vi "blackfly camera capture v2.1 - laser pointer.vi"() -> ()   [LabVIEW 2020]
uses:
  <vilib>/userDefined/High Color/IMAQdx.ctl
  <vilib>/vision/driver/IMAQdx.llb/IMAQdx Acquisition Mode.ctl
  <vilib>/vision/driver/IMAQdx.llb/IMAQdx Buffer Number Mode.ctl
  <vilib>/DAQmx/write.llb/DAQmx Write (Analog Wfm 1Chan NSamp).vi
  <vilib>/DAQmx/read.llb/DAQmx Read (Analog DBL 1Chan 1Samp).vi
  <extravilib>/ChannelInstances/Stream-a[.](u8)/Read With Abort.vi
  <extravilib>/ChannelInstances/Stream-a[.](u8)/Write With Abort.vi
  <extravilib>/ChannelInstances/Stream-a[.](u8)/EndpointRead.vi
  <extravilib>/ChannelInstances/Stream-a[.](u8)/Endpoint.vi
  <vilib>/DAQmx/create/channels.llb/DAQmx Create Channel (AO-Voltage-Basic).vi
  <vilib>/DAQmx/configure/timing.llb/DAQmx Timing (Sample Clock).vi
  <vilib>/DAQmx/create/channels.llb/DAQmx Create Channel (AI-Voltage-Basic).vi
  <vilib>/DAQmx/miscellaneous.llb/DAQmx Fill In Error Info.vi
  <extravilib>/ChannelInstances/Stream-a[.](u8)/Instantiate.vi
  <extravilib>/ChannelInstances/Stream-a[.](u8)/)Channel.vi
  <resource>/ChannelSupport/_ChannelSupport/WaitIfNeeded.vi
  <vilib>/vision/driver/NI_Vision_Acquisition_Software.lvlib
  <resource>/objmgr/imaqdx.rc
  <vilib>/Analysis/NI_AALPro.lvlib
  <vilib>/Analysis/NI_AALBase.lvlib
  <instrlib>/Tektronix AFG 1000 Series/Tektronix AFG 1000 Series.lvlib
  <extravilib>/ChannelInstances/Stream-a[.](u8).lvlib
  <resource>/objmgr/daqmx.rc
  <vilib>/measure/NI_MABase.lvlib
  Lab View projects/Tektronix DC Power Supply Interface/Tektronix PWS4XXX Series/Tektronix PWS4XXX Series.lvlib
panel:
  in  "prog 2 v arr":dbl[](array[numeric])=[0.0, 1.2, 1.4, 1.6, 1.6, 1.4, 1.2]
  in  "v time p2":dbl=20.0
  out "prog 2 step":dbl
  in  "Program 2":bool
  in  "move on click":bool
  in  "de-init time":dbl=10.0
  in  "v time":dbl=40.0
  in  "init time":dbl=10.0
  out "prog1 step":dbl
  in  "Program 1":bool
  in  "AOBD MIN":dbl=2.4
  in  "AOBD MAX":dbl=4.0
  out "Global Rectangle":i32[](array[numeric])
  out "Image":T1(plugin-control)
  in  "AOBD GO":bool
  in  "AOBD W":dbl=0.001 min=0.0 max=3.0 step=0.1
  in  "AOBD Y":dbl=3.2
  in  "AOBD X":dbl=3.2
  in  "Partial P. Ref.":string(combo)="70 nm Au"
  out "All data log refnum":refnum<file>
  out "laer volts refnum":refnum<file>
  out "Laser mW renum":refnum<file>
  in  "V limit":dbl=3.0
  in  "Laser On/Off":bool
  in  "Current (A)":dbl
  in  "Laser Volts (V)":dbl=0.3 min=0.0 max=5.0 step=0.1
  out "nm/pixel\n(binned)":dbl
  in  "nm/pixel\n(native)":dbl=67.5
  in  "2x binning":bool=TRUE
  out "offsety":dbl
  out "offsetx":dbl
  in  "Camera pixels":string(combo)="256"
  in  "Ratio Buffer Size":i32=20
  in  "Dynamic Range":dbl=0.03 step=0.01
  in  "Ratiometric?":bool
  in  "Tab Control - Record Save":enum32{"Page 1", "Page 2"}(tab)
  out "red":bool
  out "yellow":bool
  in  "Experiment Name":string="test code"
  in  "Experiment Notes":string="8ul NaH2PO4\n8ul sample\n75nm Au Partial Reflector"
  in  "SAVE RAW IMAGE":bool
  in  "RECORD / STOP VIDEO":bool
  in  "Copy Notes To Log":bool
  in  "FOV (um)":dbl
  out "second":i32
  out "minute":i32
  out "recorded fps":dbl
  out "Y":dbl
  out "X":dbl
  in  "Base Path":path=path "C:/Users/Matt/Desktop/ISCAT EXPERIMENTS"
  out "Date":string
  out "Record Step":u8
  out "record start time":dbl format="%_19f"
  in  "Save Raw Binary":bool=TRUE
  in  "Save Feed Binary":bool
  in  "Clear Log":bool
  in  "Save Experiment Log":bool
  out "Experiment Log":string
  out "Camera Status":string
  in  "Refresh":bool
  out "copy buffer":bool
  out "noise":dbl format="%0.7f"
  in  "get noise":bool
  in  "Paste Buffer":bool
  in  "Copy Buffer":bool
  out "XY Graph 2":cluster{dbl[], "element":u8[]}(graph)
  in  "V":dbl(slide) scale=-1.5..1.5
  in  "signal type":T2(ring)
  in  "Laser Zoom Level":T3(radio)=enum."Radio Selection 3"
  in  "Record\nVoltage?":bool=TRUE
  out "EPD Voltage":dbl format="%0.2f"
  out "Waveform Graph":waveform(dbl)(graph)
  in  "Amplitude (V)":dbl=1.0
  in  "Frequency (hz)":dbl=0.1
  in  "Offset (V)":dbl
  in  "phase (°)":dbl
  in  "EPD Voltage set":dbl=1.2 step=0.1
  in  "AC":bool
  in  "EPD-DC Power":bool
  out "Main Intensity":dbl[][](graph)
  in  "Camera Zoom Level - DEPRECATED":T4(radio)
  in  "conc.":string
  in  "set sample name":bool
  in  "pH":string="7"
  in  "Size":string="50"
  in  "Material":string(combo)="PS"
  in  "Coverslip":string(combo)="ITO dc 70-100 ohm - no bb"
  in  "Laser Current":dbl=500.0
  in  "Laser Power":dbl=5.0
  out "Laser Temp":u8(slide) scale=20.0..50.0
  out "PSU Temp":u8(slide) scale=20.0..50.0
  out "Laser PSUType":u16(ring)=3 items=["FPU", "MPC6000", "MPC3000", "SMD12"]
  out "Laser COM Port":refnum<visa-resource-name>="COM6"
  in  "Set Laser Power":bool
  in  "Set Power (mW)":dbl=150.0
  in  "Green Laser":bool
  in  "stop":bool
  out "Histogram Graph 2":T5(graph)
  in  "Extras":T6(tab)
  out "live print map":dbl[][](graph)
  out "resampled image":u8[][](graph)
  out "aobd y":dbl
  out "aobd x":dbl
  out "volts on?":bool
  out "applied volts":dbl
  in  "reset print image button":bool
  in  "print image button":bool
  out "timer value":dbl
  out "initialized array":dbl[][](array[numeric])
  out "x":i32
  out "y":i32
  out "pixel value":dbl
  in  "exposure time":dbl(slide)=1000.0 scale=0.0..10000.0
  in  "aobd max":dbl=4.2
  in  "aobd min":dbl=2.2
  in  "set volts":dbl=1.0
  in  "output resolution":dbl=4.0
  in  "load image button":bool
  out "Raw binfile refnum":refnum<file>
  out "Text File refnum":refnum<file>
  out "Feed binfile refnum":refnum<file>
  out "text file path":string
  out "feed file path":string
  out "raw file path":string
  out "image file path":string
  out "Laser Status Update Timer":u32
  out "fps 2":dbl(graph)
  out "raw feed":u8[][](graph)
  out "t1":dbl format="%_19f"
  out "t2":dbl format="%_19f"
  out "rt":dbl
  out "rt 2":dbl
  out "zoom array":i32[](array[numeric])
  out "FOV array":i32[](array[numeric])
  out "FunGen Amp Array":dbl[](array[numeric])
  out "EPD Voltage Log refnum":refnum<file>
  out "Voltage Log file Path":string
  in  "Tab Control 3":T7(tab)
  out "frame rate warning":bool
  in  "900 fps":bool
  in  "600 fps":bool
  in  "500 fps":bool
  in  "200 fps":bool
  out "Gain Warning":bool
  out "sync exp warning":bool
  in  "Exposure Time (us)":dbl(slide)=676.6766570605188 scale=4.4..10000.0
  in  "Frame Rate (hz)":dbl(slide) scale=0.0..1000.0
  in  "Gain (dB)":dbl(slide) scale=0.0..47.9
  out "frame rate":dbl
  out "exp time":dbl=1.0
  out "Gain (dB)":dbl
  out "sync exp":dbl
  out "Ratio Stack 1":dbl[][](array[numeric])
  out "Boolean":bool
  out "Ratio Stack 2":dbl[][](array[numeric])
  out "Boolean 2":bool
  out "max value":dbl
  out "min value":dbl
  out "Histogram Graph":T5(graph)
  out "loading ratiometric":dbl
  out "loading ratiometric stack":bool
  out "queue2 save":cluster{dbl[][]}[](array[cluster])
  out "# elements in queue":i32
  out "Numeric":i32
  out "# elements in queue 2":i32
  out "size(s)":i32
  out "queue1 save":cluster{dbl[][]}[](array[cluster])
  in  "get camera info":bool
  out "AcquisitionMode":dbl
  out "AcquisitionFrameRateEnable":dbl
  out "ExposureMode":dbl
  out "Line Selector":dbl
  out "Line Mode":dbl
  out "Line Inverter":dbl
  out "Gain Auto":dbl
  out "binning vertical":dbl
  out "binning horizontal":dbl
  out "height":dbl
  out "width":dbl
  in  "Auto Exposure":string(combo)
  in  "Auto Framerate":string(combo)
  in  "Auto Gain":string(combo)
  in  "Manual Framerate Enabled?":bool
  out "Buffer Number Out":u32
  out "bg array":dbl[][](array[numeric])
  in  "bg array sum":dbl[][](array[numeric])
  out "bg timer":u32
  out "n bg frames":i32
  out "bg countdown":dbl format="%#_2f"
  in  "acquire bg":bool
  in  "apply bg removal":bool
  out "acquiring bg":bool
  # "was 74"
  # "was 37"
  # "nm"
  # "send to NI voltage card"
  # "send to function generator"
  # "I should just remove this \"feature\""
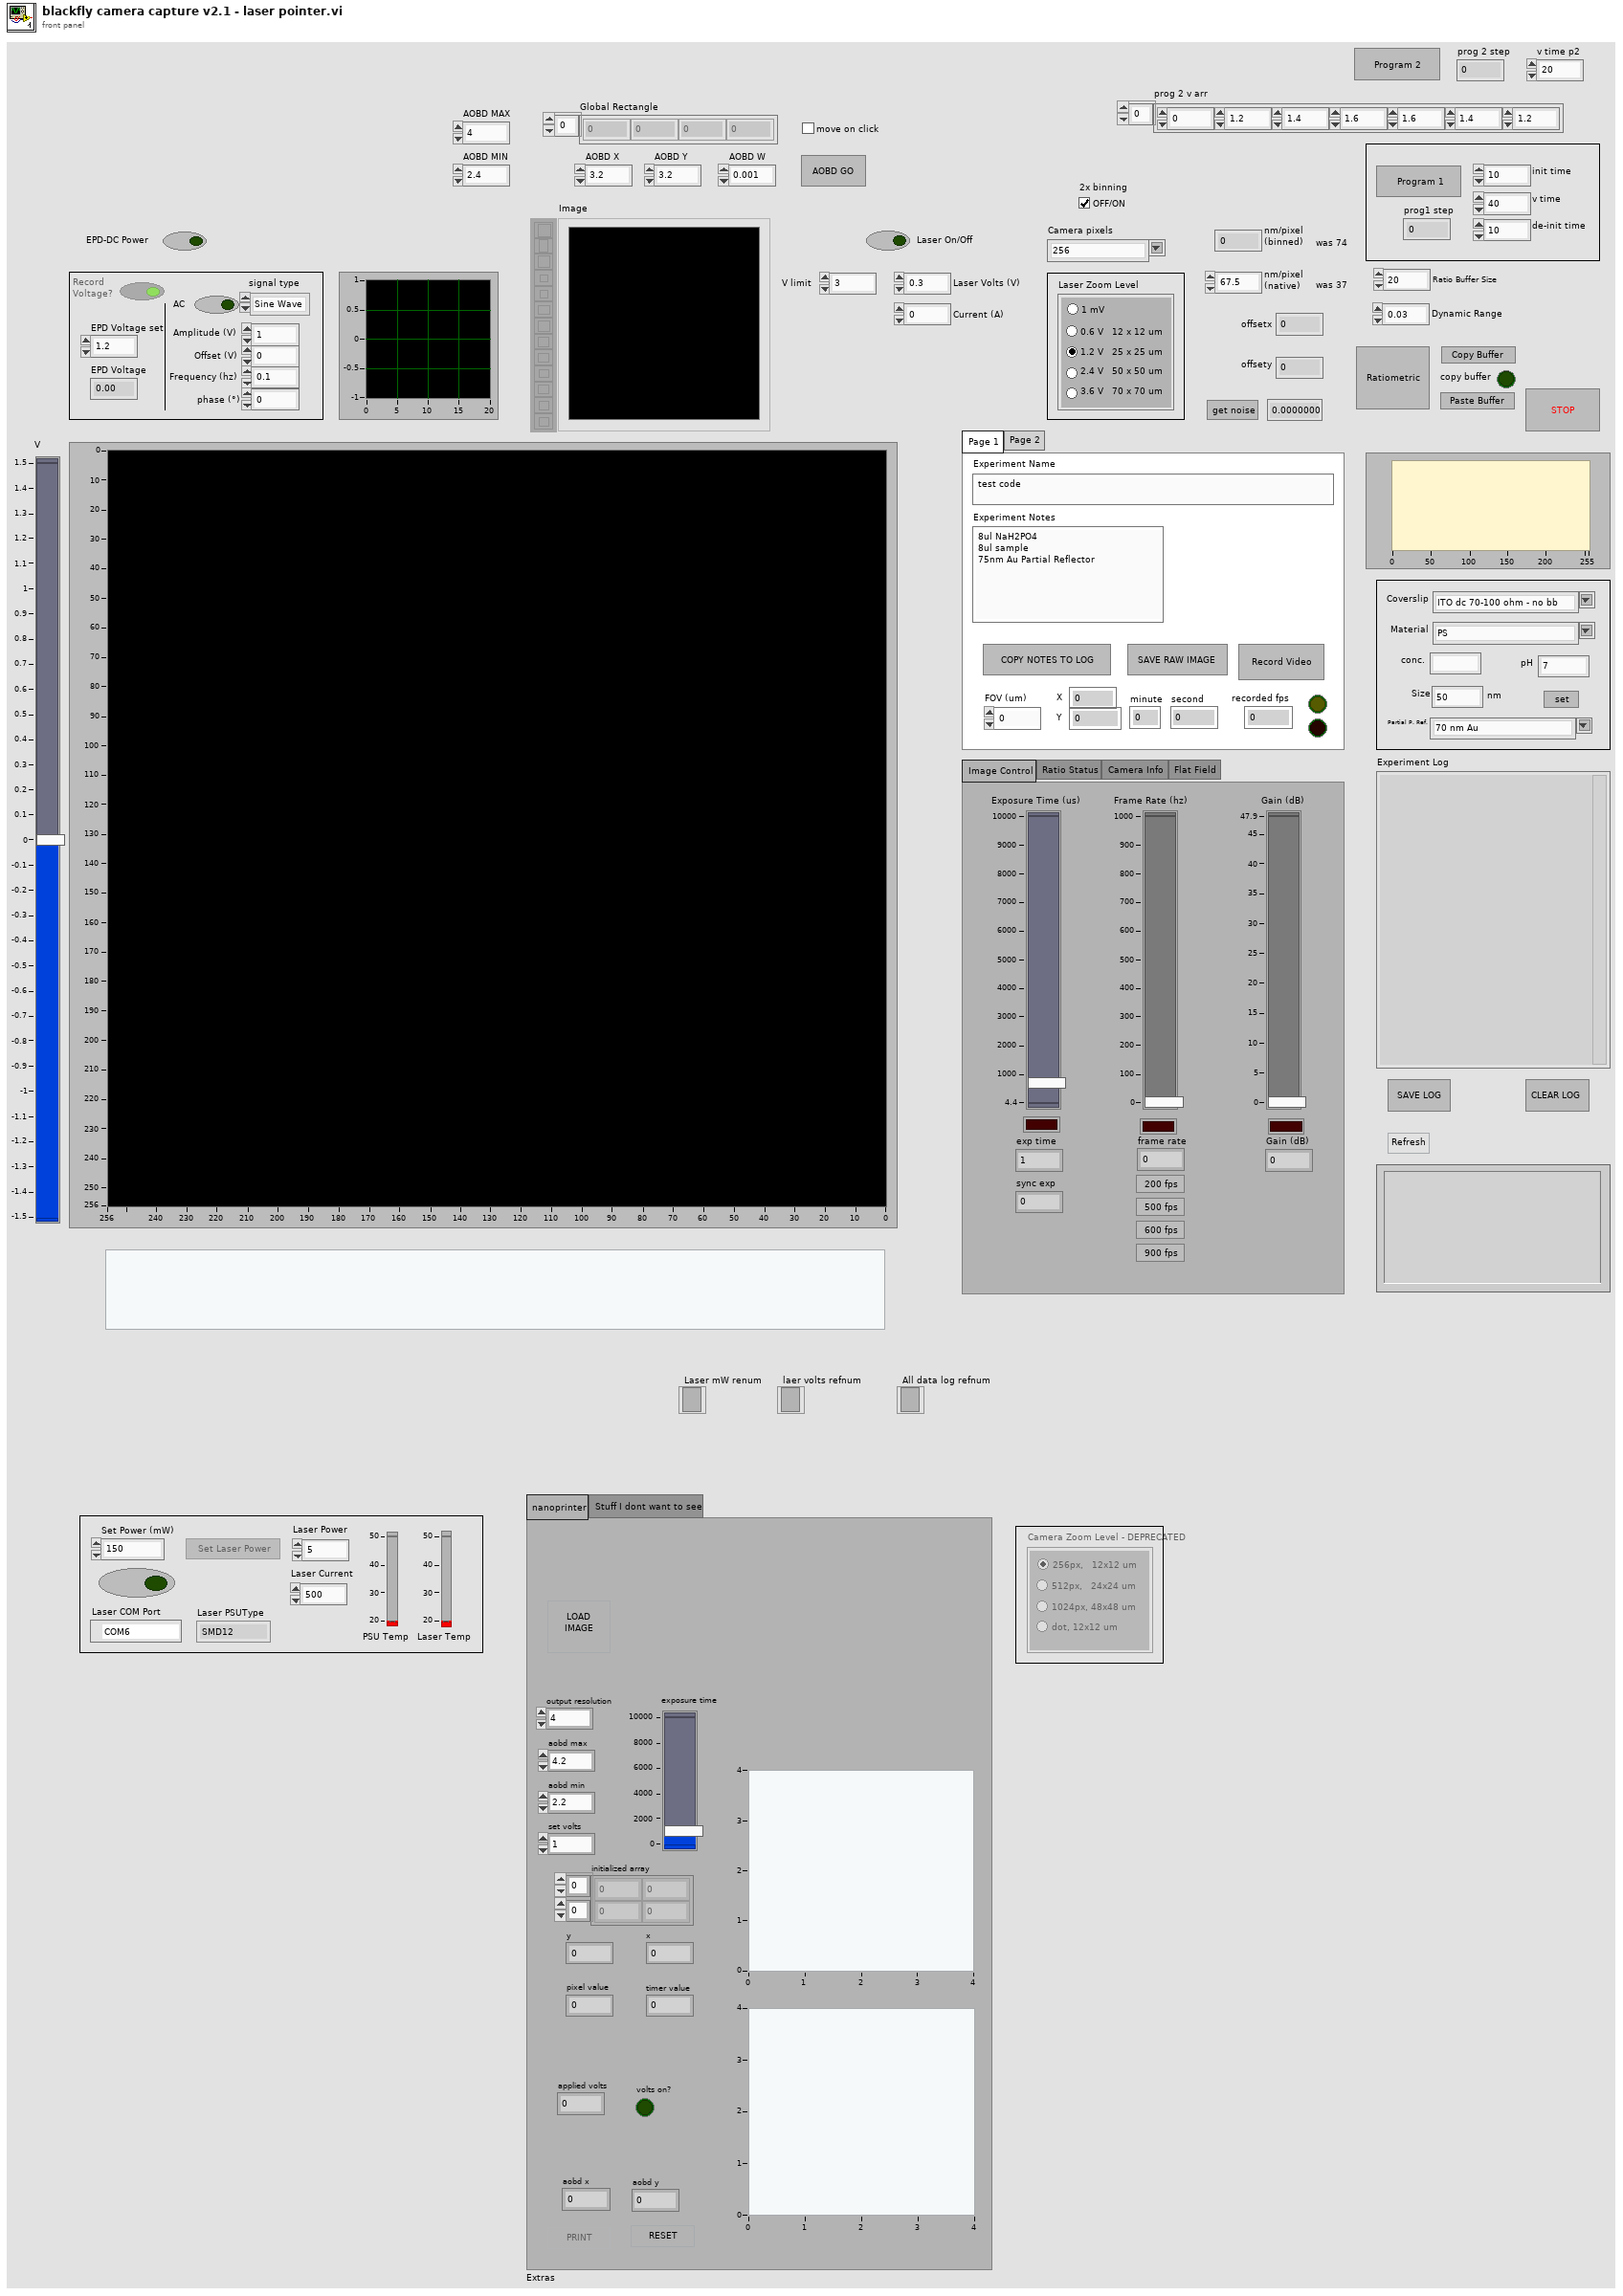
[diagram p1: front panel]
types:
  T1 = typedef "IMAQ Image.ctl" = refnum<image>
  T2 = enum16{"Sine Wave", "Triangle Wave", "Square Wave", "Sawtooth Wave"}
  T3 = enum32{"Radio Selection 1", "Radio Selection 2", "Radio Selection 3", "Radio Selection 4", "Radio Selection 5"}
  T4 = enum32{"256px,   12x12 um", "512px,   24x24 um", "1024px, 48x48 um", "dot, 12x12 um"}
  T5 = cluster{"X Values":dbl[], "Histogram: h(x)":i32[]}
  T6 = enum32{"nanoprinter", "Stuff I dont want to see"}
  T7 = enum32{"Image Control", "Ratio Status", "Camera Info", "Flat Field"}
  T8 = typedef "IMAQdx.ctl" = refnum<k21>
  T9 = enum8{"Enabled", "Disabled", "Disabled and Grayed Out"}
  T10 = typedef "NI_Vision_Acquisition_Software.lvlib/IMAQdx Acquisition Mode.ctl" = enum32{"One Shot", "Continuous"}
  T11 = typedef "NI_Vision_Acquisition_Software.lvlib/IMAQdx Buffer Number Mode.ctl" = enum32{"Next", "Last", "Buffer Number", "Every", "Last New"}
  T12 = cluster{string, "ValueDBL":dbl, string, "ValueDBL":dbl, string, "ValueDBL":dbl, string, "ValueDBL":dbl, "ValueDBL":dbl, "ValueDBL":dbl, "ValueDBL":dbl, "ValueDBL":dbl, "ValueDBL":dbl, "ValueDBL":dbl}
  T13 = cluster{"Global Rectangle":i32[], "Contours":cluster{"Contour Type":u32, "ROI Type":u32, "Points":i32[]}[]}
  T14 = typedef "Stream-a[.](u8).lvlib/)Channel.ctl" = refnum<queue>
  T15 = typedef "LVDateTimeRec.ctl" = cluster{"fractional second":dbl, "second":i32, "minute":i32, "hour":i32, "day of month":i32, "month":i32, "year":i32, "day of week":i32, "day of year":i32, "DST":i32}
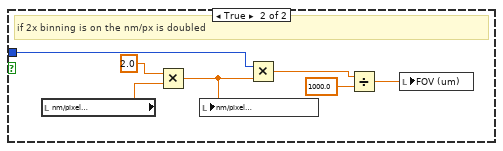
[diagram p2: hidden frame]
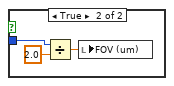
[diagram p3: hidden frame]
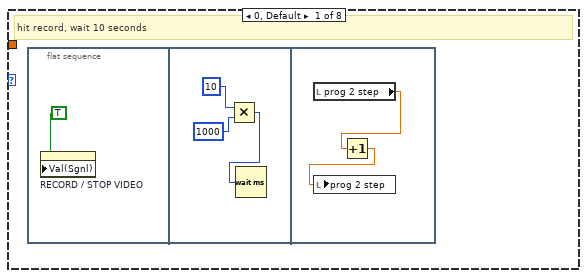
[diagram p11: hidden frame]
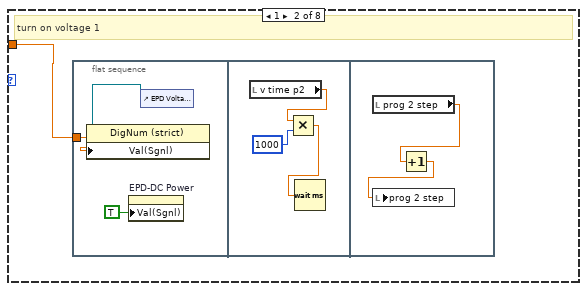
[diagram p12: hidden frame]
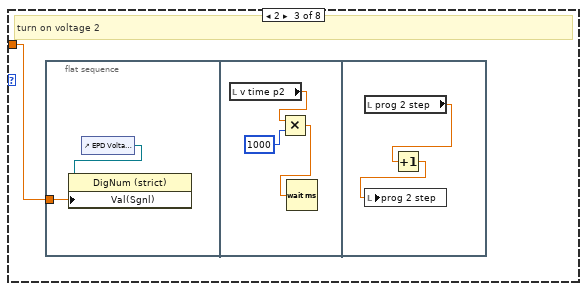
[diagram p13: hidden frame]
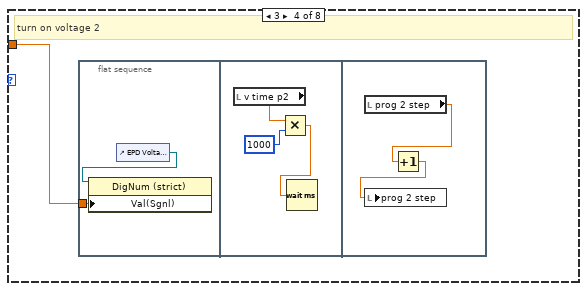
[diagram p14: hidden frame]
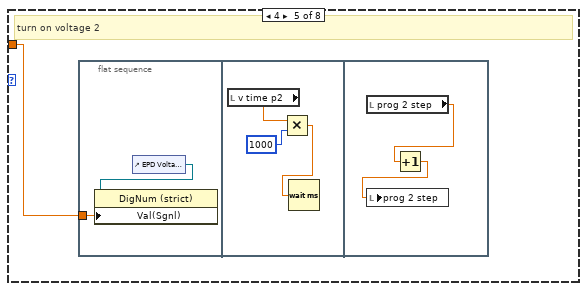
[diagram p15: hidden frame]
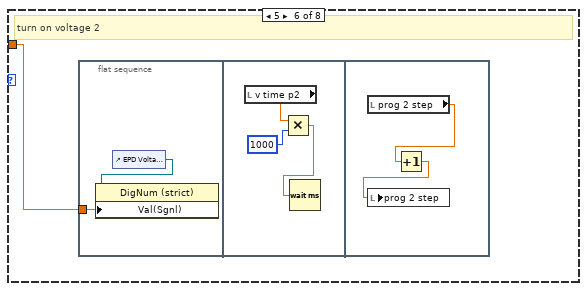
[diagram p16: hidden frame]
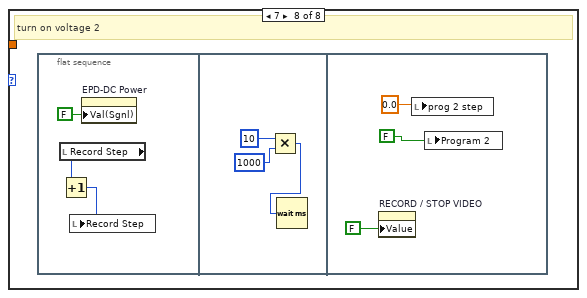
[diagram p17: hidden frame]
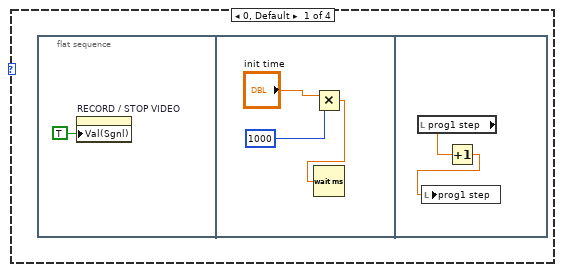
[diagram p19: hidden frame]
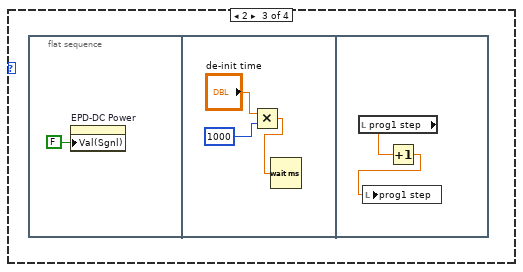
[diagram p20: hidden frame]
diagram:
  n1 = flat-sequence {
    tunnel: [w63] -> w38
    tunnel: [w53] -> w24
    tunnel: [w52] -> w23
    tunnel: [w47] -> w20
    tunnel: [w42] -> w14
    tunnel: [w40] -> w6
    tunnel: [w39] -> w3
    tunnel: w38 -> [w272]
    tunnel: [w275] -> w37
    tunnel: [w272] -> w35
    tunnel: [w273] -> w34
    tunnel: [w259] -> w30
    tunnel: [w258] -> w29
    tunnel: w24 -> [w164]
    tunnel: w23 -> [w163]
    tunnel: [w229] -> w22
    tunnel: w20 -> [w229]
    tunnel: [w197] -> w19
    tunnel: [w196] -> w17
    tunnel: [w195] -> w16
    tunnel: w14 -> [w194]
    tunnel: [w193] -> w13
    tunnel: [w187] -> w11
    tunnel: [w186] -> w10
    tunnel: w6 -> [w72]
    tunnel: [w72] -> w5
    tunnel: w3 -> [w71]
    tunnel: [w71] -> w2
    tunnel: w37 -> [w404]
    tunnel: [w400] -> w36
    tunnel: w35 -> [w400]
    tunnel: w34 -> [w405]
    tunnel: [w403] -> w33
    tunnel: [w402] -> w32
    tunnel: [w406] -> w31
    tunnel: w30 -> [w398]
    tunnel: w29 -> [w397]
    tunnel: [w396] -> w28
    tunnel: [w395] -> w27
    tunnel: [w394] -> w26
    tunnel: [w393] -> w25
    tunnel: w22 -> [w380]
    tunnel: [w399] -> w21
    tunnel: w19 -> [w391]
    tunnel: [w390] -> w18
    tunnel: w17 -> [w389]
    tunnel: w16 -> [w388]
    tunnel: [w387] -> w15
    tunnel: w13 -> [w386]
    tunnel: [w385] -> w12
    tunnel: w11 -> [w384]
    tunnel: w10 -> [w383]
    tunnel: [w382] -> w9
    tunnel: [w381] -> w8
    tunnel: [w379] -> w7
    tunnel: w5 -> [w377]
    tunnel: [w377] -> w4
    tunnel: w2 -> [w376]
    tunnel: [w375] -> w1
    tunnel: w36 -> [w2026]
    tunnel: w33 -> [w2034]
    tunnel: w32 -> [w2027]
    tunnel: w31 -> [w2016]
    tunnel: w28 -> [w2023]
    tunnel: w27 -> [w2022]
    tunnel: w26 -> [w2019]
    tunnel: w25 -> [w2018]
    tunnel: w21 -> [w2015]
    tunnel: w18 -> [w2013]
    tunnel: w15 -> [w2003]
    tunnel: w12 -> [w2002]
    tunnel: w9 -> [w2000]
    tunnel: w8 -> [w1999]
    tunnel: w7 -> [w1991]
    tunnel: w4 -> [w1990]
    tunnel: w1 -> [w1989]
    frame #0 {
      # "Lasertack Laser Controls\n\nTektronix PWS4721 Programmable\nDC Power Supply 0-72V, 1.2A"
      # "FUNCTION GENERATOR FOR ITO EXPERIMENTS"
      # "Function Generator Controls"
      # "BINARY VIDEO SAVING"
      # "Reset Default Controls Upon Start-Up"
      # "Video Feed Circular Buffer Initialization"
      # "MAIN CONTROLS"
      # "Camera Feed Controls"
      # "Initialization 1"
      n2 = control-ref of="This VI"() -> (w58:refnum<vi>)
      n3 = Multiply(x="Ratio Buffer Size", y=2) -> (x*y=w61:i32)
      n4 = Add(x=w61, y=10.0) -> (x+y=w64:dbl)
      n5 = invoke class="VI" method="Default Vals.Reinit All"(reference=w58) -> ()  [unwired: 2 in, 3 out]
      n6 = call <instrlib>:"Initialize.vi"("Reset (True)"=FALSE, "VISA resource name"=refnum<visa-resource-name> "USB0::0x0699::0x0353::2002170::INSTR") -> ("error out"=w42:errorcluster, "VISA resource name out"=w47:refnum<visa-resource-name>)  [unwired: 8 in]
      n7 = for {
        N: w64 -> [_]
        tunnel: [w66] -> w63 mode=indexing
        tunnel: [w65] -> w57
        i -> [w70]
        # "Allocate Buffer Memory"
        n8 = Format Into String(format string="Buffer ID %d", w70) -> (resulting string=w68:string)  [unwired: 2 in, 1 out]
        n9 = call "IMAQ Create"("Border Size"=0, "Image Name"=w68) -> ("New Image"=w66:T1, "error out"=w65:errorcluster)  [unwired: 3 in]
      }
      n10 = call <instrlib>:"Initialize.vi"("VISA resource name"=refnum<visa-resource-name> "USB0::0x0699::0x0394::C010244::INSTR") -> ("error out"=w39:errorcluster, "VISA resource name out"=w40:refnum<visa-resource-name>)  [unwired: 9 in]
      n11 = property on="Main Intensity" class="IntGraph (strict)"("ZScale.Maximum"=255.0 ("Z Scale.Range:Maximum"), "ZScale.Minimum"=0.0 ("Z Scale.Range:Minimum")) -> ()  [unwired: 2 in, 2 out]
      n12 = property on="Main Intensity" class="IntGraph (strict)"("XScale.Minimum"=0.0 ("Z Scale.Range:Maximum"), "YScale.Minimum"=0.0 ("Z Scale.Range:Minimum"), "XScale.Maximum"=512.0 ("Y Scale.Range:Minimum"), "YScale.Maximum"=512.0 ("Y Scale.Range:Minimum")) -> ()  [unwired: 2 in, 2 out]
      n13 = call <vilib>:"IMAQdx Open Camera.vi"("error in"=w57, "Session In"=T8 "blackfly") -> ("error out"=w53:errorcluster, "Session Out"=w52:T8)  [unwired: 8 in]
      "rt" <- 0.0 ("rt")
      "rt 2" <- 0.0 ("rt")
    }
    frame #1 {
      w83 = "\t"
      w81 = "\r\n"
      w80 = 2.0 ("ValueDBL")
      w126 = u32 256 ("Height")
      w127 = u32 256 ("Width")
      w213 = 10123 items=["Finite Samples"=10178, "Continuous Samples"=10123, "Hardware Timed Single Point"=12522] ("sample mode")
      w216 = 10123 items=["Finite Samples"=10178, "Continuous Samples"=10123, "Hardware Timed Single Point"=12522] ("sample mode")
      # "READ VOLTAGE CHANNEL"
      # "ANALOG VOLTAGE OUTPUT CHANNEL"
      # "Initialization 2"
      n14 = local read "Camera Zoom Level - DEPRECATED"() -> (w228:T4)
      n15 = property class="IMAQdx"(reference=w163, error in=w164, "OffsetX"=u32 0, "OffsetY"=u32 0) -> (reference out=w147:T8, error out=w146:errorcluster)
      n16 = disable-structure shown="Disabled" {
        frame Disabled {
          w294 = u16 3 items=["FPU", "MPC6000", "MPC3000", "SMD12"] ("PSUType")
          n17 = Tick Count (ms)() -> (millisecond timer value=→"Laser Status Update Timer":u32)
          "Laser COM Port" <- refnum<visa-resource-name> "COM6" ("LQComm Resource In")
          "Laser PSUType" <- w294
        }
        frame Enabled {
        }
      }
      n18 = disable-structure shown="Disabled" {
        disable-tunnel: _ -> [w343 _]
        disable-tunnel: [w342 _] -> _
        frame Disabled {
          n19 = property class="IMAQdx"(reference=w343, "ActiveAttribute"="CameraAttributes::ImageFormatControl::VideoMode", "ValueDBL"=2.0) -> (reference out=w342:T8)  [unwired: 1 in, 1 out]
        }
        frame Enabled {
        }
      }
      n20 = local read "FOV array"() -> (w239:i32[])
      n21 = local read "Laser Zoom Level"() -> (w143:T3)
      n22 = local read "2x binning"() -> (w79:bool)
      n23 = Build Array(0.75 ("dimension size"), 1.5 ("dimension size"), 3.0 ("dimension size"), 0.001 ("element")) -> (→"FunGen Amp Array":dbl[])
      n24 = Index Array(array=w239, index=w228) -> (element=w78:i32)
      n25 = Build Array(256 ("dimension size"), 512 ("dimension size"), 1024 ("dimension size"), 256 ("element")) -> (→"zoom array":i32[])
      n26 = Build Array(9 ("dimension size"), 18 ("dimension size"), 36 ("dimension size"), 9 ("element")) -> (→"FOV array":i32[])
      n27 = call-poly <vilib>:"DAQmx Create Virtual Channel.vi"("maximum value"=10.0, "minimum value"=-10.0, "physical channels"=tag "Dev1/ao0", "name to assign"="Channel 1 V_out") -> ("task out"=w215:refnum<k21>, "error out"=w190:errorcluster)  [unwired: 10 in]
      n28 = case shown="False" w79 {
        tunnel: w78 -> [w289 w290]
        frame False {
          n29 = local write "FOV (um)"(w289) -> ()
        }
        frame True {
          n30 = Divide(x=w290, y=2.0) -> (x/y=w291:dbl)
          n31 = local write "FOV (um)"(w291) -> ()
        }
      }
      n32 = local read "zoom array"() -> (w238:i32[])
      n33 = flat-sequence "Recall Function Generator Settings" {
        tunnel: [w351] -> w180
        tunnel: w229 -> [w350]
        tunnel: [u32 200 ("milliseconds to wait")] -> w178
        tunnel: w143 -> [w349]
        tunnel: [w348] -> w176
        tunnel: w194 -> [w347]
        tunnel: w180 -> [w355]
        tunnel: [w355] -> w179
        tunnel: w178 -> [w353]
        tunnel: [w353] -> w177
        tunnel: w176 -> [w354]
        tunnel: [w354] -> w175
        tunnel: [w360] -> w185
        tunnel: w179 -> [w359]
        tunnel: w177 -> [w358]
        tunnel: [w358] -> w183
        tunnel: w175 -> [w357]
        tunnel: [w356] -> w182
        tunnel: w185 -> [w365]
        tunnel: [w365] -> w184
        tunnel: w183 -> [w363]
        tunnel: w182 -> [w364]
        tunnel: [w364] -> w181
        tunnel: w184 -> [w368]
        tunnel: w181 -> [w367]
        tunnel: [w366] -> w193
        frame #0 {
          w352 = u16 0 items=["Recall", "Save"] ("Operation (0: Recall)")
          n34 = call <instrlib>:"Recall Save Instrument Settings.vi"("error in (no error)"=w347, "Setup Memory Location (0)"=w349, "Operation (0: Recall)"=w352, "VISA resource name"=w350) -> ("error out"=w348:errorcluster, "VISA resource name out"=w351:refnum<visa-resource-name>)  [unwired: 6 in]
        }
        frame #1 {
          n35 = Wait (ms)(milliseconds to wait=w353) -> ()  [unwired: 1 out]
        }
        frame #2 {
          w361 = u16 1 items=["Channel 1"=1, "Channel2"=2] ("Channel (1: Channel 1)")
          n36 = call <instrlib>:"Enable Output.vi"("Enable Output (T: Enable)"=TRUE, "error in (no error)"=w357, "Channel (1: Channel 1)"=w361, "VISA resource name"=w359) -> ("error out"=w356:errorcluster, "VISA resource name out"=w360:refnum<visa-resource-name>)  [unwired: 6 in]
        }
        frame #3 {
          n37 = Wait (ms)(milliseconds to wait=w363) -> ()  [unwired: 1 out]
        }
        frame #4 {
          w369 = u16 2 items=["Channel 1"=1, "Channel2"=2] ("Channel (1: Channel 1)")
          n38 = call <instrlib>:"Enable Output.vi"("Enable Output (T: Enable)"=TRUE, "error in (no error)"=w367, "Channel (1: Channel 1)"=w369, "VISA resource name"=w368) -> ("error out"=w366:errorcluster)  [unwired: 6 in, 1 out]
        }
      }
      n39 = call-poly <vilib>:"DAQmx Create Virtual Channel.vi"("physical channels"=tag "Dev1/_ao0_vs_aognd") -> ("task out"=w214:refnum<k21>, "error out"=w192:errorcluster)  [unwired: 13 in]
      n40 = Get Date/Time In Seconds() -> (seconds since 1Jan1904=w270:timestamp)
      n41 = property on="RECORD / STOP VIDEO" class="Bool (strict)"("BoolText.Text"="Record Video" ("Boolean Text.Text"), "BoolText.FontBold"=FALSE ("Boolean Text.Font:Bold")) -> ()  [unwired: 2 in, 2 out]
      n42 = Format Date/Time String(time format string (%c)="%Y-%m-%d-", seconds (now)=w270) -> (date/time string=→"Date":string)  [unwired: 1 in]
      n43 = Index Array(array=w238, index=w228) -> (element=w227:i32)
      n44 = call-poly <vilib>:"DAQmx Timing.vi"("task/channels in"=w214, "sample mode"=w213, "rate"=100000.0, "source"=tag "OnboardClock", "error in"=w192) -> ("task out"=w210:refnum<k21>, "error out"=w191:errorcluster)  [unwired: 9 in]
      n45 = Subtract(x=1224, y=w227) -> (x-y=w232:i32)
      n46 = Subtract(x=1024, y=w227) -> (x-y=w233:i32)
      n47 = call-poly <vilib>:"DAQmx Timing.vi"("task/channels in"=w215, "sample mode"=w216, "rate"=100000.0, "source"=tag "OnboardClock", "error in"=w190) -> ("task out"=w223:refnum<k21>, "error out"=w189:errorcluster)  [unwired: 9 in]
      n48 = Divide(x=w232, y=2) -> (x/y=w231:dbl)
      n49 = Divide(x=w233, y=2) -> (x/y=w230:dbl)
      n50 = disable-structure shown="Disabled" {
        disable-tunnel: w231 -> [w298 _]
        disable-tunnel: w230 -> [w297 _]
        disable-tunnel: w227 -> [w296 _]
        frame Disabled {
          n51 = property class="IMAQdx"("OffsetX"=u32 0, "OffsetY"=u32 0) -> (reference out=w299:T8)  [unwired: 2 in, 1 out]
          n52 = property class="IMAQdx"(reference=w299, "Width"=w296, "Height"=w296, "OffsetX"=w298, "OffsetY"=w297) -> ()  [unwired: 1 in, 2 out]
        }
        frame Enabled {
        }
      }
      n53 = property class="DAQmx Timing"(reference=w223) -> (reference out=w200:refnum<k21>, "SampClk.Rate"=w199:dbl)  [unwired: 1 in, 1 out]
      n54 = property class="IMAQdx"(reference=w147, error in=w146, "ActiveAttribute"="CameraAttributes::AcquisitionControl::AcquisitionFrameRateEnable", "ValueDBL"=1.0, "ActiveAttribute"="CameraAttributes::AcquisitionControl::AcquisitionFrameRate", "ValueDBL"=24.0, "ActiveAttribute"="CameraAttributes::AcquisitionControl::AcquisitionMode", "ValueDBL"=0.0, "ActiveAttribute"="CameraAttributes::ImageFormatControl::BinningHorizontal", "ValueDBL"=w80, "ActiveAttribute"="CameraAttributes::ImageFormatControl::BinningVertical", "ValueDBL"=w80, "ActiveAttribute"="CameraAttributes::AnalogControl::GainAuto", "ValueDBL"=0.0, "ActiveAttribute"="CameraAttributes::AnalogControl::Gain", "ValueDBL"=0.0, "ActiveAttribute"="CameraAttributes::AcquisitionControl::ExposureAuto", "ValueDBL"=0.0, "ActiveAttribute"="CameraAttributes::AcquisitionControl::ExposureTime", "ValueDBL"=1000.0) -> (reference out=w120:T8, error out=w119:errorcluster)
      n55 = property class="DAQmx Timing" props=["SampClk.Rate"](reference=w210) -> (reference out=w198:refnum<k21>)  [unwired: 1 in, 2 out]
      n56 = local read "Camera pixels"() -> (w74:string)
      n57 = local read "2x binning"() -> (w73:bool)
      n58 = property class="IMAQdx"(reference=w120, error in=w119, "ActiveAttribute"="CameraAttributes::DigitalIOControl::LineSelector", "ValueDBL"=2.0, "ActiveAttribute"="CameraAttributes::DigitalIOControl::LineMode", "ValueDBL"=1.0, "ActiveAttribute"="CameraAttributes::DigitalIOControl::LineInverter", "ValueDBL"=1.0) -> (reference out=w118:T8, error out=w117:errorcluster)
      n59 = Bundle By Name(cluster=cluster{"Fs":dbl, "#s":dbl} {"Fs"=1000.0, "#s"=1000.0} ("sampling info"), "#s"=1000000.0, "Fs"=w199) -> (w196:cluster{"Fs":dbl, "#s":dbl})
      n60 = Decimal String To Number(string=w74) -> (number=w75:i32)  [unwired: 2 in, 1 out]
      n61 = call "SUBVI_get_pixel_sensor_offset.vi"("vertical binning"=w80, "y dim"=w126, "horizontal binning"=w80, "x dim"=w127, "max height"=1100.0, "max width"=1600.0) -> ("y offset"=w76:dbl, "x offset"=w77:dbl)  [unwired: 4 in]
      n62 = case "Calculate FOV" shown="False" w73 {
        tunnel: w75 -> [w278 w282]
        frame False {
          # "If 2x binning is off then native nm/px = binned nm/px"
          n63 = local read "nm/pixel\n(native)"() -> (w277:dbl)
          n64 = local write "nm/pixel\n(binned)"(w277) -> ()
          n65 = Multiply(x=w278, y=w277) -> (x*y=w280:dbl)
          n66 = Divide(x=w280, y=1000.0) -> (x/y=w281:dbl)
          n67 = local write "FOV (um)"(w281) -> ()
        }
        frame True {
          # "if 2x binning is on the nm/px is doubled"
          n68 = local read "nm/pixel\n(native)"() -> (w286:dbl)
          n69 = Multiply(x=2.0 ("y"), y=w286) -> (x*y=w285:dbl)
          n70 = local write "nm/pixel\n(binned)"(w285) -> ()
          n71 = Multiply(x=w282, y=w285) -> (x*y=w287:dbl)
          n72 = Divide(x=w287, y=1000.0) -> (x/y=w288:dbl)
          n73 = local write "FOV (um)"(w288) -> ()
        }
      }
      n74 = property on="Main Intensity" class="IntGraph (strict)"("XScale.Minimum"=0.0 ("X Scale.Range:Minimum"), "YScale.Minimum"=0.0 ("Y Scale.Range:Minimum"), "XScale.Maximum"=w127, "YScale.Maximum"=w126) -> ()  [unwired: 2 in, 2 out]
      n75 = local write "Y"(w126) -> ()
      n76 = local write "X"(w127) -> ()
      n77 = property class="IMAQdx"(reference=w118, error in=w117, "Width"=w127, "Height"=w126, "OffsetX"=w77, "OffsetY"=w76) -> (reference out=w149:T8, error out=w148:errorcluster)
      n78 = call <vilib>:"Basic Function Generator.vi"("offset"=0.0, "sampling info"=w196, "signal type"=T2."Triangle Wave", "amplitude"=0.0, "frequency"=0.0) -> ("signal out"=w203:waveform(dbl))  [unwired: 4 in, 2 out]
      n79 = disable-structure shown="Disabled" {
        frame Disabled {
          n80 = local read "Laser COM Port"() -> (w372:refnum<visa-resource-name>)
          n81 = local read "Laser PSUType"() -> (w371:u16)
          n82 = call "TurnOFF.vi"("PSUType"=w371, "LQCommResourceIn"=w372) -> ()  [unwired: 1 in, 3 out]
        }
        frame Enabled {
        }
      }
      n83 = local read "Ratio Buffer Size"() -> (w262:i32)
      n84 = property on="print image button" class="Bool (strict)"("DisabledEnum"=T9."Disabled and Grayed Out" ("Disabled")) -> ()  [unwired: 2 in, 2 out]
      n85 = call-poly <vilib>:"DAQmx Write.vi"("task/channels in"=w200, "data"=w203, "error in"=w189) -> ("task out"=w204:refnum<k21>, "error out"=w188:errorcluster)  [unwired: 10 in, 1 out]
      n86 = local write "offsetx"(w77) -> ()
      n87 = local write "offsety"(w76) -> ()
      n88 = call <vilib>:"DAQmx Start Task.vi"("task/channels in"=w198, "error in"=w191) -> ("task out"=w197:refnum<k21>, "error out"=w186:errorcluster)  [unwired: 12 in]
      n89 = call <vilib>:"IMAQdx Configure Ring Acquisition.vi"("Mode"=IMAQdx_Acquisition_Mode."Continuous", "error in"=w148, "Images"=w272, "Session In"=w149) -> ("error out"=w274:errorcluster, "Session Out"=w173:T8)  [unwired: 5 in, 1 out]
      n90 = disable-structure shown="Disabled" {
        disable-tunnel: [w304 _] -> _
        disable-tunnel: [w303 _] -> _
        disable-tunnel: w173 -> [w302 _]
        frame Disabled {
          # "GET CAMERA INFO AND UPDATE CAMERA STATUS INFO"
          n91 = property class="IMAQdx" props=["ActiveAttribute", "ValueDBL", "ActiveAttribute", "ValueDBL", "ActiveAttribute", "ValueDBL", "ActiveAttribute", "ValueBool", "ActiveAttribute", "ValueDBL", "ActiveAttribute", "ValueDBL", "ActiveAttribute", "ValueDBL", "ActiveAttribute", "ValueDBL", "ActiveAttribute", "ValueDBL", "ActiveAttribute", "ValueDBL", "ActiveAttribute", "ValueDBL", "ActiveAttribute", "ValueDBL", "ActiveAttribute", "ValueDBL", "ActiveAttribute", "ValueDBL", "ActiveAttribute", "ValueDBL"](reference=w302, "ActiveAttribute"="CameraAttributes::AcquisitionControl::ExposureAuto", "ActiveAttribute"="CameraAttributes::AcquisitionControl::ExposureTime", "ActiveAttribute"="CameraAttributes::AcquisitionControl::AcquisitionFrameRateAuto", "ActiveAttribute"="CameraAttributes::AcquisitionControl::AcquisitionFrameRateEnabled", "ActiveAttribute"="CameraAttributes::AcquisitionControl::AcquisitionFrameRate", "ActiveAttribute"="CameraAttributes::AnalogControl::GainAuto", "ActiveAttribute"="CameraAttributes::AnalogControl::Gain", "ActiveAttribute"="CameraAttributes::ImageFormatControl::VideoMode", "ActiveAttribute"="CameraAttributes::ImageFormatControl::Width", "ActiveAttribute"="CameraAttributes::ImageFormatControl::Height", "ActiveAttribute"="CameraAttributes::ImageFormatControl::OffsetX", "ActiveAttribute"="CameraAttributes::ImageFormatControl::OffsetY", "ActiveAttribute"="CameraAttributes::ImageFormatControl::BinningHorizontal", "ActiveAttribute"="CameraAttributes::ImageFormatControl::BinningVertical", "ActiveAttribute"="CameraAttributes::ImageFormatControl::PixelSize") -> ("ValueDBL"=w317:dbl, "ValueDBL"=w316:dbl, "ValueDBL"=w315:dbl, "ValueDBL"=w314:dbl, "ValueDBL"=w313:dbl, "ValueDBL"=w312:dbl, "ValueDBL"=w311:dbl, "ValueDBL"=w304:dbl, "ValueDBL"=w303:dbl, "ValueDBL"=w310:dbl, "ValueDBL"=w309:dbl, "ValueDBL"=w308:dbl, "ValueDBL"=w307:dbl, "ValueDBL"=w305:dbl)  [unwired: 1 in, 3 out]
          n92 = Number To Decimal String(number=w317, width (-)=i16 1) -> (decimal integer string=w325:string)
          n93 = Number To Decimal String(number=w315, width (-)=i16 1) -> (decimal integer string=w326:string)
          n94 = Number To Decimal String(number=w313, width (-)=i16 1) -> (decimal integer string=w327:string)
          n95 = Number To Decimal String(number=w311, width (-)=i16 1) -> (decimal integer string=w322:string)
          n96 = local write "Auto Framerate"(w326) -> ()
          n97 = local write "Auto Gain"(w327) -> ()
          n98 = local write "Auto Exposure"(w325) -> ()
          n99 = Bundle(w325, "ValueDBL"=w316, w326, "ValueDBL"=w314, w327, "ValueDBL"=w312, w322, "ValueDBL"=w304, "ValueDBL"=w303, "ValueDBL"=w310, "ValueDBL"=w309, "ValueDBL"=w308, "ValueDBL"=w307, "ValueDBL"=w305) -> (w323:T12)  [unwired: 1 in]
          n100 = local write "X"(w304) -> ()
          n101 = local write "Y"(w303) -> ()
          n102 = call "SUBVI_blackfly_format_info.vi"("Cluster"=w323) -> ("String"=w324:string)
          n103 = local write "Exposure Time (us)"(w316) -> ()
          n104 = local write "Frame Rate (hz)"(w314) -> ()
          n105 = local write "Gain (dB)"(w312) -> ()
          n106 = local write "Camera Status"(w324) -> ()
        }
        frame Enabled {
        }
      }
      n107 = property class="IMAQdx"(reference=w173, "ActiveAttribute"="CameraAttributes::AcquisitionControl::ExposureTime", "ActiveAttribute"="CameraAttributes::AcquisitionControl::AcquisitionFrameRate", "ActiveAttribute"="CameraAttributes::ImageFormatControl::Width", "ActiveAttribute"="CameraAttributes::ImageFormatControl::Height", "ActiveAttribute"="CameraAttributes::ImageFormatControl::OffsetX", "ActiveAttribute"="CameraAttributes::ImageFormatControl::OffsetY", "ActiveAttribute"="CameraAttributes::ImageFormatControl::BinningHorizontal", "ActiveAttribute"="CameraAttributes::ImageFormatControl::BinningVertical", "ActiveAttribute"="CameraAttributes::AnalogControl::GainAuto", "ActiveAttribute"="CameraAttributes::AnalogControl::Gain", "ActiveAttribute"="CameraAttributes::AcquisitionControl::AcquisitionMode", "ActiveAttribute"="CameraAttributes::AcquisitionControl::AcquisitionFrameRateEnable", "ActiveAttribute"="CameraAttributes::AcquisitionControl::ExposureMode", "ActiveAttribute"="CameraAttributes::DigitalIOControl::LineSelector", "ActiveAttribute"="CameraAttributes::DigitalIOControl::LineMode", "ActiveAttribute"="CameraAttributes::DigitalIOControl::LineInverter") -> ("ValueDBL"=w105:dbl, "ValueDBL"=w104:dbl, "ValueDBL"=w103:dbl, "ValueDBL"=w102:dbl, "ValueDBL"=w101:dbl, "ValueDBL"=w100:dbl, "ValueDBL"=w99:dbl, "ValueDBL"=w98:dbl, "ValueDBL"=→"Gain Auto":dbl, "ValueDBL"=→"Gain (dB)":dbl, "ValueDBL"=→"AcquisitionMode":dbl, "ValueDBL"=→"AcquisitionFrameRateEnable":dbl, "ValueDBL"=→"ExposureMode":dbl, "ValueDBL"=→"Line Selector":dbl, "ValueDBL"=→"Line Mode":dbl, "ValueDBL"=→"Line Inverter":dbl)  [unwired: 1 in, 2 out]
      "exp time" <- w105
      "frame rate" <- w104
      "width" <- w103
      "height" <- w102
      "offsetx" <- w101
      "offsety" <- w100
      "binning horizontal" <- w99
      "binning vertical" <- w98
      n108 = Number To Decimal String(number=w104) -> (decimal integer string=w95:string)  [unwired: 1 in]
      n109 = Number To Decimal String(number=w105) -> (decimal integer string=w97:string)  [unwired: 1 in]
      n110 = Number To Decimal String(number=w103) -> (decimal integer string=w93:string)  [unwired: 1 in]
      n111 = Number To Decimal String(number=w102) -> (decimal integer string=w88:string)  [unwired: 1 in]
      n112 = Number To Decimal String(number=w101) -> (decimal integer string=w87:string)  [unwired: 1 in]
      n113 = Number To Decimal String(number=w100) -> (decimal integer string=w86:string)  [unwired: 1 in]
      n114 = Number To Decimal String(number=w98) -> (decimal integer string=w82:string)  [unwired: 1 in]
      n115 = Number To Decimal String(number=w99) -> (decimal integer string=w85:string)  [unwired: 1 in]
      n116 = Divide(x=1000000.0, y=w104) -> (x/y=→"sync exp":dbl)
      n117 = Initialize Array(0.0 ("element"), w102, w103) -> (w266:dbl[][])
      n118 = Initialize Array(0.0 ("element"), w102, w103) -> (→"Ratio Stack 2":dbl[][])
      n119 = Initialize Array(0.0 ("element"), w102, w103) -> (w265:dbl[][])
      n120 = Initialize Array(0.0 ("element"), w102, w103) -> (→"Ratio Stack 1":dbl[][])
      n121 = call <vilib>:"DAQmx Start Task.vi"("task/channels in"=w204, "error in"=w188) -> ("task out"=w195:refnum<k21>, "error out"=w187:errorcluster)  [unwired: 12 in]
      n122 = Obtain Queue(max queue size (-1, unlimited)=w262, name (unnamed)="front", element data type=w266) -> (queue out=w259:refnum<queue>)  [unwired: 2 in, 2 out]
      n123 = Concatenate Strings("Exposure Time (us):" ("string"), w83, w97, w81, "Frame Rate (fps):" ("string"), w83, w95, w81, "Width (px):" ("string"), w83, w93, w81, "Height (px):" ("string"), w83, w88, w81, "Offset X (px):" ("string"), w83, w87, w81, "Offset Y (px):" ("string"), w83, w86, w81, "Binning-H:" ("string"), w83, w85, w81, "Binning-V:" ("string"), w83, w82, w81) -> (w107:string)
      n124 = Obtain Queue(max queue size (-1, unlimited)=w262, name (unnamed)="back", element data type=w265) -> (queue out=w258:refnum<queue>)  [unwired: 2 in, 2 out]
      n125 = disable-structure shown="Disabled" {
        frame Disabled {
          n126 = property class="IMAQdx" props=["ActiveAttribute", "ValueDBL", "ActiveAttribute", "ValueDBL", "ActiveAttribute", "ValueDBL", "ActiveAttribute", "ValueDBL"]() -> ()  [unwired: 10 in, 2 out]
        }
        frame Enabled {
        }
      }
      n127 = call <vilib>:"IMAQdx Start Acquisition.vi"("error in"=w274, "Session In"=w173) -> ("error out"=w273:errorcluster, "Session Out"=w275:T8)  [unwired: 8 in]
      n128 = local write "Camera Status"(w107) -> ()
    }
    frame #2 {
      # "Main Program"
      n129 = while {
        stop <- w408 stop-if-true
        # "up down voltage steps"
        n130 = case shown="True" "Program 2" {
          frame False {
          }
          frame True {
            n131 = local read "prog 2 step"() -> (w410:dbl)
            n132 = Index Array(array="prog 2 v arr", index=w410) -> (element=w409:dbl)
            n133 = case shown="6" w410 {
              tunnel: w409 -> [_ w418 w427 w435 w443 w451 w459 _]
              frame 0, Default {
                # "hit record, wait 10 seconds"
                n134 = flat-sequence {
                  frame #0 {
                    n135 = property on="RECORD / STOP VIDEO" class="Bool (strict)"("Val(Sgnl)"=TRUE ("Value (Signaling)")) -> ()  [unwired: 2 in, 2 out]
                  }
                  frame #1 {
                    n136 = Multiply(x=u32 10, y=u32 1000 ("milliseconds to wait")) -> (x*y=w415:u32)
                    n137 = Wait (ms)(milliseconds to wait=w415) -> ()  [unwired: 1 out]
                  }
                  frame #2 {
                    n138 = local read "prog 2 step"() -> (w417:dbl)
                    n139 = Increment(x=w417) -> (x+1=w416:dbl)
                    n140 = local write "prog 2 step"(w416) -> ()
                  }
                }
              }
              frame 1 {
                # "turn on voltage 1"
                n141 = flat-sequence {
                  tunnel: w418 -> [w419]
                  frame #0 {
                    n142 = property on="EPD-DC Power" class="Bool (strict)"("Val(Sgnl)"=TRUE ("Value (Signaling)")) -> ()  [unwired: 2 in, 2 out]
                    n143 = control-ref of="EPD Voltage set"() -> (w420:refnum<vi>)
                    n144 = property on="Property Node" class="DigNum (strict)"(reference=w420, "Val(Sgnl)"=w419) -> ()  [unwired: 1 in, 2 out]
                  }
                  frame #1 {
                    n145 = local read "v time p2"() -> (w422:dbl)
                    n146 = Multiply(x=w422, y=u32 1000 ("milliseconds to wait")) -> (x*y=w424:dbl)
                    n147 = Wait (ms)(milliseconds to wait=w424) -> ()  [unwired: 1 out]
                  }
                  frame #2 {
                    n148 = local read "prog 2 step"() -> (w426:dbl)
                    n149 = Increment(x=w426) -> (x+1=w425:dbl)
                    n150 = local write "prog 2 step"(w425) -> ()
                  }
                }
              }
              frame 2 {
                # "turn on voltage 2"
                n151 = flat-sequence {
                  tunnel: w427 -> [w428]
                  frame #0 {
                    n152 = control-ref of="EPD Voltage set"() -> (w429:refnum<vi>)
                    n153 = property on="Property Node" class="DigNum (strict)"(reference=w429, "Val(Sgnl)"=w428) -> ()  [unwired: 1 in, 2 out]
                  }
                  frame #1 {
                    n154 = local read "v time p2"() -> (w430:dbl)
                    n155 = Multiply(x=w430, y=u32 1000 ("milliseconds to wait")) -> (x*y=w432:dbl)
                    n156 = Wait (ms)(milliseconds to wait=w432) -> ()  [unwired: 1 out]
                  }
                  frame #2 {
                    n157 = local read "prog 2 step"() -> (w434:dbl)
                    n158 = Increment(x=w434) -> (x+1=w433:dbl)
                    n159 = local write "prog 2 step"(w433) -> ()
                  }
                }
              }
              frame 3 {
                # "turn on voltage 2"
                n160 = flat-sequence {
                  tunnel: w435 -> [w436]
                  frame #0 {
                    n161 = control-ref of="EPD Voltage set"() -> (w437:refnum<vi>)
                    n162 = property on="Property Node" class="DigNum (strict)"(reference=w437, "Val(Sgnl)"=w436) -> ()  [unwired: 1 in, 2 out]
                  }
                  frame #1 {
                    n163 = local read "v time p2"() -> (w438:dbl)
                    n164 = Multiply(x=w438, y=u32 1000 ("milliseconds to wait")) -> (x*y=w440:dbl)
                    n165 = Wait (ms)(milliseconds to wait=w440) -> ()  [unwired: 1 out]
                  }
                  frame #2 {
                    n166 = local read "prog 2 step"() -> (w442:dbl)
                    n167 = Increment(x=w442) -> (x+1=w441:dbl)
                    n168 = local write "prog 2 step"(w441) -> ()
                  }
                }
              }
              frame 4 {
                # "turn on voltage 2"
                n169 = flat-sequence {
                  tunnel: w443 -> [w444]
                  frame #0 {
                    n170 = control-ref of="EPD Voltage set"() -> (w445:refnum<vi>)
                    n171 = property on="Property Node" class="DigNum (strict)"(reference=w445, "Val(Sgnl)"=w444) -> ()  [unwired: 1 in, 2 out]
                  }
                  frame #1 {
                    n172 = local read "v time p2"() -> (w446:dbl)
                    n173 = Multiply(x=w446, y=u32 1000 ("milliseconds to wait")) -> (x*y=w448:dbl)
                    n174 = Wait (ms)(milliseconds to wait=w448) -> ()  [unwired: 1 out]
                  }
                  frame #2 {
                    n175 = local read "prog 2 step"() -> (w450:dbl)
                    n176 = Increment(x=w450) -> (x+1=w449:dbl)
                    n177 = local write "prog 2 step"(w449) -> ()
                  }
                }
              }
              frame 5 {
                # "turn on voltage 2"
                n178 = flat-sequence {
                  tunnel: w451 -> [w452]
                  frame #0 {
                    n179 = control-ref of="EPD Voltage set"() -> (w453:refnum<vi>)
                    n180 = property on="Property Node" class="DigNum (strict)"(reference=w453, "Val(Sgnl)"=w452) -> ()  [unwired: 1 in, 2 out]
                  }
                  frame #1 {
                    n181 = local read "v time p2"() -> (w454:dbl)
                    n182 = Multiply(x=w454, y=u32 1000 ("milliseconds to wait")) -> (x*y=w456:dbl)
                    n183 = Wait (ms)(milliseconds to wait=w456) -> ()  [unwired: 1 out]
                  }
                  frame #2 {
                    n184 = local read "prog 2 step"() -> (w458:dbl)
                    n185 = Increment(x=w458) -> (x+1=w457:dbl)
                    n186 = local write "prog 2 step"(w457) -> ()
                  }
                }
              }
              frame 6 {
                # "turn on voltage 2"
                n187 = flat-sequence {
                  tunnel: w459 -> [w460]
                  frame #0 {
                    n188 = control-ref of="EPD Voltage set"() -> (w461:refnum<vi>)
                    n189 = property on="Property Node" class="DigNum (strict)"(reference=w461, "Val(Sgnl)"=w460) -> ()  [unwired: 1 in, 2 out]
                  }
                  frame #1 {
                    n190 = local read "v time p2"() -> (w462:dbl)
                    n191 = Multiply(x=w462, y=u32 1000 ("milliseconds to wait")) -> (x*y=w464:dbl)
                    n192 = Wait (ms)(milliseconds to wait=w464) -> ()  [unwired: 1 out]
                  }
                  frame #2 {
                    n193 = local read "prog 2 step"() -> (w466:dbl)
                    n194 = Increment(x=w466) -> (x+1=w465:dbl)
                    n195 = local write "prog 2 step"(w465) -> ()
                  }
                }
              }
              frame 7 {
                # "turn on voltage 2"
                n196 = flat-sequence {
                  frame #0 {
                    n197 = local read "Record Step"() -> (w469:u8)
                    n198 = Increment(x=w469) -> (x+1=w468:u8)
                    n199 = local write "Record Step"(w468) -> ()
                    n200 = property on="EPD-DC Power" class="Bool (strict)"("Val(Sgnl)"=FALSE ("Value (Signaling)")) -> ()  [unwired: 2 in, 2 out]
                  }
                  frame #1 {
                    n201 = Multiply(x=u32 10, y=u32 1000 ("milliseconds to wait")) -> (x*y=w472:u32)
                    n202 = Wait (ms)(milliseconds to wait=w472) -> ()  [unwired: 1 out]
                  }
                  frame #2 {
                    n203 = property on="RECORD / STOP VIDEO" class="Bool (strict)"("Value"=FALSE ("Value (Signaling)")) -> ()  [unwired: 2 in, 2 out]
                    n204 = local write "prog 2 step"(0.0 ("prog1 step")) -> ()
                    n205 = local write "Program 2"(FALSE ("Program 1")) -> ()
                  }
                }
              }
            }
          }
        }
        n206 = local read "stop"() -> (w408:bool)
      }
      n207 = while {
        stop <- w477 stop-if-true
        # "Autorecord 1 minute deposition"
        n208 = case shown="True" "Program 1" {
          frame False {
          }
          frame True {
            n209 = local read "prog1 step"() -> (w478:dbl)
            n210 = case shown="1" w478 {
              frame 0, Default {
                n211 = flat-sequence {
                  frame #0 {
                    n212 = property on="RECORD / STOP VIDEO" class="Bool (strict)"("Val(Sgnl)"=TRUE ("Value (Signaling)")) -> ()  [unwired: 2 in, 2 out]
                  }
                  frame #1 {
                    n213 = Multiply(x="init time", y=u32 1000 ("milliseconds to wait")) -> (x*y=w480:dbl)
                    n214 = Wait (ms)(milliseconds to wait=w480) -> ()  [unwired: 1 out]
                  }
                  frame #2 {
                    n215 = local read "prog1 step"() -> (w484:dbl)
                    n216 = Increment(x=w484) -> (x+1=w483:dbl)
                    n217 = local write "prog1 step"(w483) -> ()
                  }
                }
              }
              frame 1 {
                n218 = flat-sequence {
                  frame #0 {
                    n219 = property on="EPD-DC Power" class="Bool (strict)"("Val(Sgnl)"=TRUE ("Value (Signaling)")) -> ()  [unwired: 2 in, 2 out]
                  }
                  frame #1 {
                    n220 = Multiply(x="v time", y=u32 1000 ("milliseconds to wait")) -> (x*y=w486:dbl)
                    n221 = Wait (ms)(milliseconds to wait=w486) -> ()  [unwired: 1 out]
                  }
                  frame #2 {
                    n222 = local read "prog1 step"() -> (w490:dbl)
                    n223 = Increment(x=w490) -> (x+1=w489:dbl)
                    n224 = local write "prog1 step"(w489) -> ()
                  }
                }
              }
              frame 2 {
                n225 = flat-sequence {
                  frame #0 {
                    n226 = property on="EPD-DC Power" class="Bool (strict)"("Val(Sgnl)"=FALSE ("Value (Signaling)")) -> ()  [unwired: 2 in, 2 out]
                  }
                  frame #1 {
                    n227 = Multiply(x="de-init time", y=u32 1000 ("milliseconds to wait")) -> (x*y=w492:dbl)
                    n228 = Wait (ms)(milliseconds to wait=w492) -> ()  [unwired: 1 out]
                  }
                  frame #2 {
                    n229 = local read "prog1 step"() -> (w496:dbl)
                    n230 = Increment(x=w496) -> (x+1=w495:dbl)
                    n231 = local write "prog1 step"(w495) -> ()
                  }
                }
              }
              frame 3 {
                n232 = flat-sequence {
                  frame #0 {
                    n233 = local read "Record Step"() -> (w498:u8)
                    n234 = Increment(x=w498) -> (x+1=w497:u8)
                    n235 = local write "Record Step"(w497) -> ()
                  }
                  frame #1 {
                    n236 = property on="RECORD / STOP VIDEO" class="Bool (strict)"("Value"=FALSE ("Value (Signaling)")) -> ()  [unwired: 2 in, 2 out]
                    n237 = local write "Program 1"(FALSE ("Program 1")) -> ()
                    n238 = local write "prog1 step"(0.0 ("prog1 step")) -> ()
                  }
                }
              }
            }
          }
        }
        n239 = local read "stop"() -> (w477:bool)
      }
      n240 = call "IMAQ Create"("Image Name"="display image") -> ("New Image"=w373:T1)  [unwired: 4 in, 1 out]
      n241 = while {
        tunnel: w380 -> [w627]
        tunnel: [w626] -> w379
        stop <- w628 stop-if-true
        # "print loop"
        n242 = local read "print image button"() -> (w629:bool)
        n243 = case shown="True" w629 {
          tunnel: w627 -> [_ w631]
          tunnel: [_ w630] -> w626
          frame False {
          }
          frame True {
            n244 = flat-sequence {
              tunnel: w631 -> [w633]
              tunnel: [w632] -> w630
              frame #0 {
                n245 = local read "resampled image"() -> (w634:u8[][])
                n246 = local read "output resolution"() -> (w637:dbl)
                n247 = Initialize Array(0.0 ("element"), w637, w637) -> (w636:dbl[][])
                n248 = local write "initialized array"(w636) -> ()
                n249 = local write "live print map"(w636) -> ()
                n250 = for {
                  tunnel: w634 -> [w640] mode=indexing
                  tunnel: w633 -> [w639]
                  tunnel: [w638] -> w632
                  i -> [w641]
                  n251 = for {
                    tunnel: w640 -> [w644] mode=indexing
                    tunnel: w639 -> [w643]
                    tunnel: [w642] -> w638 mode=indexing
                    i -> [w647]
                    n252 = Greater?(x=w644, y=u8 0) -> (0:w645:bool)
                    n253 = case shown="True" w645 {
                      tunnel: w644 -> [_ w652]
                      tunnel: w643 -> [_ w651]
                      tunnel: [_ w648] -> w642
                      frame False {
                      }
                      frame True {
                        n254 = flat-sequence {
                          tunnel: [w703] -> w653
                          tunnel: w652 -> [w703]
                          tunnel: w651 -> [w687]
                          tunnel: [w657] -> w650
                          tunnel: [w654] -> w649
                          tunnel: [w688] -> w648
                          tunnel: w653 -> [w766]
                          tunnel: w650 -> [w765]
                          tunnel: w649 -> [w764]
                          frame #0 {
                            w672 = u16 2 items=["Channel 1"=1, "Channel 2"=2] ("Channel (1 Channel 1)")
                            w673 = u16 1 items=["Channel 1"=1, "Channel 2"=2] ("Channel (1 Channel 1)")
                            w666 = u16 3 items=["Sine", "Square", "Pulse", "Ramp", "Noise"] ("Waveform Function (0: Sine)")
                            n255 = local read "set volts"() -> (w704:dbl)
                            n256 = local read "y"() -> (w654:i32)
                            n257 = local read "x"() -> (w657:i32)
                            n258 = local read "aobd max"() -> (w692:dbl)
                            n259 = local read "aobd min"() -> (w693:dbl)
                            n260 = local read "output resolution"() -> (w694:dbl)
                            n261 = local read "aobd max"() -> (w699:dbl)
                            n262 = local read "aobd min"() -> (w698:dbl)
                            n263 = local read "output resolution"() -> (w697:dbl)
                            n264 = local read "aobd min"() -> (w695:dbl)
                            n265 = local read "aobd min"() -> (w696:dbl)
                            n266 = local write "applied volts"(w704) -> ()
                            n267 = flat-sequence {
                              tunnel: w687 -> [w711]
                              tunnel: w687 -> [w710]
                              tunnel: [w710] -> w686
                              tunnel: [w709] -> w685
                              tunnel: w673 -> [w708]
                              tunnel: [w707] -> w670
                              tunnel: u32 200 ("milliseconds to wait") -> [w706]
                              tunnel: [w706] -> w664
                              tunnel: w686 -> [w719]
                              tunnel: w685 -> [w718]
                              tunnel: [w718] -> w684
                              tunnel: [w717] -> w683
                              tunnel: w672 -> [w716]
                              tunnel: w670 -> [w715]
                              tunnel: [w714] -> w669
                              tunnel: w664 -> [w713]
                              tunnel: [w713] -> w663
                              tunnel: w684 -> [w728]
                              tunnel: w683 -> [w727]
                              tunnel: [w727] -> w682
                              tunnel: [w726] -> w681
                              tunnel: w673 -> [w725]
                              tunnel: w669 -> [w724]
                              tunnel: [w723] -> w668
                              tunnel: w666 -> [w722]
                              tunnel: w663 -> [w721]
                              tunnel: [w721] -> w662
                              tunnel: w682 -> [w736]
                              tunnel: w681 -> [w735]
                              tunnel: [w735] -> w680
                              tunnel: [w734] -> w677
                              tunnel: w672 -> [w733]
                              tunnel: w668 -> [w732]
                              tunnel: [w731] -> w667
                              tunnel: w666 -> [w730]
                              tunnel: w662 -> [w729]
                              tunnel: [w729] -> w661
                              tunnel: w680 -> [w745]
                              tunnel: [w744] -> w679
                              tunnel: w677 -> [w743]
                              tunnel: [w743] -> w676
                              tunnel: w673 -> [w742]
                              tunnel: w656 -> [w741]
                              tunnel: [w739] -> w671
                              tunnel: w667 -> [w738]
                              tunnel: w661 -> [w737]
                              tunnel: [w737] -> w660
                              tunnel: w679 -> [w753]
                              tunnel: [w753] -> w678
                              tunnel: w676 -> [w752]
                              tunnel: [w751] -> w675
                              tunnel: w672 -> [w750]
                              tunnel: w655 -> [w749]
                              tunnel: w671 -> [w747]
                              tunnel: w660 -> [w746]
                              tunnel: [w746] -> w659
                              tunnel: w678 -> [w758]
                              tunnel: w675 -> [w757]
                              tunnel: [w757] -> w674
                              tunnel: w673 -> [w756]
                              tunnel: w659 -> [w754]
                              tunnel: [w754] -> w658
                              tunnel: [w763] -> w688
                              tunnel: w674 -> [w762]
                              tunnel: w672 -> [w761]
                              tunnel: w658 -> [w759]
                              frame #0 {
                                n268 = Wait (ms)(milliseconds to wait=w706) -> ()  [unwired: 1 out]
                                n269 = call <instrlib>:"Enable Output.vi"("Enable Output (T: Enable)"=FALSE, "Channel (1: Channel 1)"=w708, "VISA resource name"=w711) -> ("error out"=w707:errorcluster, "VISA resource name out"=w709:refnum<visa-resource-name>)  [unwired: 7 in]
                              }
                              frame #1 {
                                n270 = Wait (ms)(milliseconds to wait=w713) -> ()  [unwired: 1 out]
                                n271 = call <instrlib>:"Enable Output.vi"("Enable Output (T: Enable)"=FALSE, "error in (no error)"=w715, "Channel (1: Channel 1)"=w716, "VISA resource name"=w719) -> ("error out"=w714:errorcluster, "VISA resource name out"=w717:refnum<visa-resource-name>)  [unwired: 6 in]
                              }
                              frame #2 {
                                n272 = Wait (ms)(milliseconds to wait=w721) -> ()  [unwired: 1 out]
                                n273 = call <instrlib>:"Configure Standard Waveform.vi"("error in (no error)"=w724, "Waveform Function (0: Sine)"=w722, "Channel (1 Channel 1)"=w725, "VISA resource name"=w728) -> ("error out"=w723:errorcluster, "VISA resource name out"=w726:refnum<visa-resource-name>)  [unwired: 6 in]
                              }
                              frame #3 {
                                n274 = call <instrlib>:"Configure Standard Waveform.vi"("error in (no error)"=w732, "Waveform Function (0: Sine)"=w730, "Channel (1 Channel 1)"=w733, "VISA resource name"=w736) -> ("error out"=w731:errorcluster, "VISA resource name out"=w734:refnum<visa-resource-name>)  [unwired: 6 in]
                                n275 = Wait (ms)(milliseconds to wait=w729) -> ()  [unwired: 1 out]
                              }
                              frame #4 {
                                w739 = 0.1 ("Amplitude (1 Vpp)")
                                n276 = Wait (ms)(milliseconds to wait=w737) -> ()  [unwired: 1 out]
                                n277 = call <instrlib>:"Configure Waveform.vi"("Frequency (1000 Hz)"=79000.0, "DC Offset (0.00 V)"=w741, "error in (no error)"=w738, "Amplitude (1 Vpp)"=w739, "Channel (1 Channel 1)"=w742, "VISA resource name"=w745) -> ("VISA resource name out"=w744:refnum<visa-resource-name>)  [unwired: 4 in, 1 out]
                              }
                              frame #5 {
                                n278 = call <instrlib>:"Configure Waveform.vi"("Frequency (1000 Hz)"=83000.0, "DC Offset (0.00 V)"=w749, "Amplitude (1 Vpp)"=w747, "Channel (1 Channel 1)"=w750, "VISA resource name"=w752) -> ("VISA resource name out"=w751:refnum<visa-resource-name>)  [unwired: 5 in, 1 out]
                                n279 = Wait (ms)(milliseconds to wait=w746) -> ()  [unwired: 1 out]
                              }
                              frame #6 {
                                n280 = call <instrlib>:"Enable Output.vi"("Enable Output (T: Enable)"=TRUE, "Channel (1: Channel 1)"=w756, "VISA resource name"=w758) -> ()  [unwired: 7 in, 2 out]
                                n281 = Wait (ms)(milliseconds to wait=w754) -> ()  [unwired: 1 out]
                              }
                              frame #7 {
                                n282 = call <instrlib>:"Enable Output.vi"("Enable Output (T: Enable)"=TRUE, "Channel (1: Channel 1)"=w761, "VISA resource name"=w762) -> ("error out"=w763:errorcluster)  [unwired: 7 in, 1 out]
                                n283 = Wait (ms)(milliseconds to wait=w759) -> ()  [unwired: 1 out]
                              }
                            }
                            n284 = Subtract(x=w692, y=w693) -> (x-y=w691:dbl)
                            n285 = Subtract(x=w699, y=w698) -> (x-y=w700:dbl)
                            n286 = Multiply(x=w657, y=w691) -> (x*y=w690:dbl)
                            n287 = Multiply(x=w654, y=w700) -> (x*y=w701:dbl)
                            n288 = Divide(x=w690, y=w694) -> (x/y=w689:dbl)
                            n289 = Divide(x=w701, y=w697) -> (x/y=w702:dbl)
                            n290 = Add(x=w689, y=w695) -> (x+y=w656:dbl)
                            n291 = Add(x=w702, y=w696) -> (x+y=w655:dbl)
                            n292 = local write "aobd x"(w656) -> ()
                            n293 = local write "volts on?"(TRUE ("volts on?")) -> ()
                            n294 = local write "aobd y"(w655) -> ()
                          }
                          frame #1 {
                            n295 = while {
                              tunnel: w766 -> [w777]
                              tunnel: w765 -> [w768]
                              tunnel: w764 -> [w767]
                              i -> [w778]
                              stop <- w776 stop-if-true
                              n296 = local read "initialized array"() -> (w769:dbl[][])
                              n297 = local read "exposure time"() -> (w773:dbl)
                              n298 = Index Array(array=w769, index (row)=w768, index (col)=w767) -> (element=w772:dbl)
                              n299 = Increment(x=w772) -> (x+1=w771:dbl)
                              n300 = Greater?(x=w778, y=w777) -> (0:w776:bool)
                              n301 = Replace Array Subset(array=w769, new element=w771, index (row)=w768, index (col)=w767) -> (w770:dbl[][])
                              n302 = local write "initialized array"(w770) -> ()
                              n303 = local write "live print map"(w770) -> ()
                              n304 = Divide(x=w773, y=256) -> (x/y=w775:dbl)
                              n305 = Wait (ms)(milliseconds to wait=w775) -> ()  [unwired: 1 out]
                            }
                          }
                          frame #2 {
                            n306 = local write "applied volts"(0.0 ("applied volts")) -> ()
                            n307 = local write "volts on?"(TRUE ("volts on?")) -> ()
                          }
                        }
                      }
                    }
                    "y" <- w647
                    "pixel value" <- w644
                  }
                  "x" <- w641
                }
              }
              frame #1 {
                n308 = local write "print image button"(FALSE ("print image button")) -> ()
              }
            }
          }
        }
        n309 = local read "stop"() -> (w628:bool)
      }
      n310 = while {
        stop <- w506 stop-if-true
        # "AOBD LASER POINTER"
        n311 = event shown="[1] \"Image\": Mouse Down" {
          selector: _ -> [_ _]
          dyn-events: _ -> [_ _]
          timeout: 3 -> [_ _]
          event Timeout {
            n312 = event-data() -> ()  [unwired: 1 in, 3 out]
          }
          event "Image": Mouse Down {
            n313 = event-data() -> ()  [unwired: 1 in, 5 out]
            n314 = case shown="True" "move on click" {
              frame False {
              }
              frame True {
                n315 = property on="AOBD GO" class="Bool (strict)"("Val(Sgnl)"=TRUE ("Value (Signaling)")) -> ()  [unwired: 2 in, 2 out]
              }
            }
          }
        }
        n316 = property on="Image" class="ImageControl"() -> ("ROI"=w505:T13)  [unwired: 2 in, 2 out]
        n317 = local read "stop"() -> (w506:bool)
        n318 = Unbundle(w505) -> ("Global Rectangle"=w503:i32[])  [unwired: 1 out]
        "Global Rectangle" <- w503
        n319 = Empty Array?(array=w503) -> (empty?=w504:bool)
        n320 = case shown="False" w504 {
          tunnel: w503 -> [w545 _]
          frame False {
            w534 = 1000
            n321 = local read "2x binning"() -> (w511:bool)
            n322 = property on="Camera pixels" class="CmbBox"() -> ("Text.Text"=w512:string)  [unwired: 2 in, 2 out]
            n323 = Decimal String To Number(string=w512) -> (number=w514:i32)  [unwired: 2 in, 1 out]
            n324 = Select(t=2.0, s=w511, f=1.0) -> (s? t:f=w513:dbl)
            n325 = Multiply(x=w514, y=w513) -> (x*y=w515:dbl)
            n326 = case shown="1024" w515 {
              frame 0, Default {
                n327 = local write "AOBD MAX"(4.7 ("element")) -> ()
                n328 = local write "AOBD MIN"(1.6 ("element")) -> ()
              }
              frame 64 {
                n329 = local write "AOBD MAX"(3.3 ("element")) -> ()
                n330 = local write "AOBD MIN"(3.1 ("element")) -> ()
              }
              frame 128 {
                n331 = local write "AOBD MAX"(3.4 ("element")) -> ()
                n332 = local write "AOBD MIN"(3.0 ("element")) -> ()
              }
              frame 256 {
                n333 = local write "AOBD MAX"(3.6 ("element")) -> ()
                n334 = local write "AOBD MIN"(2.8 ("element")) -> ()
              }
              frame 512 {
                n335 = local write "AOBD MAX"(3.9 ("element")) -> ()
                n336 = local write "AOBD MIN"(2.4 ("element")) -> ()
              }
              frame 1024 {
                n337 = local write "AOBD MAX"(4.7 ("element")) -> ()
                n338 = local write "AOBD MIN"(1.6 ("element")) -> ()
              }
            }
            n339 = Index Array(array=w545, index=0) -> (element=w518:i32)
            n340 = Index Array(array=w545, index=1) -> (element=w519:i32)
            n341 = Index Array(array=w545, index=2) -> ()  [unwired: 1 out]
            n342 = Index Array(array=w545, index=3) -> ()  [unwired: 1 out]
            n343 = local read "Y"() -> (w520:dbl)
            n344 = local read "X"() -> (w521:dbl)
            n345 = Subtract(x=w521, y=w518) -> (x-y=w516:dbl)
            n346 = Subtract(x=w520, y=w519) -> (x-y=w517:dbl)
            n347 = local read "X"() -> (w539:dbl)
            n348 = local read "Y"() -> (w540:dbl)
            n349 = Divide(x=w516, y=w539) -> (x/y=w537:dbl)
            n350 = Divide(x=w517, y=w540) -> (x/y=w538:dbl)
            n351 = local read "AOBD MIN"() -> (w529:dbl)
            n352 = local read "AOBD MAX"() -> (w531:dbl)
            n353 = Subtract(x=w531, y=w529) -> (x-y=w530:dbl)
            n354 = local read "AOBD MIN"() -> (w524:dbl)
            n355 = Multiply(x=w538, y=w530) -> (x*y=w528:dbl)
            n356 = Multiply(x=w530, y=w537) -> (x*y=w527:dbl)
            n357 = Add(x=w527, y=w524) -> (x+y=w523:dbl)
            n358 = Add(x=w528, y=w524) -> (x+y=w522:dbl)
            n359 = Multiply(x=w523, y=w534) -> (x*y=w536:dbl)
            n360 = Multiply(x=w534, y=w522) -> (x*y=w533:dbl)
            n361 = Round To Nearest(number=w536) -> (nearest integer value=w535:dbl)
            n362 = Round To Nearest(number=w533) -> (nearest integer value=w532:dbl)
            n363 = Divide(x=w535, y=w534) -> (x/y=w526:dbl)
            n364 = Divide(x=w532, y=w534) -> (x/y=w525:dbl)
            n365 = local write "AOBD X"(w525) -> ()
            n366 = local write "AOBD Y"(w526) -> ()
          }
          frame True {
          }
        }
      }
      n367 = while {
        tunnel: [w1504] -> w406
        tunnel: w404 -> [w1503]
        stop <- w1505 stop-if-true
        # "Button Functions"
        n368 = event shown="[13] \"Save Experiment Log\": Value Change" {
          selector: _ -> [_ _ _ _ _ _ _ _ _ _ _ _ _ _ _ _ _]
          dyn-events: _ -> [_ _ _ _ _ _ _ _ _ _ _ _ _ _ _ _ _]
          timeout: 10 -> [_ _ _ _ _ _ _ _ _ _ _ _ _ _ _ _ _]
          tunnel: [_ w1508 w1564 w1573 w1577 w1582 w1592 w1604 w1615 w1626 w1637 w1640 w1647 w1660 _ _ _] -> w1504
          tunnel: w1503 -> [_ w1509 w1563 w1574 w1576 w1581 w1593 w1605 w1616 w1627 w1638 w1639 w1649 _ _ _ _]
          event Timeout {
            n369 = event-data() -> ()  [unwired: 1 in, 3 out]
          }
          event "Refresh": Value Change {
            w1559 = "\t"
            w1561 = "\r\n"
            n370 = event-data() -> ()  [unwired: 1 in, 6 out]
            n371 = local write "Refresh"(FALSE ("Refresh")) -> ()
            n372 = property class="IMAQdx"(reference=w1509, "ActiveAttribute"="CameraAttributes::AcquisitionControl::ExposureTime", "ActiveAttribute"="CameraAttributes::AcquisitionControl::AcquisitionFrameRate", "ActiveAttribute"="CameraAttributes::ImageFormatControl::Width", "ActiveAttribute"="CameraAttributes::ImageFormatControl::Height", "ActiveAttribute"="CameraAttributes::ImageFormatControl::OffsetX", "ActiveAttribute"="CameraAttributes::ImageFormatControl::OffsetY", "ActiveAttribute"="CameraAttributes::ImageFormatControl::BinningHorizontal", "ActiveAttribute"="CameraAttributes::ImageFormatControl::BinningVertical", "ActiveAttribute"="CameraAttributes::AnalogControl::GainAuto", "ActiveAttribute"="CameraAttributes::AnalogControl::Gain", "ActiveAttribute"="CameraAttributes::AcquisitionControl::AcquisitionMode", "ActiveAttribute"="CameraAttributes::AcquisitionControl::AcquisitionFrameRateEnable", "ActiveAttribute"="CameraAttributes::AcquisitionControl::ExposureMode", "ActiveAttribute"="CameraAttributes::DigitalIOControl::LineSelector", "ActiveAttribute"="CameraAttributes::DigitalIOControl::LineMode", "ActiveAttribute"="CameraAttributes::DigitalIOControl::LineInverter") -> (error out=w1508:errorcluster, "ValueDBL"=w1511:dbl, "ValueDBL"=w1507:dbl, "ValueDBL"=w1514:dbl, "ValueDBL"=w1513:dbl, "ValueDBL"=w1515:dbl, "ValueDBL"=w1516:dbl, "ValueDBL"=w1517:dbl, "ValueDBL"=w1518:dbl, "ValueDBL"=w1519:dbl, "ValueDBL"=w1520:dbl, "ValueDBL"=w1521:dbl, "ValueDBL"=w1510:dbl, "ValueDBL"=w1522:dbl, "ValueDBL"=w1523:dbl, "ValueDBL"=w1524:dbl, "ValueDBL"=w1525:dbl)  [unwired: 1 in, 1 out]
            n373 = local write "exp time"(w1511) -> ()
            n374 = local write "binning vertical"(w1518) -> ()
            n375 = local write "frame rate"(w1507) -> ()
            n376 = local write "binning horizontal"(w1517) -> ()
            n377 = local write "AcquisitionFrameRateEnable"(w1510) -> ()
            n378 = local write "ExposureMode"(w1522) -> ()
            n379 = local write "offsetx"(w1515) -> ()
            n380 = local write "Gain Auto"(w1519) -> ()
            n381 = local write "width"(w1514) -> ()
            n382 = local write "height"(w1513) -> ()
            n383 = local write "Line Selector"(w1523) -> ()
            n384 = local write "Line Inverter"(w1525) -> ()
            n385 = local write "AcquisitionMode"(w1521) -> ()
            n386 = local write "offsety"(w1516) -> ()
            n387 = local write "Gain (dB)"(w1520) -> ()
            n388 = local write "Line Mode"(w1524) -> ()
            n389 = Number To Decimal String(number=w1507) -> (decimal integer string=w1547:string)  [unwired: 1 in]
            n390 = Number To Decimal String(number=w1511) -> (decimal integer string=w1545:string)  [unwired: 1 in]
            n391 = Number To Decimal String(number=w1514) -> (decimal integer string=w1549:string)  [unwired: 1 in]
            n392 = Number To Decimal String(number=w1513) -> (decimal integer string=w1554:string)  [unwired: 1 in]
            n393 = Number To Decimal String(number=w1515) -> (decimal integer string=w1555:string)  [unwired: 1 in]
            n394 = Number To Decimal String(number=w1516) -> (decimal integer string=w1556:string)  [unwired: 1 in]
            n395 = Number To Decimal String(number=w1518) -> (decimal integer string=w1560:string)  [unwired: 1 in]
            n396 = Number To Decimal String(number=w1517) -> (decimal integer string=w1557:string)  [unwired: 1 in]
            n397 = Divide(x=1000000.0, y=w1507) -> (x/y=w1526:dbl)
            n398 = local write "sync exp"(w1526) -> ()
            n399 = Concatenate Strings("Exposure Time (us):" ("string"), w1559, w1545, w1561, "Frame Rate (fps):" ("string"), w1559, w1547, w1561, "Width (px):" ("string"), w1559, w1549, w1561, "Height (px):" ("string"), w1559, w1554, w1561, "Offset X (px):" ("string"), w1559, w1555, w1561, "Offset Y (px):" ("string"), w1559, w1556, w1561, "Binning-H:" ("string"), w1559, w1557, w1561, "Binning-V:" ("string"), w1559, w1560, w1561) -> (w1543:string)
            n400 = local write "Camera Status"(w1543) -> ()
          }
          event "Auto Exposure": Value Change {
            n401 = event-data() -> ()  [unwired: 1 in, 6 out]
            n402 = local read "Auto Exposure"() -> (w1565:string)
            n403 = Decimal String To Number(string=w1565) -> (number=w1567:i32)  [unwired: 2 in, 1 out]
            n404 = property class="IMAQdx"(reference=w1563, "ActiveAttribute"="CameraAttributes::AcquisitionControl::ExposureAuto", "ValueDBL"=w1567) -> (error out=w1564:errorcluster)  [unwired: 1 in, 1 out]
          }
          event "Exposure Time (us)": Value Change {
            w1571 = "CameraAttributes::AcquisitionControl::ExposureTime"
            n405 = event-data() -> ()  [unwired: 1 in, 6 out]
            n406 = local read "Exposure Time (us)"() -> (w1575:dbl)
            n407 = property class="IMAQdx"(reference=w1574, "ActiveAttribute"=w1571, "ValueDBL"=w1575) -> (reference out=w1570:T8, error out=w1569:errorcluster)  [unwired: 1 in]
            n408 = property class="IMAQdx"(reference=w1570, error in=w1569, "ActiveAttribute"=w1571) -> (error out=w1573:errorcluster, "ValueDBL"=w1572:dbl)  [unwired: 1 out]
            n409 = local write "exp time"(w1572) -> ()
            n410 = property on="Refresh" class="Bool (strict)"("Val(Sgnl)"=TRUE ("Value (Signaling)")) -> ()  [unwired: 2 in, 2 out]
          }
          event "Auto Framerate": Value Change {
            n411 = event-data() -> ()  [unwired: 1 in, 6 out]
            n412 = local read "Auto Framerate"() -> (w1578:string)
            n413 = Decimal String To Number(string=w1578) -> (number=w1579:i32)  [unwired: 2 in, 1 out]
            n414 = property class="IMAQdx"(reference=w1576, "ActiveAttribute"="CameraAttributes::AcquisitionControl::AcquisitionFrameRateAuto", "ValueDBL"=w1579) -> (error out=w1577:errorcluster)  [unwired: 1 in, 1 out]
          }
          event "Manual Framerate Enabled?": Value Change {
            n415 = event-data() -> ()  [unwired: 1 in, 6 out]
            n416 = local read "Manual Framerate Enabled?"() -> (w1583:bool)
            n417 = property class="IMAQdx"(reference=w1581, "ActiveAttribute"="CameraAttributes::AcquisitionControl::AcquisitionFrameRateEnabled", "ValueBool"=w1583) -> (error out=w1582:errorcluster)  [unwired: 1 in, 1 out]
          }
          event "Frame Rate (hz)": Value Change {
            w1591 = "CameraAttributes::AcquisitionControl::AcquisitionFrameRate"
            n418 = event-data() -> ()  [unwired: 1 in, 6 out]
            n419 = local read "Frame Rate (hz)"() -> (w1594:dbl)
            n420 = property class="IMAQdx"(reference=w1593, "ActiveAttribute"=w1591, "ValueDBL"=w1594) -> (reference out=w1590:T8, error out=w1586:errorcluster)  [unwired: 1 in]
            n421 = property class="IMAQdx"(reference=w1590, error in=w1586, "ActiveAttribute"=w1591) -> (error out=w1592:errorcluster, "ValueDBL"=w1587:dbl)  [unwired: 1 out]
            n422 = local write "frame rate"(w1587) -> ()
            n423 = Divide(x=1000000.0, y=w1587) -> (x/y=w1589:dbl)
            n424 = local write "sync exp"(w1589) -> ()
            n425 = property on="Refresh" class="Bool (strict)"("Val(Sgnl)"=TRUE ("Value (Signaling)")) -> ()  [unwired: 2 in, 2 out]
          }
          event "200 fps": Value Change {
            w1597 = 200.0 ("ValueDBL")
            w1603 = "CameraAttributes::AcquisitionControl::AcquisitionFrameRate"
            n426 = event-data() -> ()  [unwired: 1 in, 6 out]
            n427 = property class="IMAQdx"(reference=w1605, "ActiveAttribute"=w1603, "ValueDBL"=w1597) -> (reference out=w1602:T8, error out=w1598:errorcluster)  [unwired: 1 in]
            n428 = local write "Frame Rate (hz)"(w1597) -> ()
            n429 = local write "200 fps"(FALSE ("200 fps")) -> ()
            n430 = property class="IMAQdx"(reference=w1602, error in=w1598, "ActiveAttribute"=w1603) -> (error out=w1604:errorcluster, "ValueDBL"=w1599:dbl)  [unwired: 1 out]
            n431 = local write "frame rate"(w1599) -> ()
            n432 = Divide(x=1000000.0, y=w1599) -> (x/y=w1601:dbl)
            n433 = local write "sync exp"(w1601) -> ()
            n434 = property on="Refresh" class="Bool (strict)"("Val(Sgnl)"=TRUE ("Value (Signaling)")) -> ()  [unwired: 2 in, 2 out]
          }
          event "500 fps": Value Change {
            w1608 = 500.0 ("ValueDBL")
            w1614 = "CameraAttributes::AcquisitionControl::AcquisitionFrameRate"
            n435 = event-data() -> ()  [unwired: 1 in, 6 out]
            n436 = property class="IMAQdx"(reference=w1616, "ActiveAttribute"=w1614, "ValueDBL"=w1608) -> (reference out=w1613:T8, error out=w1609:errorcluster)  [unwired: 1 in]
            n437 = local write "Frame Rate (hz)"(w1608) -> ()
            n438 = local write "500 fps"(FALSE ("200 fps")) -> ()
            n439 = property class="IMAQdx"(reference=w1613, error in=w1609, "ActiveAttribute"=w1614) -> (error out=w1615:errorcluster, "ValueDBL"=w1610:dbl)  [unwired: 1 out]
            n440 = local write "frame rate"(w1610) -> ()
            n441 = Divide(x=1000000.0, y=w1610) -> (x/y=w1612:dbl)
            n442 = local write "sync exp"(w1612) -> ()
            n443 = property on="Refresh" class="Bool (strict)"("Val(Sgnl)"=TRUE ("Value (Signaling)")) -> ()  [unwired: 2 in, 2 out]
          }
          event "600 fps": Value Change {
            w1619 = 600.0 ("ValueDBL")
            w1625 = "CameraAttributes::AcquisitionControl::AcquisitionFrameRate"
            n444 = event-data() -> ()  [unwired: 1 in, 6 out]
            n445 = property class="IMAQdx"(reference=w1627, "ActiveAttribute"=w1625, "ValueDBL"=w1619) -> (reference out=w1624:T8, error out=w1620:errorcluster)  [unwired: 1 in]
            n446 = local write "Frame Rate (hz)"(w1619) -> ()
            n447 = local write "600 fps"(FALSE ("200 fps")) -> ()
            n448 = property class="IMAQdx"(reference=w1624, error in=w1620, "ActiveAttribute"=w1625) -> (error out=w1626:errorcluster, "ValueDBL"=w1621:dbl)  [unwired: 1 out]
            n449 = local write "frame rate"(w1621) -> ()
            n450 = Divide(x=1000000.0, y=w1621) -> (x/y=w1623:dbl)
            n451 = local write "sync exp"(w1623) -> ()
            n452 = property on="Refresh" class="Bool (strict)"("Val(Sgnl)"=TRUE ("Value (Signaling)")) -> ()  [unwired: 2 in, 2 out]
          }
          event "900 fps": Value Change {
            w1630 = 900.0 ("ValueDBL")
            w1636 = "CameraAttributes::AcquisitionControl::AcquisitionFrameRate"
            n453 = event-data() -> ()  [unwired: 1 in, 6 out]
            n454 = property class="IMAQdx"(reference=w1638, "ActiveAttribute"=w1636, "ValueDBL"=w1630) -> (reference out=w1635:T8, error out=w1631:errorcluster)  [unwired: 1 in]
            n455 = local write "Frame Rate (hz)"(w1630) -> ()
            n456 = local write "900 fps"(FALSE ("200 fps")) -> ()
            n457 = property class="IMAQdx"(reference=w1635, error in=w1631, "ActiveAttribute"=w1636) -> (error out=w1637:errorcluster, "ValueDBL"=w1632:dbl)  [unwired: 1 out]
            n458 = local write "frame rate"(w1632) -> ()
            n459 = Divide(x=1000000.0, y=w1632) -> (x/y=w1634:dbl)
            n460 = local write "sync exp"(w1634) -> ()
            n461 = property on="Refresh" class="Bool (strict)"("Val(Sgnl)"=TRUE ("Value (Signaling)")) -> ()  [unwired: 2 in, 2 out]
          }
          event "Auto Gain": Value Change {
            n462 = event-data() -> ()  [unwired: 1 in, 6 out]
            n463 = local read "Auto Gain"() -> (w1641:string)
            n464 = Decimal String To Number(string=w1641) -> (number=w1642:i32)  [unwired: 2 in, 1 out]
            n465 = property class="IMAQdx"(reference=w1639, "ActiveAttribute"="CameraAttributes::AnalogControl::GainAuto", "ValueDBL"=w1642) -> (error out=w1640:errorcluster)  [unwired: 1 in, 1 out]
          }
          event "Gain (dB)": Value Change {
            w1646 = "CameraAttributes::AnalogControl::Gain"
            n466 = event-data() -> ()  [unwired: 1 in, 6 out]
            n467 = local read "Gain (dB)"() -> (w1650:dbl)
            n468 = property class="IMAQdx"(reference=w1649, "ActiveAttribute"=w1646, "ValueDBL"=w1650) -> (reference out=w1648:T8, error out=w1644:errorcluster)  [unwired: 1 in]
            n469 = property class="IMAQdx"(reference=w1648, error in=w1644, "ActiveAttribute"=w1646) -> (error out=w1647:errorcluster, "ValueDBL"=w1645:dbl)  [unwired: 1 out]
            n470 = local write "Gain (dB)"(w1645) -> ()
          }
          event "Save Experiment Log": Value Change {
            (unwired) "\\VIDEOS\\"
            n471 = event-data() -> ()  [unwired: 1 in, 6 out]
            n472 = local read "Experiment Name"() -> (w1677:string)
            n473 = Get Date/Time In Seconds() -> (seconds since 1Jan1904=w1673:timestamp)
            n474 = local read "Date"() -> (w1676:string)
            n475 = local read "Experiment Log"() -> (w1657:string)
            n476 = Format Date/Time String(time format string (%c)="%Y-%m-%d", seconds (now)=w1673) -> (date/time string=w1672:string)  [unwired: 1 in]
            n477 = local read "Base Path"() -> (w1675:path)
            n478 = Format Date/Time String(time format string (%c)="%H-%M-%S", seconds (now)=w1673) -> (date/time string=w1674:string)  [unwired: 1 in]
            n479 = Concatenate Strings(w1676, w1677) -> (w1678:string)
            n480 = Get Date/Time String() -> (date string=w1656:string, time string=w1653:string)  [unwired: 3 in]
            n481 = Concatenate Strings(w1672, "_", w1674) -> (w1666:string)
            n482 = Build Path(base path=w1675, name or relative path=w1678) -> (appended path=w1668:path)
            n483 = call <vilib>:"Space Constant.vi"() -> ("String"=w1651:string)
            n484 = Concatenate Strings(w1657, "\r", w1656, w1651, w1653, w1651, "Savied Experiment Log") -> (w1654:string)
            n485 = Concatenate Strings(w1666, "Experiment Log.txt" ("string")) -> (w1665:string)
            n486 = local write "Experiment Log"(w1654) -> ()
            n487 = Build Path(base path=w1668, name or relative path=w1665) -> (appended path=w1664:path)
            n488 = call <vilib>:"Create File and Containing Folders.vi"("file path"=w1664) -> ("error out"=w1659:errorcluster, "refnum out"=w1663:refnum<file>)  [unwired: 9 in]
            n489 = Write to Text File(file (use dialog)=w1663, text=w1654, error in=w1659) -> (refnum out=w1662:refnum<file>, error out=w1661:errorcluster)  [unwired: 1 in, 1 out]
            n490 = Close File(refnum=w1662, error in=w1661) -> (error out=w1660:errorcluster)  [unwired: 1 out]
            n491 = local write "Save Experiment Log"(FALSE ("Save Experiment Log")) -> ()
          }
          event "Clear Log": Value Change {
            n492 = event-data() -> ()  [unwired: 1 in, 6 out]
            n493 = local write "Experiment Log"("" ("Experiment Log")) -> ()
            n494 = local write "Clear Log"(FALSE ("Clear ELog")) -> ()
          }
          event "Copy Notes To Log": Value Change {
            w1685 = "\r"
            n495 = event-data() -> ()  [unwired: 1 in, 6 out]
            n496 = local read "Experiment Notes"() -> (w1684:string)
            n497 = local read "Experiment Log"() -> (w1682:string)
            n498 = Concatenate Strings(w1682, w1685, "Experiment Notes:", w1685, w1684, w1685) -> (w1681:string)
            n499 = local write "Experiment Log"(w1681) -> ()
            n500 = local write "Copy Notes To Log"(FALSE ("Copy Notes To Log")) -> ()
          }
          event "set sample name": Value Change {
            n501 = event-data() -> ()  [unwired: 1 in, 6 out]
            n502 = local read "Set Power (mW)"() -> (w1704:dbl)
            n503 = local read "Coverslip"() -> (w1694:string)
            n504 = local read "Material"() -> (w1698:string)
            n505 = local read "conc."() -> (w1696:string)
            n506 = local read "Size"() -> (w1701:string)
            n507 = local read "pH"() -> (w1688:string)
            n508 = Number To Decimal String(number=w1704) -> (decimal integer string=w1690:string)  [unwired: 1 in]
            n509 = call <vilib>:"Space Constant.vi"() -> ("String"=w1699:string)
            n510 = call <vilib>:"Space Constant.vi"() -> ("String"=w1697:string)
            n511 = call <vilib>:"Space Constant.vi"() -> ("String"=w1695:string)
            n512 = call <vilib>:"Space Constant.vi"() -> ("String"=w1693:string)
            n513 = call <vilib>:"Space Constant.vi"() -> ("String"=w1687:string)
            n514 = local write "set sample name"(FALSE ("set sample name")) -> ()
            n515 = Concatenate Strings(w1701, "nm", w1699, w1698, w1697, w1696, w1695, w1694, w1693, "pH", w1688, w1687, "Laser", w1690, "mW") -> (w1703:string)
            n516 = local write "Experiment Name"(w1703) -> ()
          }
        }
        n517 = local read "stop"() -> (w1505:bool)
      }
      n518 = while {
        tunnel: w391 -> [w787]
        tunnel: [w786] -> w390
        tunnel: w383 -> [w785]
        tunnel: [w784] -> w382
        stop <- w788 stop-if-true
        # "READ VOLTAGE"
        n519 = Wait Until Next ms Multiple(millisecond multiple=u32 100) -> ()  [unwired: 1 out]
        n520 = call-poly <vilib>:"DAQmx Read.vi"("task/channels in"=w787, "error in"=w785) -> ("task out"=w786:refnum<k21>, "data"=w783:dbl, "error out"=w784:errorcluster)  [unwired: 11 in]
        "EPD Voltage" <- w783
        n521 = local read "stop"() -> (w788:bool)
        n522 = local write "V"(w783) -> ()
      }
      n523 = while {
        tunnel: w389 -> [w801]
        tunnel: w388 -> [w796]
        tunnel: [w795] -> w387
        tunnel: w384 -> [w791]
        tunnel: [w790] -> w381
        stop <- w802 stop-if-true
        n524 = local read "Frequency (hz)"() -> (w798:dbl)
        n525 = local read "phase (°)"() -> (w797:dbl)
        n526 = local read "Amplitude (V)"() -> (w799:dbl)
        n527 = local read "Offset (V)"() -> (w800:dbl)
        n528 = call <vilib>:"Basic Function Generator.vi"("offset"=w800, "reset signal"=TRUE, "sampling info"=w801, "signal type"="signal type", "phase"=w797, "amplitude"=w799, "frequency"=w798) -> ("signal out"=w793:waveform(dbl))  [unwired: 2 in, 2 out]
        "Waveform Graph" <- w793
        n529 = event shown="[1] \"EPD-DC Power\": Value Change" {
          selector: _ -> [_ _ _ _]
          dyn-events: _ -> [_ _ _ _]
          timeout: 10 -> [_ _ _ _]
          tunnel: w796 -> [w804 w808 w838 w862]
          tunnel: [w804 w807 w839 w861] -> w795
          tunnel: w793 -> [_ _ _ w860]
          tunnel: w791 -> [w803 w806 w841 w859]
          tunnel: [w803 w805 w840 w858] -> w790
          event Timeout {
            n530 = event-data() -> ()  [unwired: 1 in, 3 out]
          }
          event "EPD-DC Power": Value Change {
            n531 = event-data() -> ("NewVal"=w809:bool)  [unwired: 1 in, 5 out]
            n532 = case shown="True" w809 {
              tunnel: w808 -> [w815 w831]
              tunnel: [w814 w830] -> w807
              tunnel: w806 -> [w813 w827]
              tunnel: [w810 w824] -> w805
              frame False {
                n533 = call <vilib>:"DAQmx Stop Task.vi"("task/channels in"=w815, "error in"=w813) -> ("task out"=w822:refnum<k21>, "error out"=w812:errorcluster)  [unwired: 12 in]
                n534 = property on="AC" class="Bool (strict)"("DisabledEnum"=T9."Enabled" ("Disabled")) -> ()  [unwired: 2 in, 2 out]
                n535 = call <vilib>:"Basic Function Generator.vi"("offset"=0.0, "signal type"=T2."Triangle Wave", "amplitude"=0.0, "frequency"=0.0) -> ("signal out"=w816:waveform(dbl))  [unwired: 5 in, 2 out]
                n536 = call-poly <vilib>:"DAQmx Write.vi"("task/channels in"=w822, "data"=w816, "error in"=w812) -> ("task out"=w821:refnum<k21>, "error out"=w811:errorcluster)  [unwired: 10 in, 1 out]
                n537 = call <vilib>:"DAQmx Start Task.vi"("task/channels in"=w821, "error in"=w811) -> ("task out"=w814:refnum<k21>, "error out"=w810:errorcluster)  [unwired: 12 in]
              }
              frame True {
                n538 = local read "EPD Voltage set"() -> (w829:dbl)
                n539 = call <vilib>:"DAQmx Stop Task.vi"("task/channels in"=w831) -> ("task out"=w836:refnum<k21>)  [unwired: 13 in, 1 out]
                n540 = call <vilib>:"Basic Function Generator.vi"("offset"=w829, "signal type"=T2."Triangle Wave", "error in (no error)"=w827, "amplitude"=0.0, "frequency"=0.0) -> ("error out"=w826:errorcluster, "signal out"=w837:waveform(dbl))  [unwired: 4 in, 1 out]
                n541 = call-poly <vilib>:"DAQmx Write.vi"("task/channels in"=w836, "data"=w837, "error in"=w826) -> ("task out"=w835:refnum<k21>, "error out"=w825:errorcluster)  [unwired: 10 in, 1 out]
                n542 = call <vilib>:"DAQmx Start Task.vi"("task/channels in"=w835, "error in"=w825) -> ("task out"=w830:refnum<k21>, "error out"=w824:errorcluster)  [unwired: 12 in]
                n543 = property on="AC" class="Bool (strict)"("DisabledEnum"=T9."Disabled and Grayed Out" ("Disabled")) -> ()  [unwired: 2 in, 2 out]
              }
            }
          }
          event "EPD Voltage set": Value Change {
            n544 = event-data() -> ()  [unwired: 1 in, 6 out]
            n545 = local read "EPD-DC Power"() -> (w842:bool)
            n546 = case shown="True" w842 {
              tunnel: w841 -> [w843 w849]
              tunnel: [w843 w848] -> w840
              tunnel: [w844 w847] -> w839
              tunnel: w838 -> [w844 w846]
              frame False {
              }
              frame True {
                n547 = local read "EPD Voltage set"() -> (w845:dbl)
                n548 = call <vilib>:"DAQmx Stop Task.vi"("task/channels in"=w846) -> ("task out"=w854:refnum<k21>)  [unwired: 13 in, 1 out]
                n549 = call <vilib>:"Basic Function Generator.vi"("offset"=w845, "signal type"=T2."Triangle Wave", "error in (no error)"=w849, "amplitude"=0.0, "frequency"=0.0) -> ("error out"=w856:errorcluster, "signal out"=w853:waveform(dbl))  [unwired: 4 in, 1 out]
                n550 = call-poly <vilib>:"DAQmx Write.vi"("task/channels in"=w854, "data"=w853, "error in"=w856) -> ("task out"=w855:refnum<k21>, "error out"=w857:errorcluster)  [unwired: 10 in, 1 out]
                n551 = call <vilib>:"DAQmx Start Task.vi"("task/channels in"=w855, "error in"=w857) -> ("task out"=w847:refnum<k21>, "error out"=w848:errorcluster)  [unwired: 12 in]
              }
            }
          }
          event "AC": Value Change {
            n552 = event-data() -> ("NewVal"=w863:bool)  [unwired: 1 in, 5 out]
            n553 = case shown="True" w863 {
              tunnel: w862 -> [w869 w884]
              tunnel: [w868 w883] -> w861
              tunnel: w860 -> [_ w882]
              tunnel: w859 -> [w867 w881]
              tunnel: [w864 w878] -> w858
              frame False {
                n554 = call <vilib>:"DAQmx Stop Task.vi"("task/channels in"=w869, "error in"=w867) -> ("task out"=w873:refnum<k21>, "error out"=w866:errorcluster)  [unwired: 12 in]
                n555 = property on="EPD-DC Power" class="Bool (strict)"("DisabledEnum"=T9."Enabled" ("Disabled")) -> ()  [unwired: 2 in, 2 out]
                n556 = call <vilib>:"Basic Function Generator.vi"("offset"=0.0, "signal type"=T2."Triangle Wave", "amplitude"=0.0, "frequency"=0.0) -> ("signal out"=w871:waveform(dbl))  [unwired: 5 in, 2 out]
                n557 = call-poly <vilib>:"DAQmx Write.vi"("task/channels in"=w873, "data"=w871, "error in"=w866) -> ("task out"=w872:refnum<k21>, "error out"=w865:errorcluster)  [unwired: 10 in, 1 out]
                n558 = call <vilib>:"DAQmx Start Task.vi"("task/channels in"=w872, "error in"=w865) -> ("task out"=w868:refnum<k21>, "error out"=w864:errorcluster)  [unwired: 12 in]
              }
              frame True {
                n559 = call <vilib>:"DAQmx Stop Task.vi"("task/channels in"=w884, "error in"=w881) -> ("task out"=w886:refnum<k21>, "error out"=w880:errorcluster)  [unwired: 12 in]
                n560 = property on="EPD-DC Power" class="Bool (strict)"("DisabledEnum"=T9."Disabled and Grayed Out" ("Disabled")) -> ()  [unwired: 2 in, 2 out]
                n561 = call-poly <vilib>:"DAQmx Write.vi"("task/channels in"=w886, "data"=w882, "error in"=w880) -> ("task out"=w885:refnum<k21>, "error out"=w879:errorcluster)  [unwired: 10 in, 1 out]
                n562 = call <vilib>:"DAQmx Start Task.vi"("task/channels in"=w885, "error in"=w879) -> ("task out"=w883:refnum<k21>, "error out"=w878:errorcluster)  [unwired: 12 in]
              }
            }
          }
        }
        n563 = local read "stop"() -> (w802:bool)
      }
      n564 = while {
        tunnel: w405 -> [w1715]
        tunnel: w404 -> [w1716]
        tunnel: [w1721] -> w403
        tunnel: [w1720] -> w402
        tunnel: [w1718] -> w401
        tunnel: w400 -> [w1714]
        tunnel: w380 -> [w1711]
        tunnel: [w1710] -> w399
        tunnel: [w1709] -> w392
        tunnel: w386 -> [w1707]
        tunnel: [w1706] -> w385
        stop <- "stop" stop-if-true
        # "Video Acquisition Loop"
        n565 = event shown="[6] \"AOBD GO\": Value Change" {
          selector: _ -> [_ _ _ _ _ _ _]
          dyn-events: _ -> [_ _ _ _ _ _ _]
          timeout: 1 -> [_ _ _ _ _ _ _]
          tunnel: w1716 -> [w1733 w1780 w1826 w1852 w1922 w1945 _]
          tunnel: w1715 -> [w1732 w1779 w1825 w1851 w1921 w1944 _]
          tunnel: w1714 -> [_ w1778 w1824 w1850 _ _ _]
          tunnel: [w1733 w1782 w1828 w1854 w1920 w1945 _] -> w1713
          tunnel: [w1732 w1781 w1827 w1853 w1919 w1944 _] -> w1712
          tunnel: w1711 -> [_ w1740 w1811 w1845 _ w1947 w1986]
          tunnel: [_ w1740 w1811 w1845 _ w1947 _] -> w1710
          tunnel: w1707 -> [_ w1738 w1807 w1844 _ w1942 w1982]
          tunnel: [_ w1738 w1807 w1844 _ w1943 w1981] -> w1706
          event Timeout {
            n566 = event-data() -> ()  [unwired: 1 in, 3 out]
          }
          event "Camera Zoom Level - DEPRECATED": Value Change {
            w1760 = "CameraAttributes::AcquisitionControl::ExposureTime"
            n567 = event-data() -> ("OldVal"=w1773:T4, "NewVal"=w1739:T4)  [unwired: 1 in, 4 out]
            n568 = call <vilib>:"IMAQdx Unconfigure Acquisition.vi"("error in"=w1779, "Session In"=w1780) -> ("error out"=w1776:errorcluster, "Session Out"=w1777:T8)  [unwired: 8 in]
            n569 = local read "Camera Zoom Level - DEPRECATED"() -> (w1736:T4)
            n570 = local read "zoom array"() -> (w1766:i32[])
            n571 = local read "zoom array"() -> (w1765:i32[])
            n572 = local read "FOV array"() -> (w1755:i32[])
            n573 = Index Array(array=w1755, index=w1739) -> (element=w1754:i32)
            n574 = local write "FOV (um)"(w1754) -> ()
            n575 = property class="IMAQdx"(reference=w1777, error in=w1776, "OffsetX"=u32 0, "OffsetY"=u32 0) -> (reference out=w1770:T8, error out=w1769:errorcluster)
            n576 = local read "FOV array"() -> (w1735:i32[])
            n577 = Index Array(array=w1766, index=w1773) -> (element=w1764:i32)
            n578 = Index Array(array=w1765, index=w1739) -> (element=w1741:i32)
            n579 = local read "2x binning"() -> (w1734:bool)
            n580 = Index Array(array=w1735, index=w1736) -> (element=w1737:i32)
            n581 = case shown="True" w1734 {
              tunnel: w1737 -> [w1786 w1787]
              frame False {
                n582 = local write "FOV (um)"(w1786) -> ()
              }
              frame True {
                n583 = Divide(x=w1787, y=2.0) -> (x/y=w1788:dbl)
                n584 = local write "FOV (um)"(w1788) -> ()
              }
            }
            n585 = Divide(x=w1741, y=w1764) -> (x/y=w1756:dbl)
            n586 = Subtract(x=1224, y=w1741) -> (x-y=w1748:i32)
            n587 = Subtract(x=1024, y=w1741) -> (x-y=w1749:i32)
            n588 = Divide(x=w1748, y=2) -> (x/y=w1743:dbl)
            n589 = Divide(x=w1749, y=2) -> (x/y=w1742:dbl)
            n590 = property class="IMAQdx"(reference=w1770, error in=w1769, "Width"=w1741, "Height"=w1741, "OffsetX"=w1743, "OffsetY"=w1742, "ActiveAttribute"=w1760) -> (reference out=w1759:T8, error out=w1758:errorcluster, "ValueDBL"=w1763:dbl)
            n591 = Multiply(x=w1756, y=w1763) -> (x*y=w1762:dbl)
            n592 = To Unsigned Word Integer(number=w1762) -> (unsigned 16bit integer=w1761:u16)
            n593 = case "Boundary Conditions" shown="..5" w1761 {
              selector: w1761 -> [w1790 _ _]
              tunnel: [w1790 5 4670] -> w1757
              frame Default {
              }
              frame ..5 {
              }
              frame 4670.. {
              }
            }
            n594 = local write "X"(w1741) -> ()
            n595 = local write "Y"(w1741) -> ()
            n596 = property on="Main Intensity" class="IntGraph (strict)"("XScale.Minimum"=0.0 ("Z Scale.Range:Maximum"), "YScale.Minimum"=0.0 ("Z Scale.Range:Minimum"), "XScale.Maximum"=w1741, "YScale.Maximum"=w1741) -> ()  [unwired: 2 in, 2 out]
            n597 = property class="IMAQdx"(reference=w1759, error in=w1758, "ActiveAttribute"=w1760, "ValueDBL"=w1757) -> (reference out=w1775:T8, error out=w1774:errorcluster)
            n598 = local write "Exposure Time (us)"(w1757) -> ()
            n599 = Initialize Array(0.0 ("element"), w1741, w1741) -> (w1750:dbl[][])
            n600 = Initialize Array(0.0 ("element"), w1741, w1741) -> (w1751:dbl[][])
            n601 = call <vilib>:"IMAQdx Configure Ring Acquisition.vi"("Mode"=IMAQdx_Acquisition_Mode."Continuous", "error in"=w1774, "Images"=w1778, "Session In"=w1775) -> ("error out"=w1785:errorcluster, "Session Out"=w1784:T8)  [unwired: 5 in, 1 out]
            n602 = local write "Ratio Stack 2"(w1751) -> ()
            n603 = local write "Ratio Stack 1"(w1750) -> ()
            n604 = call <vilib>:"IMAQdx Start Acquisition.vi"("error in"=w1785, "Session In"=w1784) -> ("error out"=w1781:errorcluster, "Session Out"=w1782:T8)  [unwired: 8 in]
          }
          event "Camera pixels": Value Change {
            n605 = event-data() -> ("NewVal"=w1808:string)  [unwired: 1 in, 5 out]
            n606 = call <vilib>:"IMAQdx Unconfigure Acquisition.vi"("error in"=w1825, "Session In"=w1826) -> ("error out"=w1822:errorcluster, "Session Out"=w1823:T8)  [unwired: 8 in]
            n607 = local read "2x binning"() -> (w1800:bool)
            n608 = property class="IMAQdx"(reference=w1823, error in=w1822, "OffsetX"=u32 0, "OffsetY"=u32 0) -> (reference out=w1819:T8, error out=w1818:errorcluster)
            n609 = case shown="True" w1800 {
              tunnel: [1 2] -> w1799
              frame False {
              }
              frame True {
              }
            }
            n610 = Decimal String To Number(string=w1808) -> (number=w1794:i32)  [unwired: 2 in, 1 out]
            n611 = local read "nm/pixel\n(binned)"() -> (w1795:dbl)
            n612 = Greater?(x=w1794, y=512) -> (0:w1805:bool)
            n613 = case shown="False" w1805 {
              frame False {
                n614 = property on="2x binning" class="Bool (strict)"("DisabledEnum"=T9."Enabled" ("Disabled")) -> ()  [unwired: 2 in, 2 out]
              }
              frame True {
                n615 = property on="2x binning" class="Bool (strict)"("DisabledEnum"=T9."Disabled and Grayed Out" ("Disabled")) -> ()  [unwired: 2 in, 2 out]
              }
            }
            n616 = call "SUBVI_get_pixel_sensor_offset.vi"("vertical binning"=w1799, "y dim"=w1794, "horizontal binning"=w1799, "x dim"=w1794, "max height"=1100, "max width"=1600) -> ("y offset"=w1801:dbl, "x offset"=w1802:dbl)  [unwired: 4 in]
            n617 = Multiply(x=w1794, y=w1795) -> (x*y=w1796:dbl)
            n618 = local write "offsetx"(w1802) -> ()
            n619 = local write "offsety"(w1801) -> ()
            n620 = Divide(x=w1796, y=1000.0) -> (x/y=w1798:dbl)
            n621 = property class="IMAQdx"(reference=w1819, error in=w1818, "Width"=w1794, "Height"=w1794, "OffsetX"=w1802, "OffsetY"=w1801) -> (reference out=w1810:T8, error out=w1809:errorcluster)
            n622 = local write "FOV (um)"(w1798) -> ()
            n623 = local write "X"(w1794) -> ()
            n624 = local write "Y"(w1794) -> ()
            n625 = property on="Main Intensity" class="IntGraph (strict)"("XScale.Minimum"=0.0 ("Z Scale.Range:Maximum"), "YScale.Minimum"=0.0 ("Z Scale.Range:Minimum"), "XScale.Maximum"=w1794, "YScale.Maximum"=w1794) -> ()  [unwired: 2 in, 2 out]
            n626 = property on="Refresh" class="Bool (strict)"("Val(Sgnl)"=TRUE ("Value (Signaling)")) -> ()  [unwired: 2 in, 2 out]
            n627 = Initialize Array(0.0 ("element"), w1794, w1794) -> (w1812:dbl[][])
            n628 = Initialize Array(0.0 ("element"), w1794, w1794) -> (w1813:dbl[][])
            n629 = call <vilib>:"IMAQdx Configure Ring Acquisition.vi"("Mode"=IMAQdx_Acquisition_Mode."Continuous", "error in"=w1809, "Images"=w1824, "Session In"=w1810) -> ("error out"=w1831:errorcluster, "Session Out"=w1830:T8)  [unwired: 5 in, 1 out]
            n630 = local write "Ratio Stack 2"(w1813) -> ()
            n631 = local write "Ratio Stack 1"(w1812) -> ()
            n632 = call <vilib>:"IMAQdx Start Acquisition.vi"("error in"=w1831, "Session In"=w1830) -> ("error out"=w1827:errorcluster, "Session Out"=w1828:T8)  [unwired: 8 in]
          }
          event "2x binning": Value Change {
            n633 = event-data() -> ("NewVal"=w1837:bool)  [unwired: 1 in, 5 out]
            n634 = call <vilib>:"IMAQdx Unconfigure Acquisition.vi"("error in"=w1851, "Session In"=w1852) -> ("error out"=w1848:errorcluster, "Session Out"=w1849:T8)  [unwired: 8 in]
            n635 = local read "Camera pixels"() -> (w1843:string)
            n636 = property class="IMAQdx"(reference=w1849, error in=w1848, "OffsetX"=u32 0, "OffsetY"=u32 0) -> (reference out=w1842:T8, error out=w1839:errorcluster)
            n637 = Decimal String To Number(string=w1843) -> (number=w1838:i32)  [unwired: 2 in, 1 out]
            n638 = case shown="True" w1837 {
              tunnel: w1842 -> [w1883 w1903]
              tunnel: w1838 -> [w1870 w1888]
              tunnel: [w1873 w1893] -> w1841
              tunnel: [w1872 w1892] -> w1840
              tunnel: w1839 -> [w1871 w1891]
              frame True {
                w1878 = 2
                n639 = property class="IMAQdx"(reference=w1883, error in=w1871, "ActiveAttribute"="CameraAttributes::ImageFormatControl::BinningHorizontal", "ValueDBL"=w1878, "ActiveAttribute"="CameraAttributes::ImageFormatControl::BinningVertical", "ValueDBL"=w1878) -> (reference out=w1875:T8, error out=w1874:errorcluster)
                n640 = call "SUBVI_get_pixel_sensor_offset.vi"("vertical binning"=w1878, "y dim"=w1870, "horizontal binning"=w1878, "x dim"=w1870, "max height"=1100.0, "max width"=1600.0) -> ("y offset"=w1876:dbl, "x offset"=w1877:dbl)  [unwired: 4 in]
                n641 = local write "offsety"(w1876) -> ()
                n642 = local write "offsetx"(w1877) -> ()
                n643 = property class="IMAQdx"(reference=w1875, error in=w1874, "Width"=w1870, "Height"=w1870, "OffsetX"=w1877, "OffsetY"=w1876) -> (reference out=w1872:T8, error out=w1873:errorcluster)
                n644 = Initialize Array(0.0 ("element"), w1870, w1870) -> (w1887:dbl[][])
                n645 = Initialize Array(0.0 ("element"), w1870, w1870) -> (w1886:dbl[][])
                n646 = local write "Y"(w1870) -> ()
                n647 = local write "X"(w1870) -> ()
                n648 = local write "Ratio Stack 2"(w1886) -> ()
                n649 = local write "Ratio Stack 1"(w1887) -> ()
              }
              frame False {
                w1898 = 1
                n650 = property class="IMAQdx"(reference=w1903, error in=w1891, "ActiveAttribute"="CameraAttributes::ImageFormatControl::BinningHorizontal", "ValueDBL"=w1898, "ActiveAttribute"="CameraAttributes::ImageFormatControl::BinningVertical", "ValueDBL"=w1898) -> (reference out=w1895:T8, error out=w1894:errorcluster)
                n651 = call "SUBVI_get_pixel_sensor_offset.vi"("vertical binning"=w1898, "y dim"=w1888, "horizontal binning"=w1898, "x dim"=w1888, "max height"=1100.0, "max width"=1600.0) -> ("y offset"=w1896:dbl, "x offset"=w1897:dbl)  [unwired: 4 in]
                n652 = local write "offsety"(w1896) -> ()
                n653 = local write "offsetx"(w1897) -> ()
                n654 = local write "Y"(w1888) -> ()
                n655 = local write "X"(w1888) -> ()
                n656 = property class="IMAQdx"(reference=w1895, error in=w1894, "Width"=w1888, "Height"=w1888, "OffsetX"=w1897, "OffsetY"=w1896) -> (reference out=w1892:T8, error out=w1893:errorcluster)
                n657 = Initialize Array(0.0 ("element"), w1888, w1888) -> (w1907:dbl[][])
                n658 = Initialize Array(0.0 ("element"), w1888, w1888) -> (w1906:dbl[][])
                n659 = property on="Main Intensity" class="IntGraph (strict)"("XScale.Minimum"=0.0 ("Z Scale.Range:Maximum"), "YScale.Minimum"=0.0 ("Z Scale.Range:Minimum"), "XScale.Maximum"=w1888, "YScale.Maximum"=w1888) -> ()  [unwired: 2 in, 2 out]
                n660 = local write "Ratio Stack 2"(w1906) -> ()
                n661 = local write "Ratio Stack 1"(w1907) -> ()
              }
            }
            n662 = case "Calculate FOV" shown="False" w1837 {
              tunnel: w1838 -> [w1859 w1863]
              frame False {
                # "If 2x binning is off then native nm/px = binned nm/px"
                n663 = local read "nm/pixel\n(native)"() -> (w1858:dbl)
                n664 = local write "nm/pixel\n(binned)"(w1858) -> ()
                n665 = Multiply(x=w1859, y=w1858) -> (x*y=w1861:dbl)
                n666 = Divide(x=w1861, y=1000.0) -> (x/y=w1862:dbl)
                n667 = local write "FOV (um)"(w1862) -> ()
              }
              frame True {
                # "if 2x binning is on the nm/px is doubled"
                n668 = local read "nm/pixel\n(native)"() -> (w1867:dbl)
                n669 = Multiply(x=2.0 ("y"), y=w1867) -> (x*y=w1866:dbl)
                n670 = local write "nm/pixel\n(binned)"(w1866) -> ()
                n671 = Multiply(x=w1863, y=w1866) -> (x*y=w1868:dbl)
                n672 = Divide(x=w1868, y=1000.0) -> (x/y=w1869:dbl)
                n673 = local write "FOV (um)"(w1869) -> ()
              }
            }
            n674 = property on="Refresh" class="Bool (strict)"("Val(Sgnl)"=TRUE ("Value (Signaling)")) -> ()  [unwired: 2 in, 2 out]
            n675 = call <vilib>:"IMAQdx Configure Ring Acquisition.vi"("Mode"=IMAQdx_Acquisition_Mode."Continuous", "error in"=w1841, "Images"=w1850, "Session In"=w1840) -> ("error out"=w1857:errorcluster, "Session Out"=w1856:T8)  [unwired: 5 in, 1 out]
            n676 = call <vilib>:"IMAQdx Start Acquisition.vi"("error in"=w1857, "Session In"=w1856) -> ("error out"=w1853:errorcluster, "Session Out"=w1854:T8)  [unwired: 8 in]
          }
          event "get camera info": Value Change {
            n677 = event-data() -> ()  [unwired: 1 in, 6 out]
            n678 = property class="IMAQdx"(reference=w1922, error in=w1921, "ActiveAttribute"="CameraAttributes::AcquisitionControl::ExposureTime", "ActiveAttribute"="CameraAttributes::AcquisitionControl::AcquisitionFrameRate", "ActiveAttribute"="CameraAttributes::ImageFormatControl::Width", "ActiveAttribute"="CameraAttributes::ImageFormatControl::Height", "ActiveAttribute"="CameraAttributes::ImageFormatControl::OffsetX", "ActiveAttribute"="CameraAttributes::ImageFormatControl::OffsetY", "ActiveAttribute"="CameraAttributes::ImageFormatControl::BinningHorizontal", "ActiveAttribute"="CameraAttributes::ImageFormatControl::BinningVertical") -> (reference out=w1920:T8, error out=w1919:errorcluster, "ValueDBL"=w1912:dbl, "ValueDBL"=w1909:dbl, "ValueDBL"=w1915:dbl, "ValueDBL"=w1916:dbl, "ValueDBL"=w1918:dbl, "ValueDBL"=w1917:dbl, "ValueDBL"=w1914:dbl, "ValueDBL"=w1913:dbl)
            n679 = local write "get camera info"(FALSE ("get camera info")) -> ()
            n680 = local write "frame rate"(w1909) -> ()
            n681 = local write "exp time"(w1912) -> ()
            n682 = local write "binning vertical"(w1913) -> ()
            n683 = local write "binning horizontal"(w1914) -> ()
            n684 = local write "width"(w1915) -> ()
            n685 = local write "offsety"(w1917) -> ()
            n686 = local write "height"(w1916) -> ()
            n687 = local write "offsetx"(w1918) -> ()
            n688 = Divide(x=1000000.0, y=w1909) -> (x/y=w1908:dbl)
            n689 = local write "sync exp"(w1908) -> ()
          }
          event "Laser Zoom Level": Value Change {
            n690 = event-data() -> ("NewVal"=w1946:T3)  [unwired: 1 in, 5 out]
            n691 = flat-sequence {
              tunnel: [w1953] -> w1941
              tunnel: [u32 200 ("milliseconds to wait")] -> w1939
              tunnel: w1947 -> [w1951]
              tunnel: w1946 -> [w1950]
              tunnel: [w1949] -> w1937
              tunnel: w1942 -> [w1948]
              tunnel: w1941 -> [w1957]
              tunnel: [w1957] -> w1940
              tunnel: w1939 -> [w1955]
              tunnel: [w1955] -> w1938
              tunnel: w1937 -> [w1956]
              tunnel: [w1956] -> w1936
              tunnel: [w1962] -> w1935
              tunnel: w1940 -> [w1961]
              tunnel: w1938 -> [w1960]
              tunnel: [w1960] -> w1933
              tunnel: w1936 -> [w1959]
              tunnel: [w1958] -> w1932
              tunnel: w1935 -> [w1967]
              tunnel: [w1967] -> w1934
              tunnel: w1933 -> [w1965]
              tunnel: w1932 -> [w1966]
              tunnel: [w1966] -> w1931
              tunnel: w1934 -> [w1970]
              tunnel: w1931 -> [w1969]
              tunnel: [w1968] -> w1943
              frame #0 {
                w1954 = u16 0 items=["Recall", "Save"] ("Operation (0: Recall)")
                n692 = call <instrlib>:"Recall Save Instrument Settings.vi"("error in (no error)"=w1948, "Setup Memory Location (0)"=w1950, "Operation (0: Recall)"=w1954, "VISA resource name"=w1951) -> ("error out"=w1949:errorcluster, "VISA resource name out"=w1953:refnum<visa-resource-name>)  [unwired: 6 in]
              }
              frame #1 {
                n693 = Wait (ms)(milliseconds to wait=w1955) -> ()  [unwired: 1 out]
              }
              frame #2 {
                w1963 = u16 1 items=["Channel 1"=1, "Channel2"=2] ("Channel (1: Channel 1)")
                n694 = call <instrlib>:"Enable Output.vi"("Enable Output (T: Enable)"=TRUE, "error in (no error)"=w1959, "Channel (1: Channel 1)"=w1963, "VISA resource name"=w1961) -> ("error out"=w1958:errorcluster, "VISA resource name out"=w1962:refnum<visa-resource-name>)  [unwired: 6 in]
              }
              frame #3 {
                n695 = Wait (ms)(milliseconds to wait=w1965) -> ()  [unwired: 1 out]
              }
              frame #4 {
                w1971 = u16 2 items=["Channel 1"=1, "Channel2"=2] ("Channel (1: Channel 1)")
                n696 = call <instrlib>:"Enable Output.vi"("Enable Output (T: Enable)"=TRUE, "error in (no error)"=w1969, "Channel (1: Channel 1)"=w1971, "VISA resource name"=w1970) -> ("error out"=w1968:errorcluster)  [unwired: 6 in, 1 out]
              }
            }
          }
          event "AOBD GO": Value Change {
            w1974 = u16 2 items=["Channel 1"=1, "Channel 2"=2] ("Channel (1 Channel 1)")
            w1985 = u16 1 items=["Channel 1"=1, "Channel 2"=2] ("Channel (1 Channel 1)")
            n697 = event-data() -> ()  [unwired: 1 in, 6 out]
            n698 = local write "AOBD GO"(FALSE ("AOBD GO")) -> ()
            n699 = local read "AOBD W"() -> (w1983:dbl)
            n700 = local read "AOBD X"() -> (w1984:dbl)
            n701 = call <instrlib>:"Configure Waveform.vi"("Frequency (1000 Hz)"=74000.0, "DC Offset (0.00 V)"=w1984, "error in (no error)"=w1982, "Amplitude (1 Vpp)"=w1983, "Channel (1 Channel 1)"=w1985, "VISA resource name"=w1986) -> ("error out"=w1980:errorcluster, "VISA resource name out"=w1975:refnum<visa-resource-name>)  [unwired: 4 in]
            n702 = local read "AOBD W"() -> (w1976:dbl)
            n703 = local read "AOBD Y"() -> (w1979:dbl)
            n704 = call <instrlib>:"Configure Waveform.vi"("Frequency (1000 Hz)"=91000.0, "DC Offset (0.00 V)"=w1979, "error in (no error)"=w1980, "Amplitude (1 Vpp)"=w1976, "Channel (1 Channel 1)"=w1974, "VISA resource name"=w1975) -> ("error out"=w1981:errorcluster)  [unwired: 4 in, 1 out]
          }
        }
        n705 = flat-sequence {
          frame #0 {
            n706 = local read "t1"() -> (w1728:dbl)
            n707 = local read "t2"() -> (w1729:dbl)
            n708 = Subtract(x=w1729, y=w1728) -> (x-y=w1727:dbl)
            n709 = Reciprocal(x=w1727) -> (1/x=→"fps 2":dbl)
          }
          frame #1 {
            n710 = local read "t2"() -> (w1730:dbl)
            n711 = local write "t1"(w1730) -> ()
          }
          frame #2 {
            n712 = call <vilib>:"High Resolution Relative Seconds.vi"() -> ("relative seconds"=w1731:dbl)
            n713 = local write "t2"(w1731) -> ()
          }
        }
        n714 = call <vilib>:"IMAQdx Get Image Data.vi"("Buffer Number Mode (Next)"=IMAQdx_Buffer_Number_Mode."Last New", "error in"=w1712, "Session In"=w1713) -> ("error out"=w1721:errorcluster, "Buffer Number Out"=→"Buffer Number Out":u32, "Image Data Array"=w1708:u8[], "Session Out"=w1720:T8)  [unwired: 5 in]
        n715 = call <extravilib>:"Write.vi"("element"=w1708) -> ("channel"=w1709:T14)  [unwired: 8 in, 2 out]
        n716 = local read "RECORD / STOP VIDEO"() -> (w1724:bool)
        n717 = local read "Save Raw Binary"() -> (w1725:bool)
        n718 = And(x=w1724, y=w1725) -> (x .and. y?=w1723:bool)
        n719 = case shown="True" w1723 {
          tunnel: w1708 -> [_ w1988]
          tunnel: [_ w1987] -> w1718
          frame False {
          }
          frame True {
            # "IF WE ARE SAVING A RAW BIN FILE, OUTPUT THE CHANNEL WRITER TO THE RAW BIN WRITER"
            n720 = call <extravilib>:"Write.vi"("element"=w1988) -> ("channel"=w1987:T14)  [unwired: 8 in, 2 out]
          }
        }
      }
      n721 = while {
        tunnel: [w912] -> w394
        tunnel: [w911] -> w393
        shift-right: [w899] -> w396
        shift-left: w398 -> [w915]
        shift-right: [w913] -> w395
        shift-left: w397 -> [w914]
        tunnel: w392 -> [w908]
        tunnel: w373 -> [w888]
        stop <- w909 stop-if-true
        # "VIDEO DISPLAY LOOP"
        n722 = call <extravilib>:"Read.vi"("channel"=w908) -> ("element"=w901:u8[])  [unwired: 6 in, 4 out]
        n723 = local read "X"() -> (w898:dbl)
        n724 = local read "Y"() -> (w897:dbl)
        n725 = Reshape Array(w901, w897, w898) -> (w902:u8[][])
        n726 = local read "Gain (dB)"() -> (w894:dbl)
        n727 = local read "exp time"() -> (w895:dbl)
        n728 = local read "sync exp"() -> (w896:dbl)
        n729 = call <vilib>:"High Resolution Relative Seconds.vi"() -> ("relative seconds"=w904:dbl)
        n730 = Not Equal To 0?(x=w894) -> (x != 0?=→"Gain Warning":bool)
        n731 = Greater?(x=w895, y=w896) -> (0:→"sync exp warning":bool)
        n732 = event shown="[0] Timeout" {
          selector: _ -> [_ _ _ _ _ _ _ _]
          dyn-events: _ -> [_ _ _ _ _ _ _ _]
          timeout: 1 -> [_ _ _ _ _ _ _ _]
          tunnel: w915 -> [w938 w1110 w1120 w1136 w1156 w1174 w1181 w1190]
          tunnel: w914 -> [w942 w1109 w1119 w1134 w1154 w1175 w1180 w1189]
          tunnel: [w941 w1110 w1120 w1132 w1143 w1173 w1179 w1190] -> w899
          tunnel: [w940 w1109 w1119 w1131 w1141 w1172 w1178 w1189] -> w913
          tunnel: [w937 _ _ _ _ _ _ _] -> w912
          tunnel: [w936 _ _ _ _ _ _ _] -> w911
          tunnel: w902 -> [w935 _ _ _ _ _ _ _]
          tunnel: w888 -> [w934 _ _ _ _ _ _ _]
          event Timeout {
            n733 = event-data() -> ()  [unwired: 1 in, 3 out]
            n734 = case shown="False" "Ratiometric?" {
              tunnel: w938 -> [w951 w995]
              tunnel: w942 -> [w950 w986]
              tunnel: [w951 w987] -> w941
              tunnel: [w950 w992] -> w940
              tunnel: [_ w991] -> w937
              tunnel: [_ w990] -> w936
              tunnel: w935 -> [w944 w988]
              tunnel: w934 -> [w943 w985]
              frame False {
                n735 = local read "bg timer"() -> (w946:u32)
                n736 = Greater?(x=w946, y=0.0) -> (0:w948:bool)
                n737 = case shown="True" w948 {
                  tunnel: w944 -> [_ w965]
                  frame False {
                  }
                  frame True {
                    n738 = local read "bg timer"() -> (w973:u32)
                    n739 = Tick Count (ms)() -> (millisecond timer value=w974:u32)
                    n740 = local write "bg array sum"(w965) -> ()
                    n741 = Subtract(x=w974, y=w973) -> (x-y=w970:u32)
                    n742 = Subtract(x=u32 3000, y=w970) -> (x-y=w968:u32)
                    n743 = Greater?(x=w970, y=u32 2999) -> (0:w971:bool)
                    n744 = Divide(x=w968, y=u32 1000) -> (x/y=w966:dbl)
                    n745 = case shown="True" w971 {
                      frame False {
                      }
                      frame True {
                        n746 = local write "bg countdown"(0.0 ("bg countdown")) -> ()
                        n747 = local write "acquiring bg"(TRUE ("acquiring background")) -> ()
                        n748 = local write "bg timer"(u32 0 ("bg timer")) -> ()
                        "n bg frames" <- 0
                      }
                    }
                    n749 = local write "bg countdown"(w966) -> ()
                  }
                }
                n750 = local read "acquiring bg"() -> (w945:bool)
                n751 = case shown="True" w945 {
                  tunnel: w944 -> [_ w955]
                  frame False {
                  }
                  frame True {
                    n752 = local read "bg array sum"() -> (w958:dbl[][])
                    n753 = local read "n bg frames"() -> (w956:i32)
                    n754 = Add(x=w955, y=w958) -> (x+y=w957:dbl[][])
                    n755 = local write "bg array sum"(w957) -> ()
                    n756 = Increment(x=w956) -> (x+1=w952:i32)
                    n757 = Equal?(x=1000.0, y=w952) -> (x = y?=w954:bool)
                    n758 = local write "n bg frames"(w952) -> ()
                    n759 = case shown="True" w954 {
                      frame False {
                      }
                      frame True {
                        n760 = flat-sequence {
                          frame #0 {
                            n761 = local read "bg array sum"() -> (w961:dbl[][])
                            n762 = local read "n bg frames"() -> (w959:i32)
                            n763 = Divide(x=w961, y=w959) -> (x/y=w960:dbl[][])
                            "bg array" <- w960
                            n764 = local write "acquiring bg"(FALSE ("acquiring background")) -> ()
                            n765 = local write "acquire bg"(FALSE ("acquire background")) -> ()
                            n766 = local write "bg array sum"(w960) -> ()
                          }
                          frame #1 {
                            n767 = local write "n bg frames"(0 ("Numeric 2")) -> ()
                          }
                        }
                      }
                    }
                  }
                }
                n768 = local read "apply bg removal"() -> (w949:bool)
                n769 = case shown="False" w949 {
                  tunnel: w944 -> [w980 w984]
                  tunnel: w943 -> [w981 _]
                  frame False {
                    n770 = local write "Main Intensity"(w980) -> ()
                    n771 = call "IMAQ ArrayToImage"("Image Pixels (U8)"=w980, "Image"=w981) -> ("Image Out"=w979:T1)  [unwired: 8 in, 1 out]
                    n772 = local write "Image"(w979) -> ()
                  }
                  frame True {
                    n773 = local read "bg array"() -> (w983:dbl[][])
                    n774 = Divide(x=w984, y=w983) -> (x/y=w982:dbl[][])
                    n775 = local write "Main Intensity"(w982) -> ()
                  }
                }
              }
              frame True {
                # "Ratiometric Mode has been Turned On"
                n776 = Lossy Enqueue Element(queue=w995, element=w988) -> (queue out=w987:refnum<queue>, overflow element=w993:dbl[][], overflow?=w994:bool, error out=w991:errorcluster)  [unwired: 1 in]
                n777 = case shown="True" w994 {
                  tunnel: w986 -> [w1003 w1013]
                  tunnel: w993 -> [_ w1007]
                  tunnel: [w1003 w1012] -> w992
                  tunnel: [_ w1009] -> w990
                  tunnel: w988 -> [w998 w1008]
                  tunnel: w987 -> [_ w1006]
                  tunnel: w986 -> [_ w1005]
                  tunnel: w985 -> [_ w1004]
                  frame False {
                    # "Waiting for Stack 1 to fill"
                    n778 = local read "Ratio Stack 1"() -> (w1000:dbl[][])
                    n779 = local read "Boolean"() -> (w1002:bool)
                    n780 = Not(x=w1002) -> (.not. x?=→"Boolean":bool)
                    n781 = Add(x=w998, y=w1000) -> (x+y=w999:dbl[][])
                    n782 = local write "Ratio Stack 1"(w999) -> ()
                  }
                  frame True {
                    # "Stack 1 has been filled"
                    n783 = Lossy Enqueue Element(queue=w1013, element=w1007) -> (queue out=w1012:refnum<queue>, overflow element=w1010:dbl[][], overflow?=w1011:bool, error out=w1009:errorcluster)  [unwired: 1 in]
                    n784 = case shown="True" w1011 {
                      tunnel: w1007 -> [w1023 w1053]
                      tunnel: w1007 -> [w1021 w1054]
                      tunnel: w1010 -> [_ w1052]
                      tunnel: w1008 -> [w1014 w1050]
                      tunnel: w1006 -> [_ w1049]
                      tunnel: w1005 -> [_ w1048]
                      tunnel: w1004 -> [_ w1024]
                      frame False {
                        # "Waiting for Stack 2 to fill"
                        n785 = local read "Ratio Stack 1"() -> (w1015:dbl[][])
                        n786 = local read "Ratio Stack 2"() -> (w1017:dbl[][])
                        n787 = Add(x=w1014, y=w1015) -> (x+y=w1022:dbl[][])
                        n788 = Subtract(x=w1022, y=w1021) -> (x-y=w1016:dbl[][])
                        n789 = local read "Boolean 2"() -> (w1020:bool)
                        n790 = Add(x=w1023, y=w1017) -> (x+y=w1018:dbl[][])
                        n791 = local write "Ratio Stack 1"(w1016) -> ()
                        n792 = Not(x=w1020) -> (.not. x?=→"Boolean 2":bool)
                        n793 = local write "Ratio Stack 2"(w1018) -> ()
                      }
                      frame True {
                        # "Both Stacks Filled. Steady State Ratiometric"
                        n794 = disable-structure shown="Disabled" {
                          disable-tunnel: w1049 -> [w1073 _]
                          disable-tunnel: w1048 -> [w1072 _]
                          frame Disabled {
                            n795 = case shown="True" {
                              selector: _ -> [_ _]
                              tunnel: w1073 -> [_ w1089]
                              tunnel: w1072 -> [_ w1082]
                              frame False {
                              }
                              frame True {
                                n796 = Get Queue Status(queue=w1089, return elements? (F)=TRUE) -> (elements=w1088:cluster{dbl[][]}[])  [unwired: 1 in, 7 out]
                                n797 = Get Queue Status(queue=w1082, return elements? (F)=TRUE) -> (elements=w1083:cluster{dbl[][]}[])  [unwired: 1 in, 7 out]
                                n798 = local read "X"() -> (w1087:dbl)
                                n799 = local read "Y"() -> (w1086:dbl)
                                n800 = for {
                                tunnel: w1088 -> [w1099] mode=indexing
                                tunnel: [w1098] -> w1084 mode=indexing
                                n801 = Unbundle(w1099) -> (w1098:dbl[][])
                                }
                                n802 = for {
                                tunnel: w1083 -> [w1094] mode=indexing
                                tunnel: [w1093] -> w1081 mode=indexing
                                n803 = Unbundle(w1094) -> (w1093:dbl[][])
                                }
                                n804 = Initialize Array(0.0 ("element"), w1087, w1086) -> (w1080:dbl[][])
                                n805 = for {
                                tunnel: w1084 -> [w1097] mode=indexing
                                shift-right: [w1096] -> w1077
                                shift-left: w1080 -> [w1095]
                                n806 = Add(x=w1097, y=w1095) -> (x+y=w1096:dbl[][])
                                }
                                n807 = for {
                                tunnel: w1081 -> [w1090] mode=indexing
                                shift-right: [w1092] -> w1076
                                shift-left: w1080 -> [w1091]
                                n808 = Add(x=w1091, y=w1090) -> (x+y=w1092:dbl[][])
                                }
                                n809 = call <vilib>:"High Resolution Relative Seconds.vi"() -> ("relative seconds"=w1074:dbl)
                                n810 = Divide(x=w1077, y=w1076) -> (x/y=w1075:dbl[][])
                                n811 = local write "rt 2"(w1074) -> ()
                              }
                            }
                          }
                          frame Enabled {
                          }
                        }
                        n812 = local write "loading ratiometric stack"(FALSE ("loading ratiometric stack")) -> ()
                        n813 = local read "rt 2"() -> (w1035:dbl)
                        n814 = call <vilib>:"High Resolution Relative Seconds.vi"() -> ("relative seconds"=w1037:dbl)
                        n815 = Add(x=w1035, y=0.03) -> (x+y=w1036:dbl)
                        n816 = local read "Ratio Stack 1"() -> (w1041:dbl[][])
                        n817 = local read "Ratio Stack 2"() -> (w1040:dbl[][])
                        n818 = Greater?(x=w1037, y=w1036) -> (0:w1033:bool)
                        n819 = local read "Buffer Number Out"() -> (w1029:u32)
                        n820 = Add(x=w1053, y=w1040) -> (x+y=w1046:dbl[][])
                        n821 = Add(x=w1050, y=w1041) -> (x+y=w1047:dbl[][])
                        n822 = Subtract(x=w1047, y=w1054) -> (x-y=w1039:dbl[][])
                        n823 = Subtract(x=w1046, y=w1052) -> (x-y=w1038:dbl[][])
                        n824 = Quotient & Remainder(x=w1029, y=u32 200) -> (x-y*floor(x/y)=w1031:u32)  [unwired: 1 out]
                        n825 = local read "get noise"() -> (w1026:bool)
                        n826 = local write "Ratio Stack 2"(w1038) -> ()
                        n827 = Add Array Elements(numeric array=w1038) -> (sum=w1043:dbl)
                        n828 = Add Array Elements(numeric array=w1039) -> (sum=w1042:dbl)
                        n829 = Equal?(x=w1031, y=0.0) -> (x = y?=w1032:bool)
                        n830 = local write "Ratio Stack 1"(w1039) -> ()
                        n831 = Divide(x=w1039, y=w1042) -> (x/y=w1044:dbl[][])
                        n832 = And(x=w1032, y=w1026) -> (x .and. y?=w1027:bool)
                        n833 = Divide(x=w1038, y=w1043) -> (x/y=w1045:dbl[][])
                        n834 = Divide(x=w1044, y=w1045) -> (x/y=w1025:dbl[][])
                        n835 = case shown="True" w1027 {
                          tunnel: w1025 -> [_ w1056]
                          frame False {
                          }
                          frame True {
                            n836 = local read "X"() -> (w1061:dbl)
                            n837 = local read "Y"() -> (w1060:dbl)
                            n838 = Multiply(x=w1061, y=w1060) -> (x*y=w1059:dbl)
                            n839 = Reshape Array(w1056, w1059) -> (w1058:dbl[])
                            n840 = for {
                              tunnel: w1058 -> [w1063] mode=indexing
                              tunnel: [w1063] -> w1057 mode=indexing if=w1062
                              n841 = Not A Number/Path/Refnum?(number/path/refnum=w1063) -> (NaN/Path/Refnum?=w1065:bool)
                              n842 = Not(x=w1065) -> (.not. x?=w1066:bool)
                              n843 = Less?(x=w1063, y=2.0) -> (x < y?=w1067:bool)
                              n844 = And(x=w1066, y=w1067) -> (x .and. y?=w1062:bool)
                            }
                            n845 = call <vilib>:"Std Deviation and Variance.vi"("X"=w1057) -> ("standard deviation"=→"noise":dbl)  [unwired: 1 in, 2 out]
                          }
                        }
                        n846 = disable-structure shown="Disabled" {
                          disable-tunnel: w1025 -> [w1100 _]
                          frame Disabled {
                            n847 = local read "X"() -> (w1108:dbl)
                            n848 = local read "Y"() -> (w1107:dbl)
                            n849 = Multiply(x=w1108, y=w1107) -> (x*y=w1106:dbl)
                            n850 = Reshape Array(w1100, w1106) -> (w1105:dbl[])
                            n851 = Array Max & Min(array=w1100) -> (max value=→"max value":dbl, min value=→"min value":dbl)  [unwired: 2 out]
                            n852 = call <vilib>:"General Histogram.vi"("X"=w1105, "# bins"=256) -> ("Histogram Graph"=→"Histogram Graph":T5)  [unwired: 9 in, 4 out]
                          }
                          frame Enabled {
                          }
                        }
                        n853 = case shown="True" w1033 {
                          tunnel: w1025 -> [_ w1070]
                          tunnel: w1024 -> [_ w1068]
                          frame False {
                          }
                          frame True {
                            n854 = call "IMAQ ArrayToImage"("Image"=w1068) -> ("Image Out"=w1069:T1)  [unwired: 9 in, 1 out]
                            n855 = local write "Main Intensity"(w1070) -> ()
                            n856 = local write "Image"(w1069) -> ()
                            n857 = call <vilib>:"High Resolution Relative Seconds.vi"() -> ("relative seconds"=w1071:dbl)
                            n858 = local write "rt 2"(w1071) -> ()
                          }
                        }
                      }
                    }
                  }
                }
                n859 = local read "loading ratiometric stack"() -> (w989:bool)
                n860 = case shown="True" w989 {
                  frame False {
                  }
                  frame True {
                    n861 = local read "loading ratiometric"() -> (w996:dbl)
                    n862 = Increment(x=w996) -> (x+1=→"loading ratiometric":dbl)
                  }
                }
              }
            }
          }
          event "apply bg removal": Value Change {
            n863 = event-data() -> ("NewVal"=w1111:bool)  [unwired: 1 in, 5 out]
            n864 = case shown="True" w1111 {
              frame False {
                n865 = property on="Main Intensity" class="IntGraph (strict)"("ZScale.Maximum"=255.0 ("Z Scale.Range:Maximum"), "ZScale.Minimum"=0.0 ("Z Scale.Range:Minimum")) -> ()  [unwired: 2 in, 2 out]
              }
              frame True {
                n866 = local read "Dynamic Range"() -> (w1118:dbl)
                n867 = Add(x=1, y=w1118) -> (x+y=w1116:dbl)
                n868 = Subtract(x=1, y=w1118) -> (x-y=w1117:dbl)
                n869 = property on="Main Intensity" class="IntGraph (strict)"("ZScale.Maximum"=w1116, "ZScale.Minimum"=w1117) -> ()  [unwired: 2 in, 2 out]
              }
            }
          }
          event "acquire bg": Value Change {
            n870 = event-data() -> ("NewVal"=w1121:bool)  [unwired: 1 in, 5 out]
            n871 = case shown="True" w1121 {
              frame False {
              }
              frame True {
                n872 = Tick Count (ms)() -> (millisecond timer value=→"bg timer":u32)
              }
            }
          }
          event "Ratio Buffer Size": Value Change {
            n873 = event-data() -> ()  [unwired: 1 in, 6 out]
            n874 = Flush Queue(queue=w1134) -> (queue out=w1133:refnum<queue>)  [unwired: 1 in, 2 out]
            n875 = Flush Queue(queue=w1136) -> (queue out=w1135:refnum<queue>)  [unwired: 1 in, 2 out]
            n876 = Release Queue(queue=w1133) -> ()  [unwired: 2 in, 3 out]
            n877 = Release Queue(queue=w1135) -> ()  [unwired: 2 in, 3 out]
            n878 = local read "X"() -> (w1124:dbl)
            n879 = local read "Y"() -> (w1123:dbl)
            n880 = Initialize Array(0.0 ("element"), w1123, w1124) -> (w1126:dbl[][])
            n881 = Initialize Array(0.0 ("element"), w1123, w1124) -> (w1125:dbl[][])
            n882 = local write "Ratio Stack 1"(w1126) -> ()
            n883 = local write "Ratio Stack 2"(w1125) -> ()
            n884 = local read "Ratio Buffer Size"() -> (w1137:i32)
            n885 = Obtain Queue(max queue size (-1, unlimited)=w1137, name (unnamed)="front", element data type=w1126) -> (queue out=w1132:refnum<queue>)  [unwired: 2 in, 2 out]
            n886 = Obtain Queue(max queue size (-1, unlimited)=w1137, name (unnamed)="back", element data type=w1125) -> (queue out=w1131:refnum<queue>)  [unwired: 2 in, 2 out]
          }
          event "Paste Buffer": Value Change {
            n887 = event-data() -> ()  [unwired: 1 in, 6 out]
            n888 = Flush Queue(queue=w1154) -> (queue out=w1153:refnum<queue>)  [unwired: 1 in, 2 out]
            n889 = Flush Queue(queue=w1156) -> (queue out=w1155:refnum<queue>)  [unwired: 1 in, 2 out]
            n890 = Release Queue(queue=w1153) -> ()  [unwired: 2 in, 3 out]
            n891 = Release Queue(queue=w1155) -> ()  [unwired: 2 in, 3 out]
            n892 = local read "X"() -> (w1146:dbl)
            n893 = local read "Y"() -> (w1145:dbl)
            n894 = Initialize Array(0.0 ("element"), w1146, w1145) -> (w1148:dbl[][])
            n895 = Initialize Array(0.0 ("element"), w1146, w1145) -> (w1147:dbl[][])
            n896 = local write "Ratio Stack 1"(w1148) -> ()
            n897 = local write "Ratio Stack 2"(w1147) -> ()
            n898 = local read "Ratio Buffer Size"() -> (w1144:i32)
            n899 = Obtain Queue(max queue size (-1, unlimited)=w1144, name (unnamed)="front", element data type=w1148) -> (queue out=w1142:refnum<queue>)  [unwired: 2 in, 2 out]
            n900 = Obtain Queue(max queue size (-1, unlimited)=w1144, name (unnamed)="back", element data type=w1147) -> (queue out=w1140:refnum<queue>)  [unwired: 2 in, 2 out]
            n901 = local read "queue2 save"() -> (w1139:cluster{dbl[][]}[])
            n902 = local read "queue1 save"() -> (w1138:cluster{dbl[][]}[])
            n903 = for {
              N: w1144 -> [_]
              shift-right: [w1165] -> w1143
              shift-left: w1142 -> [w1164]
              tunnel: w1138 -> [w1162] mode=indexing
              i -> [w1163]
              n904 = Unbundle(w1162) -> (w1161:dbl[][])
              n905 = Enqueue Element(queue=w1164, element=w1161) -> (queue out=w1165:refnum<queue>)  [unwired: 2 in, 2 out]
              "Numeric" <- w1163
            }
            n906 = for {
              tunnel: w1139 -> [w1158] mode=indexing
              shift-right: [w1160] -> w1141
              shift-left: w1140 -> [w1159]
              n907 = Unbundle(w1158) -> (w1157:dbl[][])
              n908 = Enqueue Element(queue=w1159, element=w1157) -> (queue out=w1160:refnum<queue>)  [unwired: 2 in, 2 out]
            }
          }
          event "Copy Buffer": Value Change {
            n909 = event-data() -> ()  [unwired: 1 in, 6 out]
            n910 = Get Queue Status(queue=w1175, return elements? (F)=TRUE) -> (queue out=w1172:refnum<queue>, elements=→"queue2 save":cluster{dbl[][]}[])  [unwired: 1 in, 6 out]
            n911 = Get Queue Status(queue=w1174, return elements? (F)=TRUE) -> (queue out=w1173:refnum<queue>, # elements in queue=→"# elements in queue 2":i32, elements=w1166:cluster{dbl[][]}[])  [unwired: 1 in, 5 out]
            "queue1 save" <- w1166
            n912 = Array Size(array=w1166) -> (size(s)=→"size(s)":i32)
            "copy buffer" <- TRUE ("Boolean 3")
          }
          event "Camera Zoom Level - DEPRECATED": Value Change {
            n913 = event-data() -> ()  [unwired: 1 in, 6 out]
            n914 = Flush Queue(queue=w1180) -> (queue out=w1182:refnum<queue>)  [unwired: 1 in, 2 out]
            n915 = Flush Queue(queue=w1181) -> (queue out=w1177:refnum<queue>)  [unwired: 1 in, 2 out]
            n916 = Release Queue(queue=w1182) -> ()  [unwired: 2 in, 3 out]
            n917 = Release Queue(queue=w1177) -> ()  [unwired: 2 in, 3 out]
            n918 = local read "Ratio Buffer Size"() -> (w1187:i32)
            n919 = local read "Ratio Stack 1"() -> (w1185:dbl[][])
            n920 = local read "Ratio Stack 2"() -> (w1186:dbl[][])
            n921 = Obtain Queue(max queue size (-1, unlimited)=w1187, name (unnamed)="front", element data type=w1185) -> (queue out=w1179:refnum<queue>)  [unwired: 2 in, 2 out]
            n922 = Obtain Queue(max queue size (-1, unlimited)=w1187, name (unnamed)="back", element data type=w1186) -> (queue out=w1178:refnum<queue>)  [unwired: 2 in, 2 out]
          }
          event "Ratiometric?": Value Change {
            n923 = event-data() -> ("NewVal"=w1188:bool)  [unwired: 1 in, 5 out]
            n924 = case shown="True" w1188 {
              frame False {
                n925 = property on="Main Intensity" class="IntGraph (strict)"("ZScale.Maximum"=255.0 ("Z Scale.Range:Maximum"), "ZScale.Minimum"=0.0 ("Z Scale.Range:Minimum")) -> ()  [unwired: 2 in, 2 out]
              }
              frame True {
                n926 = local read "Dynamic Range"() -> (w1197:dbl)
                n927 = Add(x=1, y=w1197) -> (x+y=w1194:dbl)
                n928 = Subtract(x=1, y=w1197) -> (x-y=w1195:dbl)
                n929 = local write "loading ratiometric stack"(TRUE ("loading ratiometric stack")) -> ()
                n930 = property on="Main Intensity" class="IntGraph (strict)"("ZScale.Maximum"=w1194, "ZScale.Minimum"=w1195) -> ()  [unwired: 2 in, 2 out]
              }
            }
          }
        }
        n931 = local read "rt"() -> (w906:dbl)
        n932 = Add(x=w906, y=0.1) -> (x+y=w905:dbl)
        n933 = Greater?(x=w904, y=w905) -> (0:w903:bool)
        n934 = local read "Frame Rate (hz)"() -> (w891:dbl)
        n935 = case shown="True" w903 {
          tunnel: w902 -> [_ w916]
          tunnel: w901 -> [_ w930]
          frame False {
          }
          frame True {
            n936 = call <vilib>:"High Resolution Relative Seconds.vi"() -> ("relative seconds"=w929:dbl)
            n937 = local write "rt"(w929) -> ()
            n938 = call <vilib>:"Histogram.vi"("intervals"=256 ("# bins"), "X"=w930) -> ("Histogram Graph"=→"Histogram Graph 2":T5)  [unwired: 6 in, 3 out]
            n939 = disable-structure shown="Disabled" {
              frame Disabled {
                n940 = Transpose 2D Array() -> ()  [unwired: 1 in, 1 out]
              }
              frame Enabled {
              }
            }
            n941 = local read "X"() -> (w918:dbl)
            n942 = Divide(x=w918, y=2.0) -> (x/y=w917:dbl)
            n943 = Index Array(array=w916, index (row)=w917) -> (element=w922:u8[])  [unwired: 1 in]
            n944 = Decrement(x=w918) -> (x-1=w919:dbl)
            n945 = Initialize Array(0.0 ("element"), 1 ("dimension size")) -> (w926:dbl[])
            n946 = for {
              N: w919 -> [_]
              shift-right: [w932] -> w924
              shift-left: w926 -> [w933]
              i -> [w931]
              n947 = Build Array (concatenate)(w933, w931) -> (w932:dbl[])
            }
            n948 = Bundle(w924, "element"=w922) -> (→"XY Graph 2":cluster{dbl[], "element":u8[]})  [unwired: 1 in]
            "raw feed" <- w916
          }
        }
        n949 = Less?(x=w891, y=200.0) -> (x < y?=→"frame rate warning":bool)
        n950 = local read "stop"() -> (w909:bool)
        n951 = Get Queue Status(queue=w899) -> (# elements in queue=→"# elements in queue":i32)  [unwired: 2 in, 7 out]
      }
      n952 = while {
        tunnel: w401 -> [w1199]
        stop <- w1201 stop-if-true
        # "VIDEO / IMAGE SAVING LOOP"
        n953 = event shown="[0] Timeout" {
          selector: _ -> [_ _ _]
          dyn-events: _ -> [_ _ _]
          timeout: 1 -> [_ _ _]
          tunnel: w1199 -> [w1202 _ _]
          event Timeout {
            n954 = event-data() -> ()  [unwired: 1 in, 3 out]
            n955 = local read "Record Step"() -> (w1203:u8)
            n956 = case shown="1" w1203 {
              tunnel: w1202 -> [_ _ w1342 _]
              frame 0, Default {
                # "Do Nothing"
                n957 = local write "yellow"(FALSE ("yellow")) -> ()
                n958 = local write "red"(FALSE ("red")) -> ()
              }
              frame 1 {
                w1236 = "\r"
                w1252 = "\r"
                w1249 = "_"
                (unwired) "\\VIDEOS\\"
                # "Initialize Files"
                n959 = local read "FOV (um)"() -> (w1254:dbl)
                n960 = local read "Experiment Name"() -> (w1272:string)
                n961 = local read "Experiment Name"() -> (w1257:string)
                n962 = Get Date/Time String() -> (date string=w1269:string, time string=w1271:string)  [unwired: 3 in]
                n963 = Get Date/Time In Seconds() -> (seconds since 1Jan1904=w1260:timestamp)
                n964 = property on="RECORD / STOP VIDEO" class="Bool (strict)"("BoolText.Text"="Stop Recording" ("Boolean Text.Text"), "BoolText.FontBold"=TRUE ("Boolean Text.Font:Bold")) -> ()  [unwired: 2 in, 2 out]
                n965 = local read "Y"() -> (w1255:dbl)
                n966 = local read "Laser Power"() -> (w1243:dbl)
                n967 = local read "FOV (um)"() -> (w1242:dbl)
                n968 = local read "Date"() -> (w1256:string)
                n969 = Number To Decimal String(number=w1254) -> (decimal integer string=w1262:string)  [unwired: 1 in]
                n970 = Number To Decimal String(number=w1255) -> (decimal integer string=w1263:string)  [unwired: 1 in]
                n971 = Format Date/Time String(time format string (%c)="%Y-%m-%d", seconds (now)=w1260) -> (date/time string=w1259:string)  [unwired: 1 in]
                n972 = local read "Base Path"() -> (w1253:path)
                n973 = local read "Camera Status"() -> (w1266:string)
                n974 = Number To Decimal String(number=w1243) -> (decimal integer string=w1240:string)  [unwired: 1 in]
                n975 = Format Date/Time String(time format string (%c)="%H-%M-%S", seconds (now)=w1260) -> (date/time string=w1261:string)  [unwired: 1 in]
                n976 = Number To Decimal String(number=w1242) -> (decimal integer string=w1238:string)  [unwired: 1 in]
                n977 = call <vilib>:"Space Constant.vi"() -> ("String"=w1270:string)
                n978 = Concatenate Strings(w1262, w1249, w1263, w1249) -> (w1235:string)
                n979 = Concatenate Strings(w1256, w1257) -> (w1258:string)
                n980 = Concatenate Strings(w1252, w1252, w1252, w1269, w1270, w1271, w1270, "Recording Experiment Video..." ("string"), w1252, "Experiment Name: " ("string"), w1272, w1252) -> (w1268:string)
                n981 = Concatenate Strings(w1259, "_", w1261) -> (w1212:string)
                n982 = Build Path(base path=w1253, name or relative path=w1258) -> (appended path=w1211:path)
                n983 = Concatenate Strings(w1236, "Laser Power (mW): ", w1240, w1236, "Field of View (um): ", w1238, w1236) -> (w1237:string)
                n984 = Concatenate Strings(w1268, w1252, w1266, w1252, w1237) -> (w1265:string)
                n985 = local write "Experiment Log"(w1265) -> ()
                n986 = local read "Save Raw Binary"() -> (w1264:bool)
                n987 = disable-structure shown="Disabled" {
                  disable-tunnel: w1235 -> [w1280 _]
                  disable-tunnel: w1211 -> [w1279 _]
                  disable-tunnel: w1212 -> [w1278 _]
                  frame Disabled {
                    n988 = local read "Save Feed Binary"() -> (w1277:bool)
                    n989 = case shown="True" w1277 {
                      tunnel: w1279 -> [_ w1288]
                      tunnel: w1278 -> [_ w1285]
                      tunnel: w1280 -> [_ w1284]
                      frame False {
                      }
                      frame True {
                        # "Initialize feed video binary file"
                        n990 = Concatenate Strings(w1285, "_feed_" ("string"), w1284, ".bin" ("name or relative path")) -> (w1287:string)
                        n991 = Build Path(base path=w1288, name or relative path=w1287) -> (appended path=w1283:path)
                        n992 = Path To String(path=w1283) -> (string=w1281:string)
                        n993 = call <vilib>:"Create File and Containing Folders.vi"("file path"=w1283) -> ("refnum out"=→"Feed binfile refnum":refnum<file>)  [unwired: 9 in, 1 out]
                        n994 = local write "feed file path"(w1281) -> ()
                      }
                    }
                  }
                  frame Enabled {
                  }
                }
                n995 = property on="Save Raw Binary" class="Bool (strict)"("DisabledEnum"=T9."Disabled and Grayed Out" ("Disabled")) -> ()  [unwired: 2 in, 2 out]
                n996 = property on="Save Feed Binary" class="Bool (strict)"("DisabledEnum"=T9."Disabled and Grayed Out" ("Disabled")) -> ()  [unwired: 2 in, 2 out]
                n997 = local read "Record Step"() -> (w1245:u8)
                n998 = case shown="True" w1264 {
                  tunnel: w1211 -> [_ w1298]
                  tunnel: w1212 -> [_ w1297]
                  tunnel: w1235 -> [_ w1296]
                  frame False {
                  }
                  frame True {
                    # "Initialize raw video binary file"
                    n999 = Concatenate Strings(w1297, "_raw_" ("string"), w1296, ".bin" ("name or relative path")) -> (w1293:string)
                    n1000 = Build Path(base path=w1298, name or relative path=w1293) -> (appended path=w1290:path)
                    n1001 = Path To String(path=w1290) -> (string=w1292:string)
                    n1002 = call <vilib>:"Create File and Containing Folders.vi"("file path"=w1290) -> ("refnum out"=→"Raw binfile refnum":refnum<file>)  [unwired: 9 in, 1 out]
                    n1003 = local write "raw file path"(w1292) -> ()
                  }
                }
                n1004 = Increment(x=w1245) -> (x+1=w1244:u8)
                n1005 = local write "Record Step"(w1244) -> ()
                n1006 = property on="2x binning" class="Bool (strict)"("DisabledEnum"=T9."Disabled and Grayed Out" ("Disabled")) -> ()  [unwired: 2 in, 2 out]
                n1007 = Concatenate Strings(w1212, "_EPD voltage" ("string"), ".txt" ("name or relative path")) -> (w1217:string)
                n1008 = property on="Camera pixels" class="CmbBox"("DisabledEnum"=T9."Disabled and Grayed Out" ("Disabled")) -> ()  [unwired: 2 in, 2 out]
                n1009 = Concatenate Strings(w1212, "_laser mW" ("string"), ".txt" ("name or relative path")) -> (w1232:string)
                n1010 = Concatenate Strings(w1212, "_all voltage data" ("string"), ".csv" ("name or relative path")) -> (w1221:string)
                n1011 = Concatenate Strings(w1212, "_laser volts" ("string"), ".txt" ("name or relative path")) -> (w1227:string)
                n1012 = Build Path(base path=w1211, name or relative path=w1217) -> (appended path=w1216:path)
                n1013 = Build Path(base path=w1211, name or relative path=w1232) -> (appended path=w1226:path)
                n1014 = Build Path(base path=w1211, name or relative path=w1221) -> (appended path=w1222:path)
                n1015 = Build Path(base path=w1211, name or relative path=w1227) -> (appended path=w1225:path)
                n1016 = Path To String(path=w1216) -> (string=w1214:string)
                n1017 = call <vilib>:"Create File and Containing Folders.vi"("file path"=w1216) -> ("refnum out"=→"EPD Voltage Log refnum":refnum<file>)  [unwired: 9 in, 1 out]
                n1018 = call <vilib>:"Create File and Containing Folders.vi"("file path"=w1226) -> ("refnum out"=→"Laser mW renum":refnum<file>)  [unwired: 9 in, 1 out]
                n1019 = Concatenate Strings("EPD Voltage (V), Laser Voltage (V), Exposure Time (us), Pixels, AOBD Volts (V)" ("string"), "\r\n") -> (w1210:string)
                n1020 = local write "Voltage Log file Path"(w1214) -> ()
                n1021 = call <vilib>:"Create File and Containing Folders.vi"("file path"=w1222) -> ("refnum out"=w1207:refnum<file>)  [unwired: 9 in, 1 out]
                n1022 = call <vilib>:"Create File and Containing Folders.vi"("file path"=w1225) -> ("refnum out"=→"laer volts refnum":refnum<file>)  [unwired: 9 in, 1 out]
                n1023 = call <vilib>:"High Resolution Relative Seconds.vi"() -> ("relative seconds"=→"record start time":dbl)
                n1024 = Write to Text File(file (use dialog)=w1207, text=w1210) -> (refnum out=→"All data log refnum":refnum<file>)  [unwired: 2 in, 2 out]
              }
              frame 2 {
                w1304 = ","
                # "Stream Data to Binary File"
                n1025 = call <extravilib>:"Read.vi"("channel"=w1342) -> ("element"=w1334:u8[], "element valid?"=w1335:bool)  [unwired: 6 in, 3 out]
                n1026 = local read "Save Raw Binary"() -> (w1344:bool)
                n1027 = local read "minute"() -> (w1331:i32)
                n1028 = And(x=w1344, y=w1335) -> (x .and. y?=w1343:bool)
                n1029 = Greater Or Equal?(x=w1331, y=2.0) -> (x >= y?=→"yellow":bool)
                n1030 = Greater Or Equal?(x=w1331, y=5.0) -> (x >= y?=→"red":bool)
                n1031 = local read "EPD Voltage Log refnum"() -> (w1321:refnum<file>)
                n1032 = case shown="True" w1343 {
                  tunnel: w1334 -> [_ w1354]
                  frame False {
                  }
                  frame True {
                    n1033 = local read "Raw binfile refnum"() -> (w1355:refnum<file>)
                    n1034 = Write to Binary File(file (use dialog)=w1355, data=w1354, 5:FALSE ("prepend array or string size? (T)")) -> ()  [unwired: 3 in, 3 out]
                  }
                }
                n1035 = local read "laer volts refnum"() -> (w1323:refnum<file>)
                n1036 = local read "EPD Voltage"() -> (w1319:dbl)
                n1037 = local read "Laser Volts (V)"() -> (w1322:dbl)
                n1038 = Number To Fractional String(number=w1319, precision (6)=i16 2 ("width (-)")) -> (F-format string=w1320:string)  [unwired: 2 in]
                n1039 = Number To Fractional String(number=w1322, precision (6)=i16 2 ("width (-)")) -> (F-format string=w1327:string)  [unwired: 2 in]
                n1040 = Concatenate Strings(w1320, ",", "\r\n") -> (w1315:string)
                n1041 = Concatenate Strings(w1327, ",", "\r\n") -> (w1328:string)
                n1042 = call <vilib>:"High Resolution Relative Seconds.vi"() -> ("relative seconds"=w1341:dbl)
                n1043 = local read "record start time"() -> (w1340:dbl)
                n1044 = Write to Text File(file (use dialog)=w1321, text=w1315) -> ()  [unwired: 2 in, 3 out]
                n1045 = Write to Text File(file (use dialog)=w1323, text=w1328) -> ()  [unwired: 2 in, 3 out]
                n1046 = Subtract(x=w1341, y=w1340) -> (x-y=w1339:dbl)
                n1047 = Seconds To Date/Time(time stamp (now)=w1339) -> (date time rec=w1338:T15)  [unwired: 1 in]
                n1048 = local read "Laser Volts (V)"() -> (w1300:dbl)
                n1049 = local read "Laser On/Off"() -> (w1301:bool)
                n1050 = local read "Laser Zoom Level"() -> (w1305:T3)
                n1051 = local read "Exposure Time (us)"() -> (w1308:dbl)
                n1052 = Unbundle By Name(w1338) -> ("second"=→"second":i32, "minute"=→"minute":i32)  [unwired: 5 out]
                n1053 = local read "EPD Voltage"() -> (w1311:dbl)
                n1054 = local read "All data log refnum"() -> (w1313:refnum<file>)
                n1055 = local read "Camera pixels"() -> (w1306:string)
                n1056 = case shown="True" w1301 {
                  tunnel: w1300 -> [_ w1348]
                  tunnel: ["0.0000" w1346] -> w1299
                  frame False {
                  }
                  frame True {
                    n1057 = Number To Fractional String(number=w1348, precision (6)=i16 4 ("width (-)")) -> (F-format string=w1346:string)  [unwired: 2 in]
                  }
                }
                n1058 = Number To Fractional String(number=w1311, precision (6)=i16 2) -> (F-format string=w1310:string)  [unwired: 2 in]
                n1059 = Number To Fractional String(number=w1308, precision (6)=i16 4 ("width (-)")) -> (F-format string=w1307:string)  [unwired: 2 in]
                n1060 = case shown="\"Radio Selection 5\"" w1305 {
                  tunnel: ["1 mV" "0.6 V" "1.2 V" "2.4 V" "3.6 V"] -> w1303
                  frame "Radio Selection 1" {
                  }
                  frame "Radio Selection 2" {
                  }
                  frame "Radio Selection 3" {
                  }
                  frame "Radio Selection 4" {
                  }
                  frame "Radio Selection 5" {
                  }
                }
                n1061 = Concatenate Strings(w1310, w1304, w1299, w1304, w1307, w1304, w1306, w1304, w1303, "\r\n") -> (w1314:string)
                n1062 = Write to Text File(file (use dialog)=w1313, text=w1314) -> ()  [unwired: 2 in, 3 out]
              }
              frame 3 {
                # "Close Files"
                n1063 = local read "EPD Voltage Log refnum"() -> (w1362:refnum<file>)
                n1064 = local read "Laser mW renum"() -> (w1364:refnum<file>)
                n1065 = local read "All data log refnum"() -> (w1361:refnum<file>)
                n1066 = local read "laer volts refnum"() -> (w1363:refnum<file>)
                n1067 = flat-sequence {
                  tunnel: [w1390] -> w1360
                  tunnel: w1357 -> [w1384]
                  tunnel: w1360 -> [w1438]
                  frame #0 {
                    w1373 = "\r"
                    w1389 = "\r"
                    w1386 = "\r"
                    # "write final video time to experimental log"
                    n1068 = local read "Partial P. Ref."() -> (w1423:string)
                    n1069 = local read "Coverslip"() -> (w1425:string)
                    n1070 = local read "Material"() -> (w1421:string)
                    n1071 = local read "conc."() -> (w1417:string)
                    n1072 = local read "Size"() -> (w1419:string)
                    n1073 = local read "pH"() -> (w1415:string)
                    n1074 = Number To Fractional String(number=w1384, precision (6)=i16 4) -> (F-format string=w1432:string)  [unwired: 2 in]
                    n1075 = Concatenate Strings(w1386, "EXPERIMENT TIME", w1386, "Video Duration: ", w1432, " Seconds", w1386, w1386) -> (w1383:string)
                    n1076 = Concatenate Strings("COVERSLIP AND SAMPLE INFO", w1389, "Coverslip: ", w1425, w1389, "Partial Reflector: ", w1423, w1389, "Material: ", w1421, w1389, "Size: ", w1419, w1389, "Concentration: ", w1417, w1389, "pH: ", w1415, w1389, w1389) -> (w1382:string)
                    n1077 = local read "Laser Zoom Level"() -> (w1379:T3)
                    n1078 = local read "Exposure Time (us)"() -> (w1376:dbl)
                    n1079 = local read "EPD Voltage set"() -> (w1397:dbl)
                    n1080 = local read "Experiment Notes"() -> (w1381:string)
                    n1081 = local read "Laser Volts (V)"() -> (w1396:dbl)
                    n1082 = local read "nm/pixel\n(binned)"() -> (w1402:dbl)
                    n1083 = local read "FOV (um)"() -> (w1398:dbl)
                    n1084 = local read "Camera pixels"() -> (w1406:string)
                    n1085 = local read "2x binning"() -> (w1412:bool)
                    n1086 = Number To Decimal String(number=w1397, width (-)=i16 5) -> (decimal integer string=w1391:string)
                    n1087 = Number To Decimal String(number=w1398, width (-)=i16 5) -> (decimal integer string=w1399:string)
                    n1088 = Number To Decimal String(number=w1396, width (-)=i16 5) -> (decimal integer string=w1393:string)
                    n1089 = Number To Decimal String(number=w1376, width (-)=i16 5) -> (decimal integer string=w1374:string)
                    n1090 = case shown="\"Radio Selection 5\"" w1379 {
                      tunnel: ["1 mV" "0.6 V" "1.2 V" "2.4 V" "3.6 V"] -> w1378
                      frame "Radio Selection 1" {
                      }
                      frame "Radio Selection 2" {
                      }
                      frame "Radio Selection 3" {
                      }
                      frame "Radio Selection 4" {
                      }
                      frame "Radio Selection 5" {
                      }
                    }
                    n1091 = local read "Experiment Log"() -> (w1428:string)
                    n1092 = Select(t="2x", s=w1412, f="1x") -> (s? t:f=w1404:string)
                    n1093 = Number To Decimal String(number=w1402, width (-)=i16 5) -> (decimal integer string=w1401:string)
                    n1094 = Concatenate Strings(w1373, "EXPERIMENT SPECIFICATIONS", w1373, "Pixels: ", w1406, w1373, "Binning: ", w1404, w1373, "nm/pixel: ", w1401, w1373, "FOV (um): ", w1399, w1373, "AOBD amplitude: ", w1378, w1373, "Laser Volts: ", w1393, w1373, "EPD volts: ", w1391, w1373, "Exposure time", w1373, w1374, w1373) -> (w1385:string)
                    n1095 = Concatenate Strings(w1385, w1383, w1382, w1381) -> (w1390:string)
                    n1096 = Concatenate Strings(w1428, w1390) -> (w1427:string)
                    n1097 = local write "Experiment Log"(w1427) -> ()
                  }
                  frame #1 {
                    # "Write text file"
                    # "copy everything from experimental log to a text file"
                    n1098 = local read "Experiment Name"() -> (w1444:string)
                    n1099 = local read "Date"() -> (w1443:string)
                    n1100 = local read "Raw binfile refnum"() -> (w1453:refnum<file>)
                    n1101 = Refnum to Path(1:w1453) -> (0:w1452:path)
                    n1102 = Strip Path(path=w1452) -> (name=w1454:string)  [unwired: 1 out]
                    n1103 = local read "Base Path"() -> (w1442:path)
                    n1104 = Concatenate Strings(w1443, w1444) -> (w1445:string)
                    n1105 = String Subset(string=w1454, length (rest)=19 ("length (rest)")) -> (substring=w1451:string)  [unwired: 1 in]
                    n1106 = Build Path(base path=w1442, name or relative path=w1445) -> (appended path=w1441:path)
                    n1107 = Concatenate Strings(w1451, "_Experiment Notes.txt" ("name or relative path")) -> (w1450:string)
                    n1108 = Build Path(base path=w1441, name or relative path=w1450) -> (appended path=w1448:path)
                    n1109 = call <vilib>:"Create File and Containing Folders.vi"("file path"=w1448) -> ("refnum out"=w1449:refnum<file>)  [unwired: 9 in, 1 out]
                    "Text File refnum" <- w1449
                    n1110 = Path To String(path=w1448) -> (string=w1447:string)
                    n1111 = Write to Text File(file (use dialog)=w1449, text=w1438) -> (refnum out=w1446:refnum<file>)  [unwired: 2 in, 2 out]
                    n1112 = local write "text file path"(w1447) -> ()
                    n1113 = Close File(refnum=w1446) -> ()  [unwired: 1 in, 2 out]
                  }
                }
                n1114 = local read "record start time"() -> (w1359:dbl)
                n1115 = call <vilib>:"High Resolution Relative Seconds.vi"() -> ("relative seconds"=w1358:dbl)
                n1116 = Subtract(x=w1358, y=w1359) -> (x-y=w1357:dbl)
                n1117 = Close File(refnum=w1361) -> ()  [unwired: 1 in, 2 out]
                n1118 = Close File(refnum=w1362) -> ()  [unwired: 1 in, 2 out]
                n1119 = Close File(refnum=w1364) -> ()  [unwired: 1 in, 2 out]
                n1120 = Close File(refnum=w1363) -> ()  [unwired: 1 in, 2 out]
                n1121 = local read "Save Raw Binary"() -> (w1372:bool)
                n1122 = property on="RECORD / STOP VIDEO" class="Bool (strict)"("BoolText.Text"="Record Video" ("Boolean Text.Text"), "BoolText.FontBold"=FALSE ("Boolean Text.Font:Bold")) -> ()  [unwired: 2 in, 2 out]
                n1123 = case shown="True" w1372 {
                  tunnel: w1357 -> [_ w1466]
                  frame False {
                  }
                  frame True {
                    w1474 = "\r"
                    n1124 = local read "Raw binfile refnum"() -> (w1477:refnum<file>)
                    n1125 = local read "Experiment Log"() -> (w1476:string)
                    n1126 = local read "Y"() -> (w1471:dbl)
                    n1127 = local read "X"() -> (w1472:dbl)
                    n1128 = Close File(refnum=w1477) -> (path=w1455:path)  [unwired: 1 in, 1 out]
                    n1129 = Multiply(x=w1472, y=w1471) -> (x*y=w1470:dbl)
                    n1130 = Concatenate Strings(w1476, w1474, "Saved Raw Binary File", w1474) -> (w1475:string)
                    n1131 = Strip Path(path=w1455) -> (stripped path=w1459:path, name=w1464:string)
                    n1132 = Get File Size(file=w1455) -> (size (in bytes)=w1469:i64)  [unwired: 1 in, 2 out]
                    n1133 = local write "Experiment Log"(w1475) -> ()
                    n1134 = Divide(x=w1469, y=w1470) -> (x/y=w1468:dbl)
                    n1135 = Divide(x=w1468, y=w1466) -> (x/y=w1467:dbl)
                    n1136 = Round To Nearest(number=w1467) -> (nearest integer value=w1465:dbl)
                    "recorded fps" <- w1465
                    n1137 = Number To Decimal String(number=w1465) -> (decimal integer string=w1461:string)  [unwired: 1 in]
                    n1138 = Concatenate Strings(w1461, "." ("string")) -> (w1460:string)
                    n1139 = Search and Replace String(input string=w1464, search string=".", replace string=w1460) -> (result string=w1458:string)  [unwired: 5 in, 3 out]
                    n1140 = String To Path(string=w1458) -> (path=w1457:path)
                    n1141 = Build Path(base path=w1459, name or relative path=w1457) -> (appended path=w1456:path)
                    n1142 = Move(source path=w1455, 10:w1456) -> ()  [unwired: 3 in, 3 out]
                  }
                }
                n1143 = property on="Save Raw Binary" class="Bool (strict)"("DisabledEnum"=T9."Enabled" ("Disabled")) -> ()  [unwired: 2 in, 2 out]
                n1144 = property on="Save Feed Binary" class="Bool (strict)"("DisabledEnum"=T9."Enabled" ("Disabled")) -> ()  [unwired: 2 in, 2 out]
                n1145 = local write "Record Step"(u8 0 ("Record Step")) -> ()
                n1146 = property on="2x binning" class="Bool (strict)"("DisabledEnum"=T9."Enabled" ("Disabled")) -> ()  [unwired: 2 in, 2 out]
                n1147 = property on="Camera pixels" class="CmbBox"("DisabledEnum"=T9."Enabled" ("Disabled")) -> ()  [unwired: 2 in, 2 out]
              }
            }
          }
          event "SAVE RAW IMAGE": Value Change {
            n1148 = event-data() -> ()  [unwired: 1 in, 6 out]
            n1149 = flat-sequence {
              frame #0 {
                w1483 = "_"
                n1150 = local read "Experiment Name"() -> (w1496:string)
                n1151 = local read "raw feed"() -> (w1478:u8[][])
                n1152 = local read "Date"() -> (w1495:string)
                n1153 = Get Date/Time In Seconds() -> (seconds since 1Jan1904=w1489:timestamp)
                n1154 = Format Date/Time String(time format string (%c)="%Y-%m-%d", seconds (now)=w1489) -> (date/time string=w1490:string)  [unwired: 1 in]
                n1155 = Concatenate Strings(w1495, w1496, "\\IMAGES\\") -> (w1498:string)
                n1156 = Format Date/Time String(time format string (%c)="%H-%M-%S", seconds (now)=w1489) -> (date/time string=w1484:string)  [unwired: 1 in]
                n1157 = local read "Base Path"() -> (w1494:path)
                n1158 = call "IMAQ Create"("Image Name"="temp save") -> ("New Image"=w1480:T1)  [unwired: 4 in, 1 out]
                n1159 = Concatenate Strings(w1490, w1483, "image" ("string"), w1483, w1484, ".png" ("name or relative path")) -> (w1493:string)
                n1160 = Build Path(base path=w1494, name or relative path=w1498) -> (appended path=w1488:path)
                n1161 = call "IMAQ ArrayToImage"("Image Pixels (U8)"=w1478, "Image"=w1480) -> ("Image Out"=w1481:T1)  [unwired: 8 in, 1 out]
                n1162 = Build Path(base path=w1488, name or relative path=w1493) -> (appended path=w1487:path)
                n1163 = call <vilib>:"Create File and Containing Folders.vi"("file path"=w1487) -> ()  [unwired: 9 in, 2 out]
                n1164 = Path To String(path=w1487) -> (string=w1492:string)
                n1165 = call-poly "IMAQ Write File 2"("File Path"=w1487, "Image"=w1481) -> ()  [unwired: 8 in, 2 out]
                n1166 = local write "image file path"(w1492) -> ()
              }
              frame #1 {
                n1167 = local write "SAVE RAW IMAGE"(FALSE ("SAVE IMAGE")) -> ()
                n1168 = Wait (ms)(milliseconds to wait=u32 1000) -> ()  [unwired: 1 out]
              }
            }
          }
          event "RECORD / STOP VIDEO": Value Change {
            n1169 = event-data() -> ()  [unwired: 1 in, 6 out]
            n1170 = local read "Record Step"() -> (w1502:u8)
            n1171 = Increment(x=w1502) -> (x+1=w1501:u8)
            n1172 = local write "Record Step"(w1501) -> ()
          }
        }
        n1173 = local read "stop"() -> (w1201:bool)
      }
      n1174 = disable-structure shown="Disabled" {
        frame Disabled {
          n1175 = while {
            stop <- w606 stop-if-true
            # "GREEN GEM LASER CONTROLS"
            n1176 = local read "Laser Status Update Timer"() -> (w605:u32)
            n1177 = Tick Count (ms)() -> (millisecond timer value=w601:u32)
            n1178 = Add(x=u32 1000, y=w605) -> (x+y=w603:u32)
            n1179 = Greater?(x=w601, y=w603) -> (0:w604:bool)
            n1180 = case "Refresh Laser Status" shown="True" w604 {
              frame False {
              }
              frame True {
                n1181 = Tick Count (ms)() -> (millisecond timer value=w625:u32)
                n1182 = local read "Laser COM Port"() -> (w624:refnum<visa-resource-name>)
                n1183 = local write "Laser Status Update Timer"(w625) -> ()
                n1184 = local read "Laser PSUType"() -> (w623:u16)
                n1185 = call "GetCurrent.vi"("LQComm Resource In"=w624, "PSUType"=w623) -> ("CurrentValue"=w616:dbl, "LQComm Resource Out"=w622:refnum<visa-resource-name>)  [unwired: 1 in, 2 out]
                n1186 = local write "Laser Current"(w616) -> ()
                n1187 = call "GetLaserTemperature.vi"("LQCommResourceIn"=w622) -> ("LQComm Resource Out"=w621:refnum<visa-resource-name>, "LaserTemperatureValue"=w619:dbl)  [unwired: 2 in, 2 out]
                n1188 = local write "Laser Temp"(w619) -> ()
                n1189 = call "GetPower.vi"("LQComm Resource In"=w621) -> ("PowerValue"=w617:dbl, "LQComm Resource Out"=w620:refnum<visa-resource-name>)  [unwired: 2 in, 2 out]
                n1190 = local write "Laser Power"(w617) -> ()
                n1191 = call "GetPSUTemp.vi"("LQCommResourceIn"=w620) -> ("PSUTemperatureValue"=w618:dbl)  [unwired: 2 in, 3 out]
                n1192 = local write "PSU Temp"(w618) -> ()
              }
            }
            n1193 = event shown="[1] \"Set Laser Power\", \"Set Power (mW)\": Value Change" {
              selector: _ -> [_ _ _]
              dyn-events: _ -> [_ _ _]
              timeout: 10 -> [_ _ _]
              event Timeout {
                n1194 = event-data() -> ()  [unwired: 1 in, 3 out]
              }
              event "Set Laser Power", "Set Power (mW)": Value Change {
                n1195 = event-data() -> ()  [unwired: 1 in, 6 out]
                n1196 = local read "Laser COM Port"() -> (w610:refnum<visa-resource-name>)
                n1197 = local read "Set Power (mW)"() -> (w608:dbl)
                n1198 = local read "Laser PSUType"() -> (w609:u16)
                n1199 = call "SetPower.vi"("NewPower"=w608, "PSUType"=w609, "LQCommResourceIn"=w610) -> ()  [unwired: 1 in, 3 out]
                n1200 = local write "Set Laser Power"(FALSE ("Set Laser Power")) -> ()
              }
              event "Green Laser": Value Change {
                n1201 = event-data() -> ("NewVal"=w611:bool)  [unwired: 1 in, 5 out]
                n1202 = case shown="False" w611 {
                  frame False {
                    n1203 = local read "Laser COM Port"() -> (w613:refnum<visa-resource-name>)
                    n1204 = local read "Laser PSUType"() -> (w612:u16)
                    n1205 = call "TurnOFF.vi"("PSUType"=w612, "LQCommResourceIn"=w613) -> ()  [unwired: 1 in, 3 out]
                  }
                  frame True {
                    n1206 = local read "Laser COM Port"() -> (w615:refnum<visa-resource-name>)
                    n1207 = local read "Laser PSUType"() -> (w614:u16)
                    n1208 = call "TurnON.vi"("PSUType"=w614, "LQCommResourceIn"=w615) -> ()  [unwired: 1 in, 3 out]
                  }
                }
              }
            }
            n1209 = local read "stop"() -> (w606:bool)
          }
        }
        frame Enabled {
        }
      }
      n1210 = while {
        tunnel: w377 -> [w560]
        tunnel: w376 -> [w559]
        tunnel: [w558] -> w375
        stop <- w561 stop-if-true
        n1211 = event shown="[2] \"Laser Volts (V)\": Value Change" {
          selector: _ -> [_ _ _]
          dyn-events: _ -> [_ _ _]
          timeout: 10 -> [_ _ _]
          tunnel: w560 -> [_ w570 w575]
          tunnel: w559 -> [w563 w565 w572]
          tunnel: [w563 w564 w571] -> w558
          event Timeout {
            n1212 = event-data() -> ()  [unwired: 1 in, 3 out]
          }
          event "Laser On/Off": Value Change {
            w567 = u16 0 items=["V", "mV", "kV", "A", "mA"] ("Unit(V)")
            w569 = u16 0 items=["Voltage", "Current"] ("Function(0:Voltage)")
            n1213 = event-data() -> ("NewVal"=w568:bool)  [unwired: 1 in, 5 out]
            n1214 = local read "Laser Volts (V)"() -> (w566:dbl)
            n1215 = call "Configure Output.vi"("VISA resource name"=w570, "Manual Range(0.00)"=w566, "Function(0:Voltage)"=w569, "Enable Output (T: Enable)"=w568, "error in (no error)"=w565, "Unit(V)"=w567) -> ("error out"=w564:errorcluster)  [unwired: 8 in, 1 out]
          }
          event "Laser Volts (V)": Value Change {
            n1216 = event-data() -> ("NewVal"=w573:dbl)  [unwired: 1 in, 5 out]
            n1217 = Greater?(x=w573, y="V limit") -> (0:w576:bool)
            n1218 = case shown="False" w576 {
              tunnel: w575 -> [w580 w594]
              tunnel: w573 -> [w579 _]
              tunnel: w572 -> [w578 w592]
              tunnel: [w577 w591] -> w571
              frame False {
                n1219 = property on="Laser On/Off" class="Bool (strict)"("DisabledEnum"=T9."Enabled" ("Disabled")) -> ()  [unwired: 2 in, 2 out]
                n1220 = local read "Laser On/Off"() -> (w581:bool)
                n1221 = case shown="False" w581 {
                  tunnel: w580 -> [_ w590]
                  tunnel: w579 -> [_ w589]
                  tunnel: w578 -> [w583 w585]
                  tunnel: [w583 w584] -> w577
                  frame False {
                  }
                  frame True {
                    w586 = u16 0 items=["V", "mV", "kV", "A", "mA"] ("Unit(V)")
                    w588 = u16 0 items=["Voltage", "Current"] ("Function(0:Voltage)")
                    n1222 = call "Configure Output.vi"("VISA resource name"=w590, "Manual Range(0.00)"=w589, "Function(0:Voltage)"=w588, "Enable Output (T: Enable)"=TRUE, "error in (no error)"=w585, "Unit(V)"=w586) -> ("error out"=w584:errorcluster)  [unwired: 8 in, 1 out]
                  }
                }
              }
              frame True {
                w596 = u16 0 items=["V", "mV", "kV", "A", "mA"] ("Unit(V)")
                w597 = u16 0 items=["Voltage", "Current"] ("Function(0:Voltage)")
                n1223 = call "Configure Output.vi"("VISA resource name"=w594, "Manual Range(0.00)"=0.0, "Function(0:Voltage)"=w597, "Enable Output (T: Enable)"=FALSE, "error in (no error)"=w592, "Unit(V)"=w596) -> ("error out"=w591:errorcluster)  [unwired: 8 in, 1 out]
                n1224 = local write "Laser On/Off"(FALSE ("Laser On/Off")) -> ()
                n1225 = property on="Laser On/Off" class="Bool (strict)"("DisabledEnum"=T9."Disabled and Grayed Out" ("Disabled")) -> ()  [unwired: 2 in, 2 out]
              }
            }
          }
        }
        n1226 = local read "stop"() -> (w561:bool)
      }
      "bg countdown" <- 0.0 ("bg countdown")
    }
    frame #3 {
      # "Close Everything"
      n1227 = call <vilib>:"DAQmx Stop Task.vi"("task/channels in"=w2003, "error in"=w1999) -> ("task out"=w2004:refnum<k21>, "error out"=w1998:errorcluster)  [unwired: 12 in]
      n1228 = call <vilib>:"Basic Function Generator.vi"("offset"=0.0, "signal type"=T2."Triangle Wave", "amplitude"=0.0, "frequency"=0.0) -> ("signal out"=w2008:waveform(dbl))  [unwired: 5 in, 2 out]
      n1229 = Flush Queue(queue=w2023) -> (queue out=w2025:refnum<queue>)  [unwired: 1 in, 2 out]
      n1230 = Flush Queue(queue=w2022) -> (queue out=w2024:refnum<queue>)  [unwired: 1 in, 2 out]
      n1231 = call <vilib>:"IMAQdx Stop Acquisition.vi"("error in"=w2034, "Session In"=w2027) -> ("error out"=w2033:errorcluster, "Session Out"=w2028:T8)  [unwired: 8 in]
      n1232 = Release Queue(queue=w2024) -> (error out=w2020:errorcluster)  [unwired: 2 in, 2 out]
      n1233 = Release Queue(queue=w2025) -> (error out=w2021:errorcluster)  [unwired: 2 in, 2 out]
      n1234 = disable-structure shown="Disabled" {
        disable-tunnel: w2015 -> [w2036 _]
        frame Disabled {
          n1235 = call <instrlib>:"Close.vi"("VISA resource name"=w2036) -> ()  [unwired: 10 in, 1 out]
        }
        frame Enabled {
        }
      }
      n1236 = call <vilib>:"IMAQdx Unconfigure Acquisition.vi"("error in"=w2033, "Session In"=w2028) -> ("error out"=w2032:errorcluster, "Session Out"=w2029:T8)  [unwired: 8 in]
      n1237 = for {
        tunnel: w2026 -> [w2038] mode=indexing
        tunnel: [w2037] -> w2030 mode=indexing
        n1238 = call "IMAQ Dispose"("Image"=w2038) -> ("error out"=w2037:errorcluster)  [unwired: 5 in]
      }
      n1239 = call <vilib>:"IMAQdx Close Camera.vi"("error in"=w2032, "Session In"=w2029) -> ("error out"=w2031:errorcluster)  [unwired: 9 in]
      n1240 = call-poly <vilib>:"DAQmx Write.vi"("task/channels in"=w2004, "data"=w2008, "error in"=w1998) -> ("task out"=w2007:refnum<k21>, "error out"=w1997:errorcluster)  [unwired: 10 in, 1 out]
      n1241 = call <vilib>:"DAQmx Stop Task.vi"("task/channels in"=w2013, "error in"=w2000) -> ("task out"=w2014:refnum<k21>, "error out"=w2001:errorcluster)  [unwired: 12 in]
      n1242 = call <vilib>:"DAQmx Start Task.vi"("task/channels in"=w2007, "error in"=w1997) -> ("task out"=w2006:refnum<k21>, "error out"=w1996:errorcluster)  [unwired: 12 in]
      n1243 = call <vilib>:"DAQmx Stop Task.vi"("task/channels in"=w2006, "error in"=w1996) -> ("task out"=w2005:refnum<k21>, "error out"=w1995:errorcluster)  [unwired: 12 in]
      n1244 = call <vilib>:"DAQmx Clear Task.vi"("task in"=w2014, "error in"=w2001) -> ("error out"=w1994:errorcluster)  [unwired: 13 in]
      n1245 = call <vilib>:"DAQmx Clear Task.vi"("task in"=w2005, "error in"=w1995) -> ("error out"=w1993:errorcluster)  [unwired: 13 in]
      n1246 = call <instrlib>:"Close.vi"("error in (no error)"=w1989, "VISA resource name"=w1990) -> ()  [unwired: 9 in, 1 out]
      n1247 = Merge Errors(w1993, w1994, w1991) -> (w1992:errorcluster)
      n1248 = Merge Errors(w2021, w2020, w2019, w2018, w2016, w1992) -> (w2017:errorcluster)
      n1249 = Merge Errors(w2030, w2031, w2017, w2002) -> (w2035:errorcluster)
      n1250 = call <vilib>:"Simple Error Handler.vi"("error in (no error)"=w2035) -> ()  [unwired: 4 in, 5 out]
    }
  }
